vi "Main 1.0.vi"() -> ()   [LabVIEW 2014]
doc: "This template is for the Queued Message Handler design pattern.\n\nThe Event Handling Loop generates messages based on user interface actions.\n\nThe Message Handling Loop processes messages generated by the Event Handling Loop, or by other messages. The messages are string values, so new messages can be added easily to the Message Cases case structure in the Message Handling Loop. Each message cluster can also provide an optional value for Message Data, which is a variant that can be converted to whatever message-specific data is required."
uses:
  Loops.ctl
  Digital/Digital Input Cluster.ctl
  Digital/Digital Output Cluster.ctl
  Laser/Keyence Status.ctl
  Analog/Analog Output Cluster.ctl
  Analog/Analog Input Cluster.ctl
  Analog/Analog Result Cluster.ctl
  Engine/Thread Flag Control.ctl
  Engine/Message.ctl
  Analog/Enum AO.ctl
  Data Processor/Data Processor cluster.ctl
  Data Processor/I Adj Parameters.ctl
  Data Processor/UCTRL Cluster.ctl
  <vilib>/Utility/miscctls.llb/LVRectTypeDef.ctl
  <vilib>/Utility/miscctls.llb/LVPointTypeDef.ctl
  Engine/Thread.ctl
  Teszt/Teszt.ctl
  Teszt/Command.ctl
  Laser/Keyence data cluster.ctl
  support/Message Queue/Enqueue Message (Single).vi
  support/Message Queue/Enqueue Message (Array).vi
  global/Global 1.vi
  <vilib>/Utility/error.llb/Error Cluster From Error Code.vi
  <vilib>/ErrorRing/Error Ring.xnode
  support/Message Queue/Message Queue.lvlib
  support/User Event - Stop/User Event - Stop.lvlib
panel:
  out "Digitális Óra":timestamp format="%<%H:%M:%S\n%x>T"
  out "Termék":string
  in  "Tab Control":T1(tab)=enum."Etalon"
  out "Gyûrû megnyomva":bool caption="JÓ"
  out "Termék behelyezve":bool caption="JÓ"
  out "Gyûrû behelyezve":bool caption="JÓ"
  in  "Reset_Counters 2":bool
  out "Rossz db 2":i32 caption="Rossz db"
  out "Jó db 2":i32 caption="Jó db"
  out "Állapot kijelzõ ring":string
  out "Rossz 3":bool caption="Rossz"
  out "JÓ 3":bool caption="JÓ"
  out "dU görbe":T2
  in  "Eredmény Listbox":i32(listbox)
  out "Állapot kijelzõ fõképernyõ":string
  out "Rossz 2":bool caption="Rossz"
  out "JÓ 2":bool caption="JÓ"
  in  "Mérés stop 2":bool
  in  "Mérés start 2":bool
  in  "Reset_Counters":bool
  out "Rossz db":i32
  out "Jó db":i32
  out "Felhasználó":string
  out "Jogosultság":string
  in  "Termék választás":bool
  in  "Kilépés":bool
  in  "Felhasználó váltás":bool
  in  "Karbantartás":bool
  in  "Stop":bool
  in  "Végig mér":bool
  in  "Mérés Folyamatos":bool
  in  "Mérés stop":bool
  in  "Mérés következõ":bool
  out "Állapot kijelzõ 2":string
  out "Rossz":bool
  out "JÓ":bool
  in  "Mérés Listbox":i32(listbox)
  in  "Mérés start":bool
  in  "Thread 1":bool
  in  "Thread 0":bool
  out "Thread Num":enum16{"Mérés", "Gyûrûzés"}(ring)
  in  "Teszt eltávolít":bool
  out "Tesztszekvencia neve":string="Nincs betöltve..."
  in  "Teszt szerkeszt":bool
  in  "Teszt hozzáad":bool
  in  "Teszt töröl":bool
  in  "Teszt módosít":bool
  in  "Teszt vektor listbox":i32(listbox)
  in  "Teszt másol":bool
  in  "Teszt beilleszt":bool
  in  "Teszt megnyit":bool
  in  "Teszt ment":bool
  out "Thread Num 2":enum16{"Mérés", "Gyûrûzés"}(ring)
  in  "Etalon mérés":bool=TRUE
  in  "Teszt eltávolít 2":bool
  out "Tesztszekvencia neve 2":string="Nincs betöltve..."
  in  "Teszt szerkeszt 2":bool
  in  "Teszt hozzáad 2":bool
  in  "Teszt töröl 2":bool
  in  "Teszt módosít 2":bool
  in  "Etalon listbox":i32(listbox)
  in  "Teszt másol 2":bool
  in  "Teszt beilleszt 2":bool
  in  "Teszt megnyit 2":bool
  in  "Teszt ment 2":bool
  in  "Thread 0_2":bool
  in  "Thread 1_2":bool
  in  "Tab control debug":enum32{"Digital IO", "Analog IO", "Laser"}(tab)
  out "Digital input":T3
  in  "Digital Out":T4
  in  "Setup UCTRL NTC":bool
  out "NI Analog Input":T5 {"NI-6221"."Uref" format="%_5f"; "NI-6221"."Temperature" format="%_5f"; "NI-6221"."Uisol" format="%_5f"; "NI-6221"."U48" format="%_5f"; "NI-6221"."U15" format="%_5f"; "NI-6221"."NTC" format="%_5f"; "NI-6221"."Sensor" format="%_5f"; "Analog Result"."Számolt NTC hõmérséklet" format="%.3g"; "Analog Result"."15V" format="%.3g"; "Analog Result"."Elvárt NTC ellenállás" format="%.3g"; "Analog Result"."48V" format="%.3g"; "Analog Result"."Hõmérséklet" format="%.3g"; "Analog Result"."Szigetelési ellenállás" format="%.3g"; "Analog Result"."NTC ellenállás" format="%.3g"; "Analog Result"."Szenzor ellenállás" format="%.3g"}
  in  "NI Analog Output":T7
  out "UCTRL NTC":dbl
  out "UCTRL R":dbl
  out "UCTRL dU":dbl
  in  "Setup UCTRL R":bool
  in  "Keyence Disable":bool caption="Lézer jelölés tiltása"
  in  "Update Sys Time":bool
  out "Communication opened":bool
  in  "Start marking":bool
  out "Status":T8
  in  "Program change":bool
  in  "Error clear":bool
  in  "Keyence Open":bool
  in  "Program No":dbl
  in  "Termék cluster array":T9[](array[typedef])
  in  "Termék ment":bool
  out "Aktuális termék":T9
  in  "Felhasználók mentés":bool
  in  "Jogosultságok array":T10[](array[typedef])
  in  "Felhasználók Listbox":i32(listbox)
  in  "Új felhasználó":bool
  in  "Felhasználó törlése":bool
  in  "Felhasználó módosítás":bool
  out "Loops":T11
  out "Állapot kijelzõ":string
  # "Termék:"
  # "686 EOL Teszter"
  # "GYÛRÛZÉS"
  # "MÉRÉS"
  # "Menü"
  # "Bejelentkezve:"
  # "Jogosultság:"
  # "Menü"
  # "Keyence lézer jelölõ"
  # "Aktuális termék:"
  # "Termékek felvétele/beállítása:"
  # "Menü"
  # "Felhasználók"
  # "Jogosultságok"
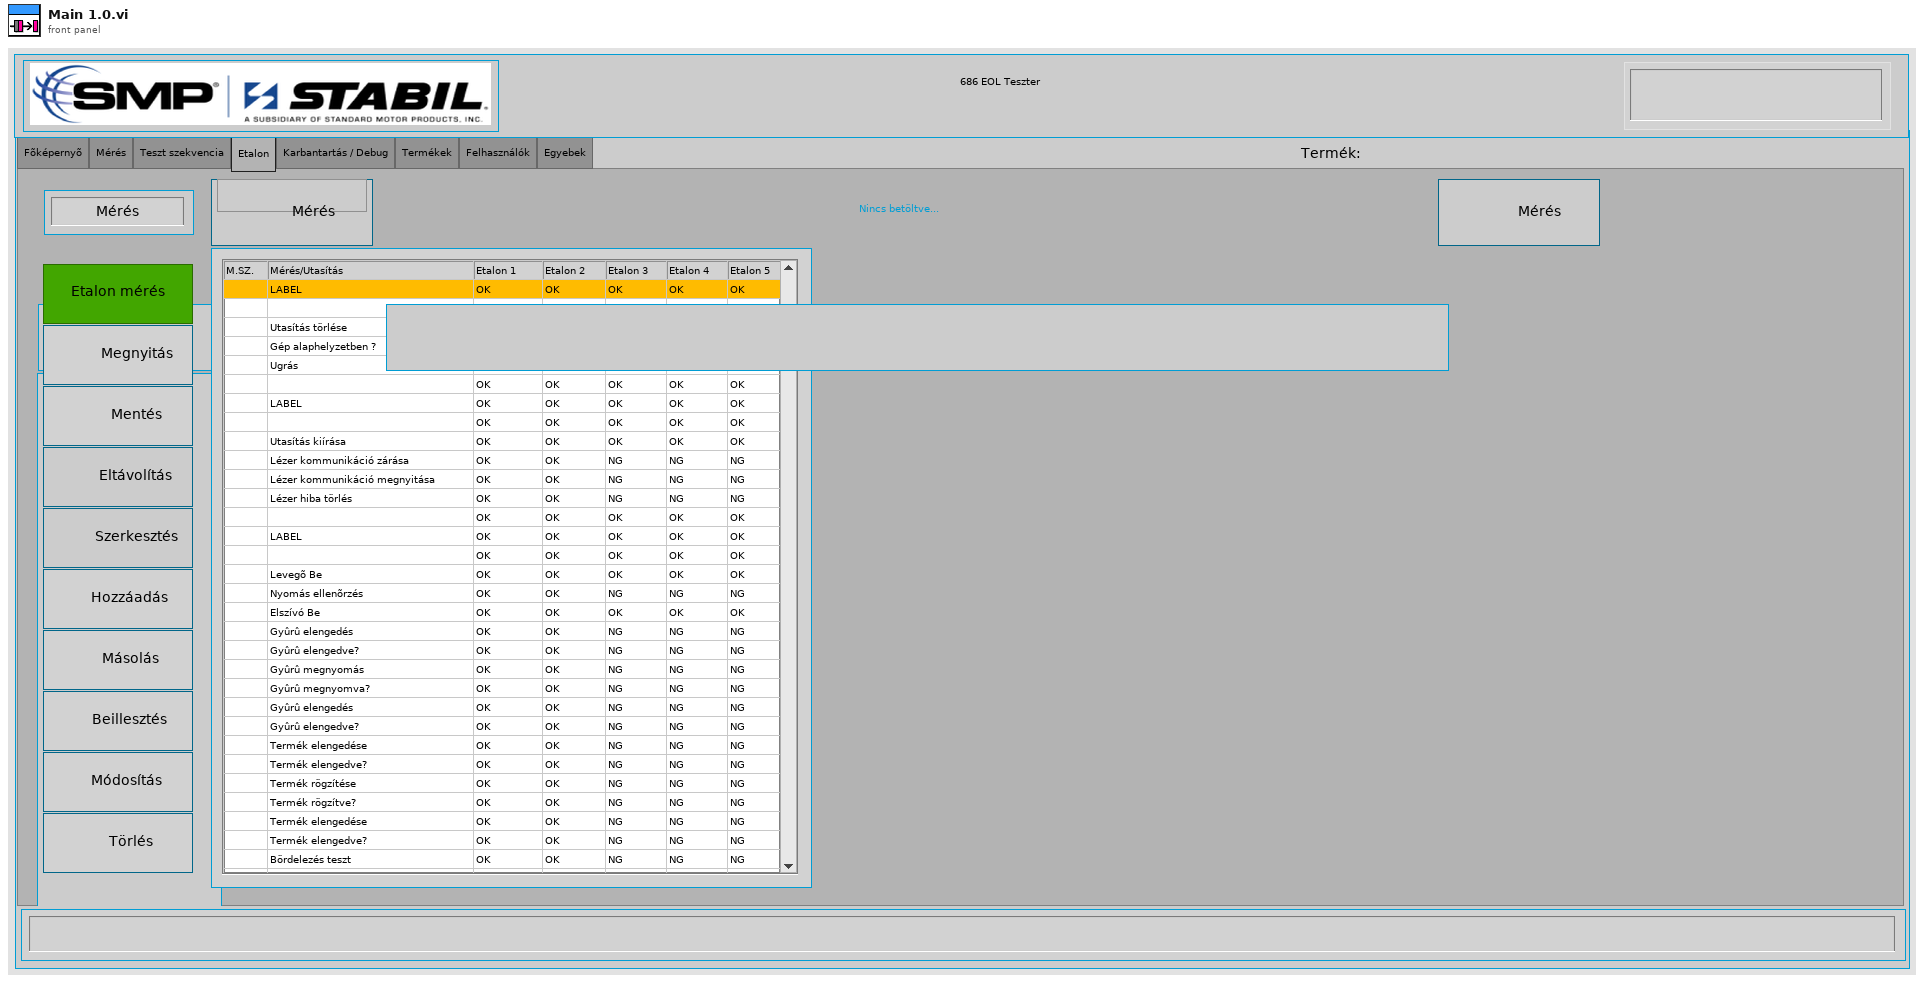
[diagram p1: front panel]
types:
  T1 = enum32{"Fõképernyõ", "Mérés", "Teszt szekvencia", "Etalon", "Karbantartás / Debug", "Termékek", "Felhasználók", "Egyebek"}
  T2 = typedef "dU görbe.ctl" = waveform(dbl)
  T3 = typedef "Digital Input Cluster.ctl" = cluster{"PCIE-6321 IN":cluster{"Termék bördelezve":bool, "Izolációs relék OK":bool, "Rézgyûrû a terméken":bool, "Termék rögzítve":bool, "Termék a gyûrûzõben":bool, "Rézgyûrû behelyezve":bool, "Rézgyûrû elengedve":bool, "Rézgyûrû megnyomva":bool, "Termék elengedve":bool, "Levegõ rendben":bool, "Termék jelen (táv)":bool, "Termék jelen (fém)":bool, "Selejt érzékelõ":bool}}
  T4 = typedef "Digital Output Cluster.ctl" = cluster{"PCIE-6321 OUT":cluster{"Izolációs relé":bool, "B oldal relé (nincs használva)":bool, "48V relé":bool, "Elszívás KI":bool, "Bördelezés teszt":bool, "Gyûrû megnyomás":bool, "Termék rögzítés":bool, "R mérés relé":bool, "200mA relé":bool, "NTC mérés relé":bool, "Levegõ BE":bool}}
  T5 = typedef "Analog Input Cluster.ctl" = cluster{"NI-6221":cluster{"Sensor":dbl, "Uref":dbl, "Temperature":dbl, "Uisol":dbl, "NTC":dbl, "U48":dbl, "U15":dbl}, "Analog Result":T6, "AI engedélyezés":bool, "dU":dbl[]}
  T6 = typedef "Analog Result Cluster.ctl" = cluster{"Szenzor ellenállás":dbl, "NTC ellenállás":dbl, "Szigetelési ellenállás":dbl, "Hõmérséklet":dbl, "48V":dbl, "15V":dbl, "Elvárt NTC ellenállás":dbl, "Számolt NTC hõmérséklet":dbl}
  T7 = typedef "Analog Output Cluster.ctl" = cluster{"NI-6221":cluster{"UCTRL":dbl}}
  T8 = typedef "Keyence Status.ctl" = cluster{"Ready":bool, "Error":bool, "Warning":bool, "Shutter":bool, "Mark Check OK":bool, "Mark Check NG":bool, "Marking Busy":bool, "Program No":u16, "Marking Check Busy":bool, "Marking Completed":bool, "Marking Score":u16, "Marking Error":bool, "Marking Stop":bool, "Program is changing":bool, "Date/Time":timestamp}
  T9 = typedef "Termék cluster.ctl" = cluster{"Termék név":string, "Teszt szekvencia":path, "Etalonok száma":i8}
  T10 = typedef "Tab jogosultság.ctl" = cluster{"Tab Name":string, "Operator":bool, "Karbantartó":bool, "QS":bool}
  T11 = typedef "Loops.ctl" = cluster{"Engine Stopped":bool, "Laser Stopped":bool, "Keyence Stopped":bool, "Data Processor Stopped":bool, "Timers Stopped":bool, "Timer mérés Stopped":bool, "Timer laser Stopped":bool, "DAQ  Stopped":bool, "NI Digital Stopped":bool, "NI Analog Stopped":bool, "Ring Stopped":bool}
  T12 = typedef "Message Queue.lvlib/All Message Queues.ctl" = cluster{"UI":refnum<queue>, "Engine":refnum<queue>, "Laser":refnum<queue>, "Keyence":refnum<queue>, "Data Processor":refnum<queue>, "Timers":refnum<queue>, "Timer mérés":refnum<queue>, "Timer laser":refnum<queue>, "DAQ":refnum<queue>, "NI Digital":refnum<queue>, "DI data":refnum<queue>, "DO data":refnum<queue>, "Data Processor data":refnum<queue>, "Keyence Data":refnum<queue>, "Ring":refnum<queue>, "NI Analog":refnum<queue>, "AI data":refnum<queue>, "AO data":refnum<queue>, "Analog UI Data":refnum<queue>}
  T13 = typedef "LVPointTypeDef.ctl" = cluster{"Horizontal":i16, "Vertical":i16}
  T14 = typedef "LVRectTypeDef.ctl" = cluster{"Left":i16, "Top":i16, "Right":i16, "Bottom":i16}
  T15 = cluster{"Thread Num":enum16{"Mérés", "Gyûrûzés"}, "Elérési út":path}
  T16 = typedef "Thread.ctl" = cluster{"Run":bool, "Pause":bool, "Step Execution":bool, "Ignore Error":bool, "File name":string, "Program":T17[], "Program PTR":u32, "Current Test":T17, "Error":errorcluster, "Previous Test":T17, "Etalon number":u32, "Etalon error code":u32, "Meas Result":bool, "Etalon Result":bool, "Aborted":bool, "Alaphelyzet":bool, "Command":string, "Response":string}
  T17 = typedef "Teszt.ctl" = cluster{"Thread ID":dbl, "Mérésszám":string, "Mérés/Utasítás":string, "Command":T18, "Min":string, "Max":string, "Aktív?":bool, "Log?":bool, "Kiértékelés":bool, "Etalon 1 exp":bool, "Etalon 2 exp":bool, "Etalon 3 exp":bool, "Etalon 4 exp":bool, "Etalon 5 exp":bool}
  T18 = typedef "Command.ctl" = cluster{"Parancs":string, "Paraméter 1":string, "Paraméter 2":string, "Paraméter 3":string, "Paraméter 4":string, "Paraméter 5":string, "Eredmény":string}
  T19 = typedef "Felhasználó típus.ctl" = cluster{"NÉV:":string, "Jelszó: (csak számjegyek)":string, "Felhasználói szint":string}
  T20 = cluster{"Jó":bool, "Rossz":bool, "Jó db":i32, "Rossz db":i32}
  T21 = enum8{"Enabled", "Disabled", "Disabled and Grayed Out"}
  T22 = typedef "Fõképernyõ references.ctl" = cluster{"Felhasználó váltás":refnum<vi>, "Kilépés":refnum<vi>, "Termék választás":refnum<vi>, "Karbantartás":refnum<vi>, "Stop":refnum<vi>, "Tab control":refnum<vi>, "Tab control debug":refnum<vi>, "Mérés start":refnum<vi>, "Mérés start 2":refnum<vi>, "Mérés következõ":refnum<vi>, "Mérés stop":refnum<vi>, "Mérés stop 2":refnum<vi>, "Mérés folyamatos":refnum<vi>, "Végig mér":refnum<vi>, "Mérés listbox":refnum<vi>, "Teszt vektor listbox":refnum<vi>, "Etalon listbox":refnum<vi>, "Eredmény listbox":refnum<vi>}
  T23 = typedef "Thread Flag Control.ctl" = cluster{"Thread ID":u16, "Thread Flag":bool}
  T24 = typedef "Message.ctl" = cluster{"Thread ID":u16, "Callback":string, "Data":variant, "Error":errorcluster}
  T25 = cluster{"ItemNames[0]":string, "ItemNames[1]":string, "ItemNames[2]":string}
  T26 = typedef "Keyence data cluster.ctl" = cluster{"Communication Opened":bool, "Status":T8, "IP Address":string, "Laser Disabled":bool}
  T27 = typedef "Data Processor cluster.ctl" = cluster{"Dummy":bool, "R Res":dbl, "NTC Res":dbl, "Insulation Res":dbl, "Temperature":dbl, "NTC Exp Res":dbl, "NTC Calc Temp":dbl, "Delta U Puffer":refnum<queue>, "I Adj Parameters":T28, "UCTRL Cluster":T29}
  T28 = typedef "I Adj Parameters.ctl" = cluster{"Vr NTC":dbl, "Vr R":dbl, "Vr dU":dbl, "I Adj step":i32, "Output":dbl, "Adj Failed":bool}
  T29 = typedef "UCTRL Cluster.ctl" = cluster{"UCTRL NTC":dbl, "UCTRL R":dbl, "UCTRL dU":dbl}
  T30 = typedef "Enum AO.ctl" = enum16{"UCTRL"}
  T31 = enum32{"Page Enabled", "Page Disabled", "Page Disabled & Grayed"}
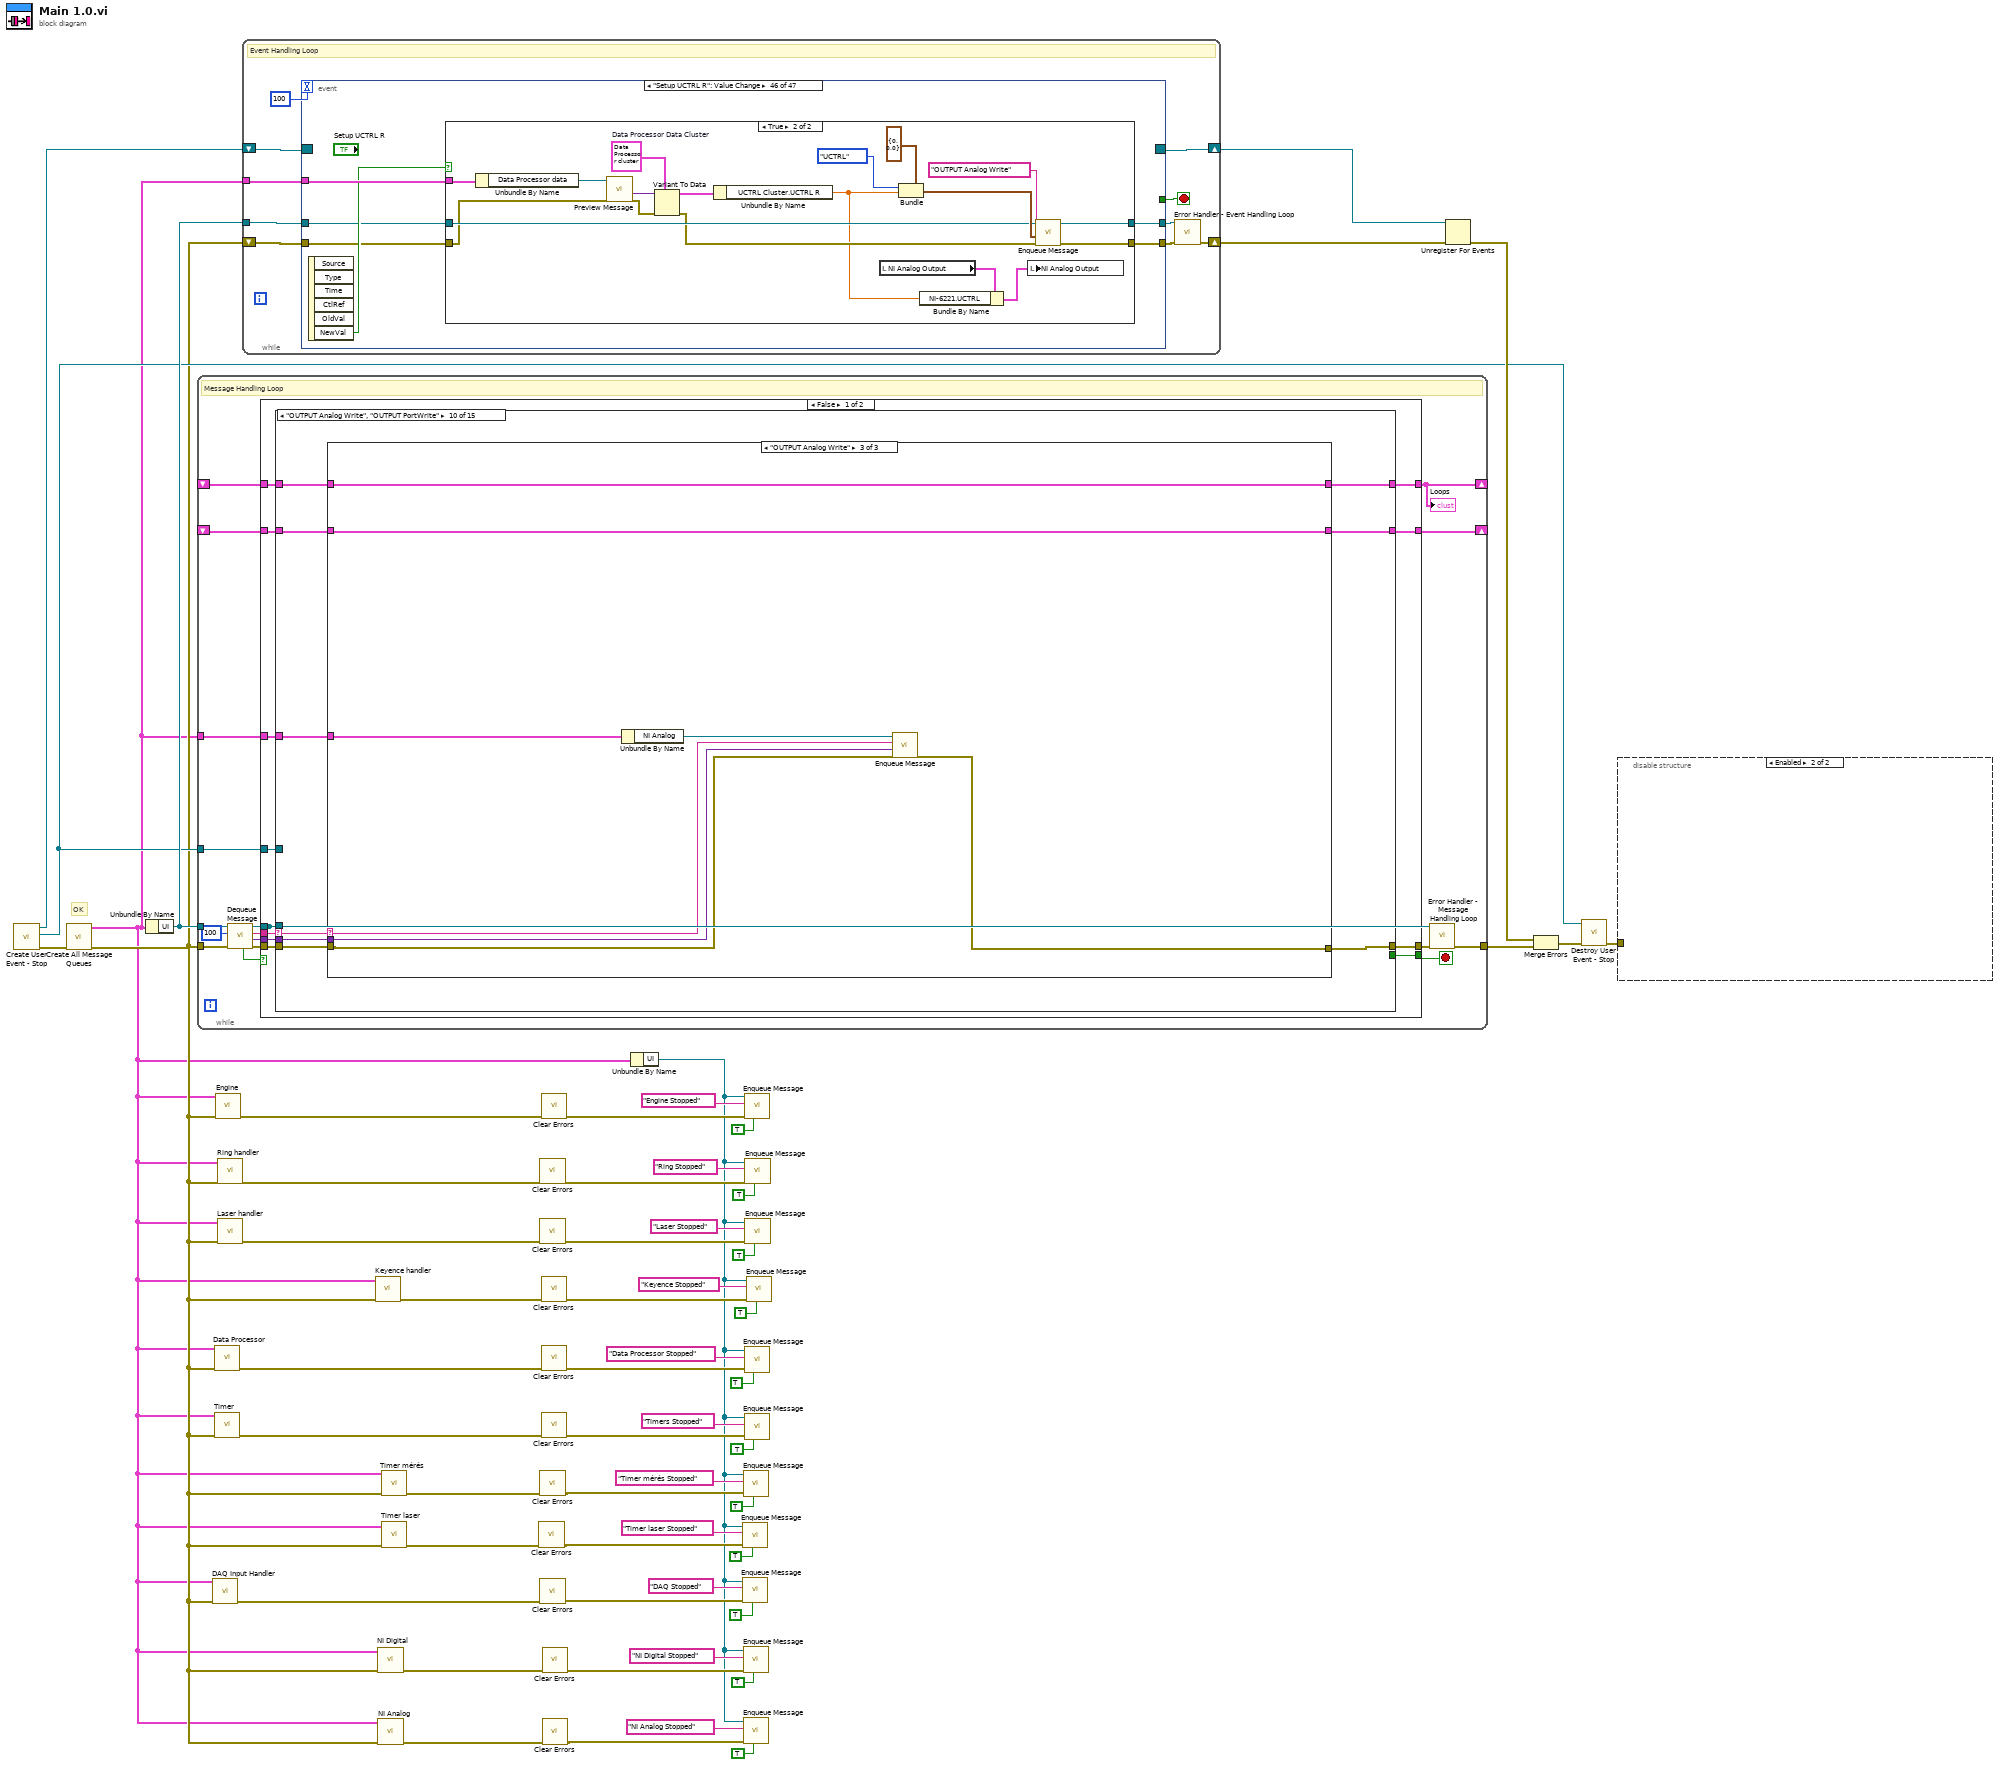
[diagram p0: block diagram]
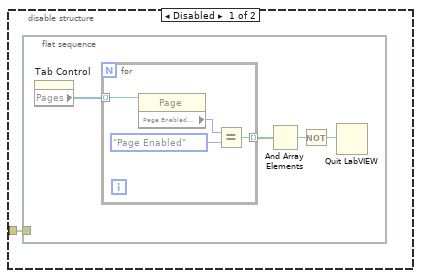
[diagram p2: hidden frame]
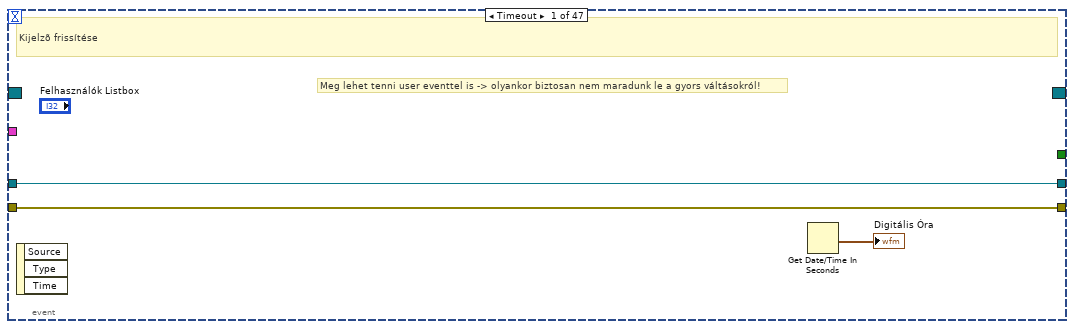
[diagram p3: hidden frame]
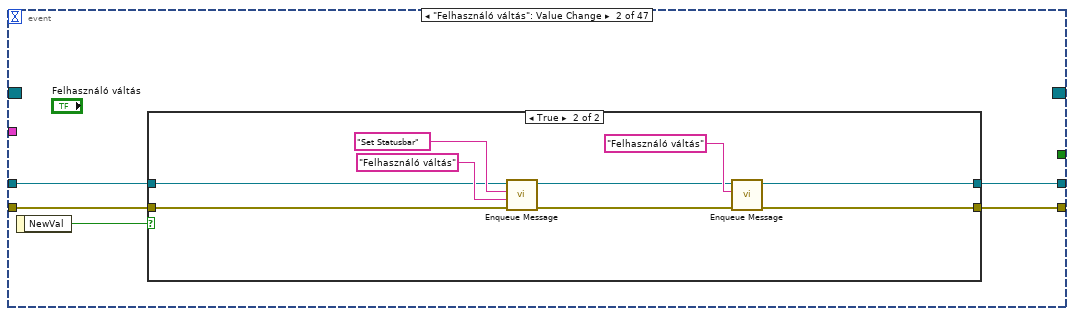
[diagram p4: hidden frame]
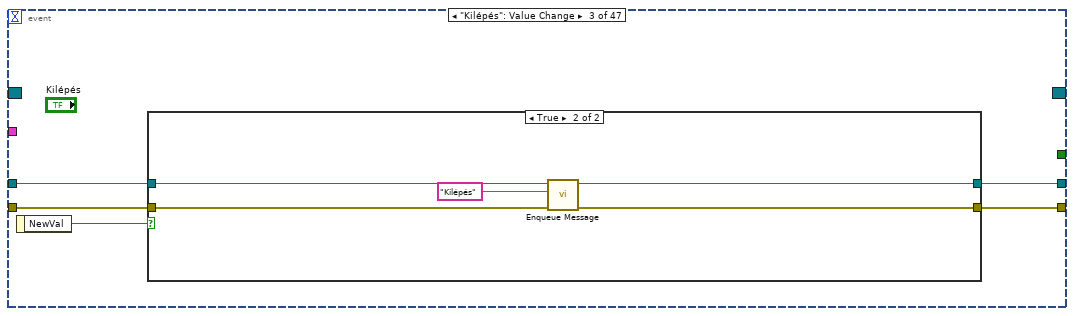
[diagram p6: hidden frame]
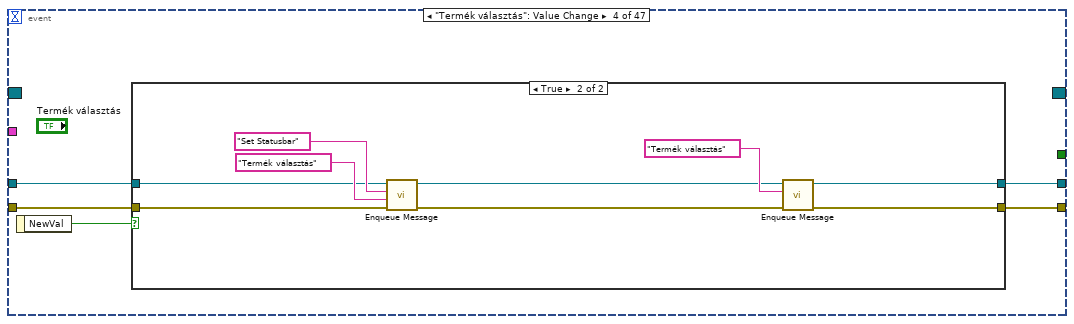
[diagram p8: hidden frame]
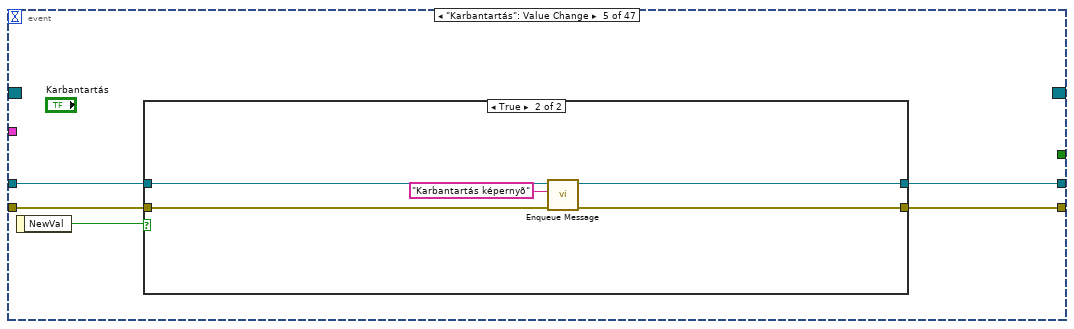
[diagram p10: hidden frame]
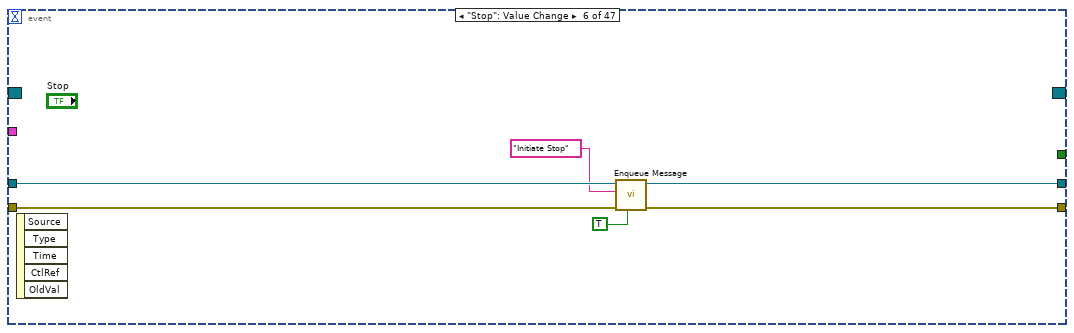
[diagram p12: hidden frame]
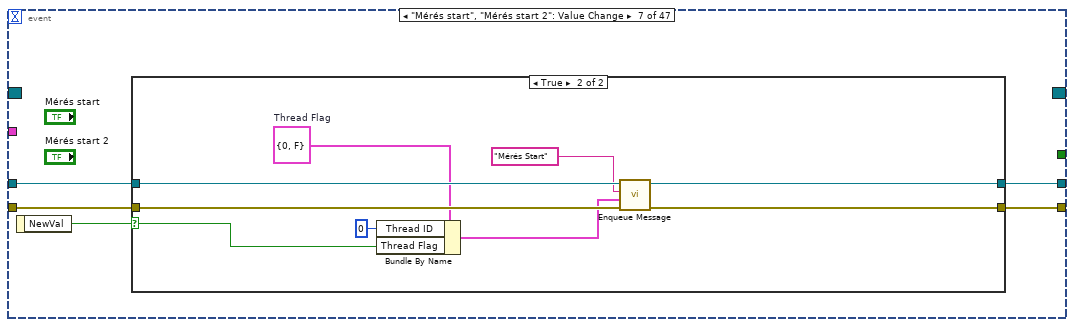
[diagram p13: hidden frame]
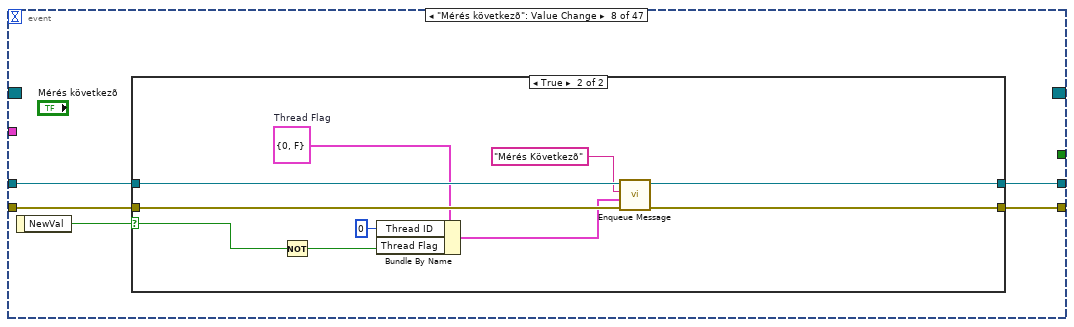
[diagram p15: hidden frame]
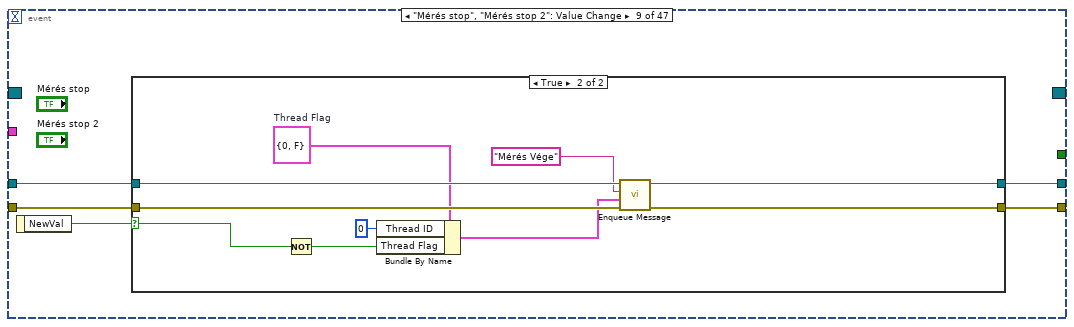
[diagram p17: hidden frame]
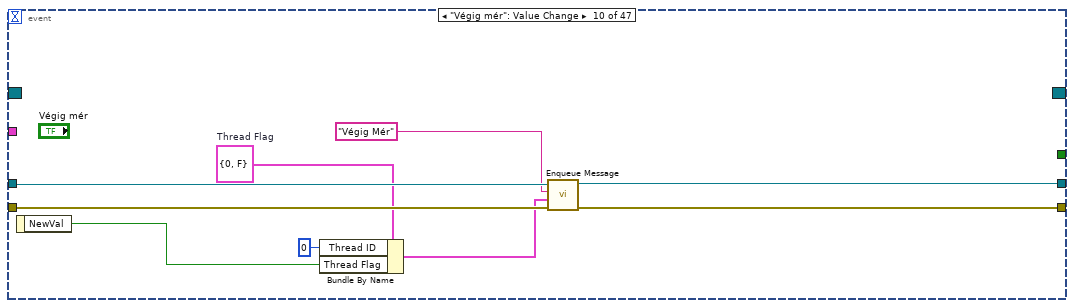
[diagram p19: hidden frame]
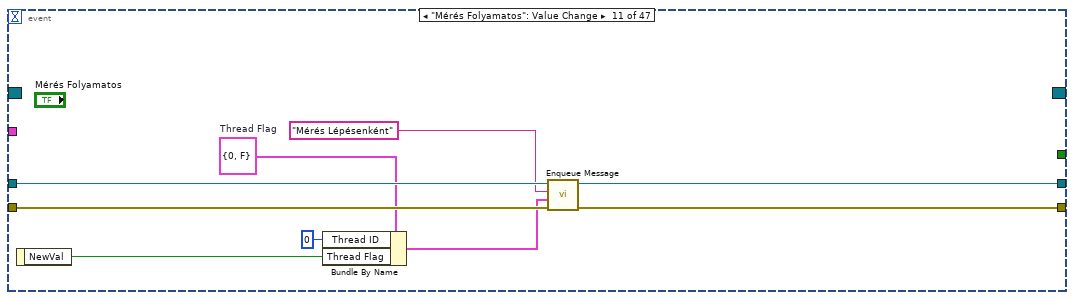
[diagram p20: hidden frame]
diagram:
  # "OK"
  n1 = call "Create User Event - Stop.vi"() -> ("error out"=w56:errorcluster, "User Event - Stop"=w13:refnum<user-event>, "Stop Event Registration Refnum"=w12:refnum<event-registration>)  [unwired: 9 in]
  n2 = call "Create All Message Queues.vi"("error in (no error)"=w56) -> ("error out"=w3:errorcluster, "Message Queues out"=w1:T12)  [unwired: 9 in]
  n3 = Unbundle By Name(w1) -> ("UI"=w50:refnum<queue>)
  n4 = while {
    tunnel: w50 -> [w68]
    tunnel: w13 -> [w73]
    tunnel: w3 -> [w72]
    tunnel: [w66] -> w57
    shift-right: [w64] -> _
    shift-left: _ -> [w63]
    tunnel: w1 -> [w62]
    shift-right: [w60] -> _
    shift-left: _ -> [w61]
    stop <- w74 stop-if-true
    # "Message Handling Loop"
    n5 = call "Dequeue Message.vi"("error in (no error)"=w72, "timeout in ms (-1)"=100, "Message Queue"=w68) -> ("error out"=w71:errorcluster, "Message Data"=w69:variant, "Message"=w70:string, "dup Message Queue"=w67:refnum<queue>, "timed out?"=w59:bool)  [unwired: 4 in]
    n6 = case shown="False" w59 {
      tunnel: [w86 FALSE] -> w74
      tunnel: w73 -> [w85 _]
      tunnel: w71 -> [w84 w1498]
      tunnel: w70 -> [w83 _]
      tunnel: w69 -> [w82 _]
      tunnel: w67 -> [w81 _]
      tunnel: [w80 w1500] -> w65
      tunnel: [w79 w1512] -> w64
      tunnel: w63 -> [w78 w1512]
      tunnel: w62 -> [w77 w1506]
      tunnel: w61 -> [w76 w1513]
      tunnel: [w75 w1513] -> w60
      frame False {
        n7 = case "Message Cases" shown="\"OUTPUT Analog Write\", \"OUTPUT PortWrite\"" w83 {
          selector: w83 -> [w97 w176 w316 w475 w533 w747 w771 w866 _ w1061 w1092 w1103 w1394 _ w1486]
          tunnel: w81 -> [w96 w177 w317 w474 w532 w746 w770 w865 _ _ _ w1102 w1398 w1476 _]
          tunnel: w84 -> [w95 w178 w318 w473 w531 w745 w768 w864 w991 w1065 w1091 w1101 w1400 w1477 _]
          tunnel: [w89 w181 w321 w467 w525 w739 w763 w858 w992 w1062 w1087 w1095 w1397 w1472 w1487] -> w80
          tunnel: [_ _ w313 _ _ _ _ _ _ _ _ _ _ _ _] -> w86
          tunnel: w82 -> [w94 w173 w312 w472 w530 w744 w769 w863 _ w1064 w1090 w1100 w1399 _ _]
          tunnel: w85 -> [w92 w174 w314 w470 w528 w742 w767 w861 _ _ _ w1098 _ _ _]
          tunnel: [w90 w179 w319 w468 w526 w740 w764 w859 w1005 w1057 w1088 w1096 w1392 w1470 w1485] -> w79
          tunnel: w78 -> [w91 w180 w320 w469 w527 w741 w765 w860 w1005 w1058 w1088 w1097 w1393 w1470 w1485]
          tunnel: w77 -> [w93 w175 w315 w471 w529 w743 w766 w862 w999 w1063 w1089 w1099 _ _ _]
          tunnel: w76 -> [w87 w171 w311 w465 w524 w737 w761 w856 w1004 w1060 w1086 w1093 w1396 w1469 w1484]
          tunnel: [w88 w172 w310 w466 w523 w738 w762 w857 w1004 w1059 w1086 w1094 w1395 w1469 w1484] -> w75
          frame "Initialize", "Initialize Data", "Initialize UI" {
            n8 = case shown="\"Initialize Data\"" w97 {
              tunnel: w96 -> [w103 _ _ _]
              tunnel: w95 -> [w102 w145 w146 w169]
              tunnel: w94 -> [_ _ _ _]
              tunnel: w93 -> [_ _ w157 _]
              tunnel: w92 -> [_ _ _ _]
              tunnel: w91 -> [w110 _ w160 w170]
              tunnel: [w110 w135 w162 w170] -> w90
              tunnel: [w108 w116 w159 w169] -> w89
              tunnel: [w99 w144 w161 w168] -> w88
              tunnel: w87 -> [_ w144 w161 w168]
              frame "Initialize" {
                w99 = T11 {"Engine Stopped"=FALSE, "Laser Stopped"=FALSE, "Keyence Stopped"=FALSE, "Data Processor Stopped"=FALSE, "Timers Stopped"=FALSE, "Timer mérés Stopped"=FALSE, "Timer laser Stopped"=FALSE, "DAQ  Stopped"=FALSE, "NI Digital Stopped"=FALSE, "NI Analog Stopped"=FALSE, "Ring Stopped"=FALSE}  # Loops
                # "Reinit values default"
                n9 = case shown="True" TRUE {
                  tunnel: w102 -> [w111 w113]
                  tunnel: [w111 w112] -> w105
                  frame False {
                  }
                  frame True {
                    # "50 ->hogy látszódjon a title bar"
                    # "Origó"
                    # "Fullscreen"
                    n10 = property class="VI"(error in=w113, "Front Panel.PanelBounds"=T14 {"Left"=0, "Top"=50, "Right"=1920, "Bottom"=1030} ("Front Panel Window:Panel Bounds")) -> (error out=w112:errorcluster)  [unwired: 1 in, 1 out]
                    n11 = property on="Pane" class="Pane"("Origin"=T13 {"Horizontal"=0, "Vertical"=0}) -> ()  [unwired: 2 in, 2 out]
                  }
                }
                n12 = control-ref of="This VI"() -> (w106:refnum<vi>)
                n13 = invoke class="VI" method="Default Vals.Reinit All"(reference=w106, error in=w105) -> (reference out=w107:refnum<vi>, error out=w104:errorcluster)  [unwired: 1 in, 1 out]
                n14 = Close Reference(reference=w107, error in (no error)=w104) -> (error out=w98:errorcluster)
                n15 = call-poly "Enqueue Message.vi"("error in (no error)"=w102, "Message Array"=string[] ["Initialize Data", "Initialize UI"], "Message Queue"=w103) -> ("error out"=w101:errorcluster)  [unwired: 7 in, 1 out]
                n16 = Merge Errors(w98, w101) -> (w108:errorcluster)
              }
              frame "Initialize Data" {
                w137 = enum16{"Mérés", "Gyûrûzés"}."Mérés" ("Thread Num")
                w136 = T22 {"Felhasználó váltás"=refnum, "Kilépés"=refnum, "Termék választás"=refnum, "Karbantartás"=refnum, "Stop"=refnum, "Tab control"=refnum, "Tab control debug"=refnum, "Mérés start"=refnum, "Mérés start 2"=refnum, "Mérés következõ"=refnum, "Mérés stop"=refnum, "Mérés stop 2"=refnum, "Mérés folyamatos"=refnum, "Végig mér"=refnum, "Mérés listbox"=refnum, "Teszt vektor listbox"=refnum, "Etalon listbox"=refnum, "Eredmény listbox"=refnum}  # Fõképernyõ references
                n17 = call "Megnyitás.vi"("error in"=w145) -> ("error out"=w142:errorcluster, "Felhasználói adatok out"=w143:string[][])  [unwired: 9 in]
                n18 = control-ref of="Mérés Listbox"() -> (w120:refnum<vi>)
                n19 = control-ref of="Teszt vektor listbox"() -> (w119:refnum<vi>)
                n20 = control-ref of="Etalon listbox"() -> (w118:refnum<vi>)
                n21 = control-ref of="Eredmény Listbox"() -> (w117:refnum<vi>)
                n22 = control-ref of="Tab Control"() -> (w129:refnum<vi>)
                n23 = control-ref of="Tab control debug"() -> (w128:refnum<vi>)
                n24 = control-ref of="Felhasználó váltás"() -> (w134:refnum<vi>)
                n25 = control-ref of="Kilépés"() -> (w133:refnum<vi>)
                n26 = control-ref of="Termék választás"() -> (w132:refnum<vi>)
                n27 = control-ref of="Karbantartás"() -> (w131:refnum<vi>)
                n28 = control-ref of="Stop"() -> (w130:refnum<vi>)
                n29 = control-ref of="Mérés start"() -> (w127:refnum<vi>)
                n30 = control-ref of="Mérés start 2"() -> (w126:refnum<vi>)
                n31 = control-ref of="Mérés következõ"() -> (w125:refnum<vi>)
                n32 = control-ref of="Mérés stop"() -> (w124:refnum<vi>)
                n33 = control-ref of="Mérés stop 2"() -> (w123:refnum<vi>)
                n34 = control-ref of="Mérés Folyamatos"() -> (w122:refnum<vi>)
                n35 = control-ref of="Végig mér"() -> (w121:refnum<vi>)
                n36 = property on="Felhasználók Listbox" class="MCListbox (strict)"(error in=w142, "ItemNames"=w143) -> (error out=w141:errorcluster)  [unwired: 1 in, 1 out]
                n37 = Bundle By Name(cluster=w136, "Felhasználó váltás"=w134, "Kilépés"=w133, "Termék választás"=w132, "Karbantartás"=w131, "Stop"=w130, "Tab control"=w129, "Tab control debug"=w128, "Mérés start"=w127, "Mérés start 2"=w126, "Mérés következõ"=w125, "Mérés stop"=w124, "Mérés stop 2"=w123, "Mérés folyamatos"=w122, "Végig mér"=w121, "Mérés listbox"=w120, "Teszt vektor listbox"=w119, "Etalon listbox"=w118, "Eredmény listbox"=w117) -> (w135:T22)
                n38 = call "Termék megnyitás.vi"("error in"=w141) -> ("error out"=w139:errorcluster, "Termék cluster array"=w140:T9[])  [unwired: 8 in, 1 out]
                n39 = local write "Termék cluster array"(w140) -> ()
                n40 = call "Jogosultságok megnyitás.vi"("error in"=w139, "UI Data"=w135) -> ("error out"=w116:errorcluster, "Jogosultsági adatok out"=w138:T10[])  [unwired: 8 in]
                n41 = local write "Jogosultságok array"(w138) -> ()
                "Thread Num" <- w137
                "Thread Num 2" <- w137
              }
              frame "Initialize UI" {
                # "KÉSZ"
                n42 = Unbundle By Name(w160) -> ("Eredmény listbox"=w147:refnum<vi>, "Etalon listbox"=w151:refnum<vi>, "Teszt vektor listbox"=w152:refnum<vi>, "Mérés listbox"=w153:refnum<vi>)
                n43 = call "Fõképernyõ UI engedélyezés.vi"("Error In"=w146, "Felhasználói szint"="", "UI Data"=w160) -> ("Error Out"=w166:errorcluster, "Felhasználói szint ki"=w163:string, "UI Data out"=w165:T22)  [unwired: 6 in]
                n44 = Unbundle By Name(w157) -> ("Engine"=w156:refnum<queue>)
                n45 = call "Mérésképernyõ UI engedélyezés.vi"("Error In"=w166, "Felhasználói szint"=w163, "UI Data"=w165) -> ("Error Out"=w164:errorcluster, "UI Data out"=w162:T22)  [unwired: 7 in]
                n46 = call "Init listbox.vi"("error in (no error)"=w146, "MulticolumnListbox in"=w153) -> ("error out"=w154:errorcluster)  [unwired: 9 in]
                n47 = call "Init listbox.vi"("error in (no error)"=w154, "MulticolumnListbox in"=w152) -> ("error out"=w150:errorcluster)  [unwired: 9 in]
                n48 = call "Init listbox.vi"("error in (no error)"=w150, "MulticolumnListbox in"=w151) -> ("error out"=w149:errorcluster)  [unwired: 9 in]
                n49 = call "Init listbox.vi"("error in (no error)"=w149, "MulticolumnListbox in"=w147) -> ("error out"=w148:errorcluster)  [unwired: 9 in]
                n50 = Merge Errors(w164, w148) -> (w158:errorcluster)
                n51 = call-poly "Enqueue Message.vi"("error in (no error)"=w158, "Message"="UI Initialized", "Message Queue"=w156) -> ("error out"=w159:errorcluster)  [unwired: 7 in, 1 out]
              }
              frame Default {
                # "KÉSZ"
              }
            }
          }
          frame "Felhasználó váltás", "Initiate Stop", "Karbantartás képernyõ", "Kilépés", "Termék választás" {
            n52 = case shown="\"Felhasználó váltás\"" w176 {
              tunnel: [w199 w219 w229 w264 w290 w308] -> w181
              tunnel: w180 -> [w193 w220 w233 w268 w300 w309]
              tunnel: [w192 w210 w233 w268 w300 w309] -> w179
              tunnel: w178 -> [w189 w215 w228 w269 w295 w308]
              tunnel: w177 -> [w184 w213 w227 _ w297 _]
              tunnel: w175 -> [_ _ w224 _ w293 _]
              tunnel: w174 -> [_ _ _ _ _ _]
              tunnel: w173 -> [_ _ _ _ _ _]
              tunnel: [w188 w217 w225 w267 w292 w307] -> w172
              tunnel: w171 -> [w188 w217 w225 w267 w292 w307]
              frame "Felhasználó váltás" {
                # "KÉSZ"
                n53 = property on="Felhasználók Listbox" class="MCListbox (strict)"(error in=w189) -> (error out=w195:errorcluster, "ItemNames"=w196:string[][])  [unwired: 1 in, 1 out]
                n54 = call "Bejelentkezés.vi"("Error In"=w195, "Message Queue"=w184, "Felhasználói adatok in"=w196) -> ("Error Out"=w183:errorcluster, "OK ?"=w194:bool, "Felhasználó ki"=w182:T19)  [unwired: 6 in]
                n55 = case shown="True" w194 {
                  tunnel: w182 -> [_ w208]
                  tunnel: w193 -> [w201 w207]
                  tunnel: [w201 w203] -> w192
                  tunnel: w189 -> [w200 w206]
                  tunnel: [w200 w202] -> w191
                  frame False {
                  }
                  frame True {
                    n56 = local read "Jogosultságok array"() -> (w204:T10[])
                    n57 = Unbundle By Name(w208) -> ("Felhasználói szint"=w205:string)
                    n58 = call "Fõképernyõ UI engedélyezés.vi"("Error In"=w206, "Jogosultságok array"=w204, "Felhasználói szint"=w205, "UI Data"=w207) -> ("Error Out"=w202:errorcluster, "UI Data out"=w203:T22)  [unwired: 5 in, 1 out]
                  }
                }
                n59 = call-poly "Enqueue Message.vi"("error in (no error)"=w183, "Message Data"=w182, "Message"="Set User", "Message Queue"=w184) -> ("error out"=w186:errorcluster, "dup Message Queue"=w185:refnum<queue>)  [unwired: 6 in]
                n60 = call-poly "Enqueue Message.vi"("error in (no error)"=w186, "Message Data"="", "Message"="Set Statusbar", "Message Queue"=w185) -> ("error out"=w198:errorcluster)  [unwired: 6 in, 1 out]
                n61 = Merge Errors(w191, w198) -> (w199:errorcluster)
              }
              frame "Kilépés" {
                w211 = T19 {"NÉV:"="", "Jelszó: (csak számjegyek)"="", "Felhasználói szint"=""}  # Felhasználói adatok in
                # "KÉSZ"
                n62 = call "Fõképernyõ UI engedélyezés.vi"("Error In"=w215, "Felhasználói szint"="", "UI Data"=w220) -> ("Error Out"=w209:errorcluster, "UI Data out"=w210:T22)  [unwired: 6 in, 1 out]
                n63 = call-poly "Enqueue Message.vi"("error in (no error)"=w215, "Message Data"=w211, "Message"="Set User", "Message Queue"=w213) -> ("error out"=w214:errorcluster, "dup Message Queue"=w212:refnum<queue>)  [unwired: 6 in]
                n64 = call-poly "Enqueue Message.vi"("error in (no error)"=w214, "Message Data"="", "Message"="Set Statusbar", "Message Queue"=w212) -> ("error out"=w223:errorcluster)  [unwired: 6 in, 1 out]
                n65 = Merge Errors(w209, w223) -> (w219:errorcluster)
              }
              frame "Termék választás" {
                # "KÉSZ"
                n66 = call "Termék választás.vi"("error in"=w228, "Termék cluster array"="Termék cluster array") -> ("error out"=w226:errorcluster, "Kiválasztott termék"=w231:T9, "OK"=w230:bool)  [unwired: 6 in, 1 out]
                n67 = case shown="True" w230 {
                  tunnel: w231 -> [_ w247]
                  tunnel: w227 -> [w234 w241]
                  tunnel: w226 -> [w235 w255]
                  tunnel: [w236 w246] -> w229
                  tunnel: w224 -> [_ w251]
                  frame False {
                    n68 = call-poly "Enqueue Message.vi"("error in (no error)"=w235, "Message Data"="", "Message"="Set Statusbar", "Message Queue"=w234) -> ("error out"=w236:errorcluster)  [unwired: 6 in, 1 out]
                  }
                  frame True {
                    n69 = Unbundle By Name(w251) -> ("Engine"=w250:refnum<queue>)
                    n70 = Unbundle By Name(w247) -> ("Termék név"=→"Termék":string)
                    n71 = Unbundle By Name(w247) -> ("Teszt szekvencia"=w242:path)
                    n72 = call-poly "Enqueue Message.vi"("error in (no error)"=w255, "Message Data"=w247, "Message"="Set Product Variables", "Message Queue"=w250) -> ("error out"=w252:errorcluster, "dup Message Queue"=w249:refnum<queue>)  [unwired: 6 in]
                    n73 = local read "Etalon mérés"() -> (w253:bool)
                    n74 = Bundle By Name(cluster=T15 {"Thread Num"=enum."Mérés", "Elérési út"=path ""}, "Thread Num"=enum16{"Mérés", "Gyûrûzés"}."Mérés", "Elérési út"=w242) -> (w243:T15)
                    n75 = case shown="True" w253 {
                      tunnel: w252 -> [w259 w263]
                      tunnel: [w258 w262] -> w240
                      tunnel: w249 -> [w256 w260]
                      frame True {
                        n76 = call-poly "Enqueue Message.vi"("error in (no error)"=w259, "Message"="Set Etalon", "Message Queue"=w256) -> ("error out"=w258:errorcluster)  [unwired: 7 in, 1 out]
                      }
                      frame False {
                        n77 = call-poly "Enqueue Message.vi"("error in (no error)"=w263, "Message"="Reset Etalon", "Message Queue"=w260) -> ("error out"=w262:errorcluster)  [unwired: 7 in, 1 out]
                      }
                    }
                    n78 = call-poly "Enqueue Message.vi"("error in (no error)"=w240, "Message Data"=w243, "Message"="Tesztszekvencia megnyitása", "Message Queue"=w241) -> ("error out"=w246:errorcluster)  [unwired: 6 in, 1 out]
                    "Aktuális termék" <- w247
                  }
                }
              }
              frame "Karbantartás képernyõ" {
                # "KÉSZ"
                n79 = Unbundle By Name(w268) -> ("Tab control"=w285:refnum<vi>)
                n80 = Unbundle By Name(w268) -> ("Tab control debug"=w276:refnum<vi>)
                n81 = property class="TabCtl"(reference=w285, error in=w269, "Value"=4 ("index")) -> (error out=w280:errorcluster, "Pages"=w279:refnum<vi>[])  [unwired: 1 out]
                n82 = property class="TabCtl"(reference=w276, error in=w269, "Value"=0 ("index")) -> (error out=w273:errorcluster, "Pages"=w274:refnum<vi>[])  [unwired: 1 out]
                n83 = Index Array(array=w279, index #1=0 ("index"), index #2=4 ("index")) -> (element #1=w283:refnum<vi>, element #2=w284:refnum<vi>)
                n84 = property class="Page"(reference=w284, error in=w280, "FG Color"=u32 13816530) -> (error out=w271:errorcluster)  [unwired: 1 out]
                n85 = property class="Page"(reference=w283, error in=w280, "FG Color"=u32 12369084) -> (error out=w270:errorcluster)  [unwired: 1 out]
                n86 = for {
                  shift-right: [w289] -> w272
                  shift-left: w273 -> [w288]
                  tunnel: u32[] [13816530, 12369084, 12369084, 12369084, 12369084, 12369084, 12369084] -> [w287] mode=indexing
                  tunnel: w274 -> [w286] mode=indexing
                  n87 = property class="Page"(reference=w286, error in=w288, "FG Color"=w287) -> (error out=w289:errorcluster)  [unwired: 1 out]
                }
                n88 = Merge Errors(w270, w271, w272) -> (w264:errorcluster)
              }
              frame "Initiate Stop" {
                n89 = disable-structure shown="Disabled" {
                  disable-tunnel: w297 -> [w304 w306]
                  disable-tunnel: [w303 w306] -> w296
                  disable-tunnel: w295 -> [w302 w305]
                  disable-tunnel: [w301 w305] -> w294
                  frame Disabled {
                    n90 = Flush Queue(queue=w304, error in (no error)=w302) -> (queue out=w303:refnum<queue>, error out=w301:errorcluster)  [unwired: 1 out]
                  }
                  frame Enabled {
                  }
                }
                n91 = call-poly "Enqueue Message.vi"("error in (no error)"=w294, "Message Data"="Program leállítása..." ("Message"), "Message"="Set Statusbar", "Message Queue"=w296) -> ("error out"=w291:errorcluster)  [unwired: 6 in, 1 out]
                n92 = call "Initiate Stop.vi"("error in (no error)"=w291, "Loops"=w292, "Message Queues in"=w293) -> ("error out"=w290:errorcluster)  [unwired: 6 in]
              }
              frame Default {
                # "KÉSZ"
              }
            }
          }
          frame "All Stopped?", "DAQ Stopped", "Data Processor Stopped", "Engine Stopped", "Keyence Stopped", "Laser Stopped", "NI Analog Stopped", "NI Digital Stopped", "Program Stop", "Ring Stopped", "Timer laser Stopped", "Timer mérés Stopped", "Timers Stopped" {
            n93 = case shown="\"NI Analog Stopped\"" w316 {
              tunnel: [w327 w337 w347 w357 w367 w377 w387 w397 w407 w417 w427 w437 w448 w463] -> w321
              tunnel: w320 -> [w331 w341 w351 w361 w371 w381 w391 w401 w411 w421 w431 w438 w455 w464]
              tunnel: [w331 w341 w351 w361 w371 w381 w391 w401 w411 w421 w431 w438 w455 w464] -> w319
              tunnel: w318 -> [w322 w332 w343 w352 w362 w372 w382 w392 w403 w412 w422 w436 w445 w463]
              tunnel: w317 -> [w326 w336 w346 w356 w366 w376 w386 w396 w406 w416 w426 w435 w450 _]
              tunnel: w315 -> [w323 w333 w344 w353 w363 w373 w383 w393 w404 w413 w423 _ _ _]
              tunnel: w314 -> [_ _ _ _ _ _ _ _ _ _ _ _ w449 _]
              tunnel: [_ _ _ _ _ _ _ _ _ _ _ _ TRUE _] -> w313
              tunnel: w312 -> [_ _ _ _ _ _ _ _ _ _ _ _ _ _]
              tunnel: w311 -> [w330 w340 w350 w360 w370 w380 w390 w400 w410 w420 w430 w434 w446 w462]
              tunnel: [w329 w339 w349 w359 w369 w379 w389 w399 w409 w419 w429 w434 w446 w462] -> w310
              frame "Engine Stopped" {
                n94 = Unbundle By Name(w323) -> ("Engine"=w324:refnum<queue>)
                n95 = Release Queue(queue=w324, error in (no error)=w322) -> ()  [unwired: 1 in, 3 out]
                n96 = Bundle By Name(cluster=w330, "Engine Stopped"=TRUE) -> (w329:T11)
                n97 = call-poly "Enqueue Message.vi"("error in (no error)"=w322, "Message"="All Stopped?", "Message Queue"=w326) -> ("error out"=w327:errorcluster)  [unwired: 7 in, 1 out]
              }
              frame "Ring Stopped" {
                n98 = Unbundle By Name(w333) -> ("Ring"=w334:refnum<queue>)
                n99 = Release Queue(queue=w334, error in (no error)=w332) -> ()  [unwired: 1 in, 3 out]
                n100 = Bundle By Name(cluster=w340, "Ring Stopped"=TRUE ("Engine Stopped")) -> (w339:T11)
                n101 = call-poly "Enqueue Message.vi"("error in (no error)"=w332, "Message"="All Stopped?", "Message Queue"=w336) -> ("error out"=w337:errorcluster)  [unwired: 7 in, 1 out]
              }
              frame "Laser Stopped" {
                # "KÉSZ"
                n102 = Unbundle By Name(w344) -> ("Laser"=w345:refnum<queue>)
                n103 = Release Queue(queue=w345, error in (no error)=w343) -> ()  [unwired: 1 in, 3 out]
                n104 = Bundle By Name(cluster=w350, "Laser Stopped"=TRUE ("Engine Stopped")) -> (w349:T11)
                n105 = call-poly "Enqueue Message.vi"("error in (no error)"=w343, "Message"="All Stopped?", "Message Queue"=w346) -> ("error out"=w347:errorcluster)  [unwired: 7 in, 1 out]
              }
              frame "Keyence Stopped" {
                n106 = Unbundle By Name(w353) -> ("Keyence"=w354:refnum<queue>)
                n107 = Release Queue(queue=w354, error in (no error)=w352) -> ()  [unwired: 1 in, 3 out]
                n108 = Bundle By Name(cluster=w360, "Keyence Stopped"=TRUE ("Engine Stopped")) -> (w359:T11)
                n109 = call-poly "Enqueue Message.vi"("error in (no error)"=w352, "Message"="All Stopped?", "Message Queue"=w356) -> ("error out"=w357:errorcluster)  [unwired: 7 in, 1 out]
              }
              frame "Data Processor Stopped" {
                # "KÉSZ"
                n110 = Unbundle By Name(w363) -> ("Data Processor"=w364:refnum<queue>)
                n111 = Release Queue(queue=w364, error in (no error)=w362) -> ()  [unwired: 1 in, 3 out]
                n112 = Bundle By Name(cluster=w370, "Data Processor Stopped"=TRUE ("Engine Stopped")) -> (w369:T11)
                n113 = call-poly "Enqueue Message.vi"("error in (no error)"=w362, "Message"="All Stopped?", "Message Queue"=w366) -> ("error out"=w367:errorcluster)  [unwired: 7 in, 1 out]
              }
              frame "Timers Stopped" {
                # "KÉSZ"
                n114 = Unbundle By Name(w373) -> ("Timers"=w374:refnum<queue>)
                n115 = Release Queue(queue=w374, error in (no error)=w372) -> ()  [unwired: 1 in, 3 out]
                n116 = Bundle By Name(cluster=w380, "Timers Stopped"=TRUE ("Engine Stopped")) -> (w379:T11)
                n117 = call-poly "Enqueue Message.vi"("error in (no error)"=w372, "Message"="All Stopped?", "Message Queue"=w376) -> ("error out"=w377:errorcluster)  [unwired: 7 in, 1 out]
              }
              frame "Timer mérés Stopped" {
                # "KÉSZ"
                n118 = Unbundle By Name(w383) -> ("Timer mérés"=w384:refnum<queue>)
                n119 = Release Queue(queue=w384, error in (no error)=w382) -> ()  [unwired: 1 in, 3 out]
                n120 = Bundle By Name(cluster=w390, "Timer mérés Stopped"=TRUE ("Engine Stopped")) -> (w389:T11)
                n121 = call-poly "Enqueue Message.vi"("error in (no error)"=w382, "Message"="All Stopped?", "Message Queue"=w386) -> ("error out"=w387:errorcluster)  [unwired: 7 in, 1 out]
              }
              frame "Timer laser Stopped" {
                # "KÉSZ"
                n122 = Unbundle By Name(w393) -> ("Timer laser"=w394:refnum<queue>)
                n123 = Release Queue(queue=w394, error in (no error)=w392) -> ()  [unwired: 1 in, 3 out]
                n124 = Bundle By Name(cluster=w400, "Timer laser Stopped"=TRUE ("Engine Stopped")) -> (w399:T11)
                n125 = call-poly "Enqueue Message.vi"("error in (no error)"=w392, "Message"="All Stopped?", "Message Queue"=w396) -> ("error out"=w397:errorcluster)  [unwired: 7 in, 1 out]
              }
              frame "DAQ Stopped" {
                # "KÉSZ"
                n126 = Unbundle By Name(w404) -> ("DAQ"=w405:refnum<queue>)
                n127 = Release Queue(queue=w405, error in (no error)=w403) -> ()  [unwired: 1 in, 3 out]
                n128 = Bundle By Name(cluster=w410, "DAQ  Stopped"=TRUE ("Engine Stopped")) -> (w409:T11)
                n129 = call-poly "Enqueue Message.vi"("error in (no error)"=w403, "Message"="All Stopped?", "Message Queue"=w406) -> ("error out"=w407:errorcluster)  [unwired: 7 in, 1 out]
              }
              frame "NI Digital Stopped" {
                # "KÉSZ"
                n130 = Unbundle By Name(w413) -> ("NI Digital"=w414:refnum<queue>)
                n131 = Release Queue(queue=w414, error in (no error)=w412) -> ()  [unwired: 1 in, 3 out]
                n132 = Bundle By Name(cluster=w420, "NI Digital Stopped"=TRUE ("Engine Stopped")) -> (w419:T11)
                n133 = call-poly "Enqueue Message.vi"("error in (no error)"=w412, "Message"="All Stopped?", "Message Queue"=w416) -> ("error out"=w417:errorcluster)  [unwired: 7 in, 1 out]
              }
              frame "NI Analog Stopped" {
                # "KÉSZ"
                n134 = Unbundle By Name(w423) -> ("NI Analog"=w424:refnum<queue>)
                n135 = Release Queue(queue=w424, error in (no error)=w422) -> ()  [unwired: 1 in, 3 out]
                n136 = Bundle By Name(cluster=w430, "NI Analog Stopped"=TRUE ("Engine Stopped")) -> (w429:T11)
                n137 = call-poly "Enqueue Message.vi"("error in (no error)"=w422, "Message"="All Stopped?", "Message Queue"=w426) -> ("error out"=w427:errorcluster)  [unwired: 7 in, 1 out]
              }
              frame "All Stopped?" {
                # "KÉSZ"
                n138 = Cluster To Array(cluster=w434) -> (array=w433:bool[])
                n139 = And Array Elements(Boolean array=w433) -> (logical AND=w432:bool)
                n140 = case shown="False" w432 {
                  tunnel: [w439 w443] -> w437
                  tunnel: w436 -> [w439 w442]
                  tunnel: w435 -> [_ w441]
                  frame False {
                  }
                  frame True {
                    n141 = call-poly "Enqueue Message.vi"("Priority Message? (F)"=TRUE, "error in (no error)"=w442, "Message"="Program Stop", "Message Queue"=w441) -> ("error out"=w443:errorcluster)  [unwired: 6 in, 1 out]
                  }
                }
              }
              frame "Program Stop" {
                # "KÉSZ"
                n142 = flat-sequence {
                  tunnel: w449 -> [w458]
                  tunnel: [w458] -> w454
                  tunnel: w445 -> [w456]
                  tunnel: [w456] -> w453
                  tunnel: [w460] -> w451
                  tunnel: w454 -> [w461]
                  tunnel: w453 -> [w459]
                  frame #0 {
                    n143 = Wait (ms)(milliseconds to wait=u32 100) -> ()  [unwired: 1 out]
                  }
                  frame #1 {
                    n144 = call "Fire User Event - Stop.vi"("error in (no error)"=w459, "User Event - Stop"=w461) -> ("error out"=w460:errorcluster)  [unwired: 9 in]
                  }
                }
                n145 = Release Queue(queue=w450, error in (no error)=w445) -> (error out=w452:errorcluster)  [unwired: 1 in, 2 out]
                n146 = Merge Errors(w451, w452) -> (w448:errorcluster)
              }
              frame Default {
                # "KÉSZ"
              }
            }
          }
          frame "Mérés Következõ", "Mérés Lépésenként", "Mérés Start", "Mérés Vége", "Végig Mér" {
            n147 = case shown="\"Mérés Start\", \"Mérés Vége\"" w475 {
              tunnel: w474 -> [_ _ _ _ _]
              tunnel: w473 -> [w483 w494 w505 w516 w521]
              tunnel: w472 -> [w484 w495 w506 w517 _]
              tunnel: w471 -> [w482 w493 w504 w515 _]
              tunnel: w470 -> [_ _ _ _ _]
              tunnel: w469 -> [w478 w489 w500 w511 w522]
              tunnel: [w478 w489 w500 w511 w522] -> w468
              tunnel: [w476 w487 w498 w509 w521] -> w467
              tunnel: w465 -> [w481 w492 w503 w514 w520]
              tunnel: [w481 w492 w503 w514 w520] -> w466
              frame "Mérés Start", "Mérés Vége" {
                w480 = T23 {"Thread ID"=0, "Thread Flag"=FALSE}  # Thread Flag
                n148 = Unbundle By Name(w482) -> ("Engine"=w485:refnum<queue>)
                n149 = Variant To Data(error in=w483, type=w480, Variant=w484) -> (data=w479:T23, error out=w477:errorcluster)
                n150 = call-poly "Enqueue Message.vi"("error in (no error)"=w477, "Message Data"=w479, "Message"="Run", "Message Queue"=w485) -> ("error out"=w476:errorcluster)  [unwired: 6 in, 1 out]
              }
              frame "Mérés Következõ" {
                w491 = T23 {"Thread ID"=0, "Thread Flag"=FALSE}  # Thread Flag
                # "KÉSZ"
                n151 = Unbundle By Name(w493) -> ("Engine"=w496:refnum<queue>)
                n152 = Variant To Data(error in=w494, type=w491, Variant=w495) -> (data=w490:T23, error out=w488:errorcluster)
                n153 = call-poly "Enqueue Message.vi"("error in (no error)"=w488, "Message Data"=w490, "Message"="Pause", "Message Queue"=w496) -> ("error out"=w487:errorcluster)  [unwired: 6 in, 1 out]
              }
              frame "Végig Mér" {
                w502 = T23 {"Thread ID"=0, "Thread Flag"=FALSE}  # Thread Flag
                # "KÉSZ"
                n154 = Unbundle By Name(w504) -> ("Engine"=w507:refnum<queue>)
                n155 = Variant To Data(error in=w505, type=w502, Variant=w506) -> (data=w501:T23, error out=w499:errorcluster)
                n156 = call-poly "Enqueue Message.vi"("error in (no error)"=w499, "Message Data"=w501, "Message"="Ignore Error", "Message Queue"=w507) -> ("error out"=w498:errorcluster)  [unwired: 6 in, 1 out]
              }
              frame "Mérés Lépésenként" {
                w513 = T23 {"Thread ID"=0, "Thread Flag"=FALSE}  # Thread Flag
                # "KÉSZ"
                n157 = Unbundle By Name(w515) -> ("Engine"=w518:refnum<queue>)
                n158 = Variant To Data(error in=w516, type=w513, Variant=w517) -> (data=w512:T23, error out=w510:errorcluster)
                n159 = call-poly "Enqueue Message.vi"("error in (no error)"=w510, "Message Data"=w512, "Message"="Step Execution", "Message Queue"=w518) -> ("error out"=w509:errorcluster)  [unwired: 6 in, 1 out]
              }
              frame Default {
                # "KÉSZ"
              }
            }
          }
          frame "Etalon mérés", "Teszt beillesztése", "Teszt hozzáadása", "Teszt másolása", "Teszt módosítása", "Teszt szerkesztése", "Teszt törlése", "Teszt váltás Gyûrûzés", "Teszt váltás Mérés", "Tesztszekvencia eltávolítása", "Tesztszekvencia megnyitása", "Tesztszekvencia mentése", "Update Test Listbox" {
            n160 = case shown="\"Update Test Listbox\"" w533 {
              tunnel: w532 -> [_ _ _ _ _ _ _ _ _ _ _ _ _ _]
              tunnel: w531 -> [w547 w570 w593 w601 w609 w621 w635 w649 w663 w679 w708 w714 w725 w735]
              tunnel: w530 -> [w546 _ _ _ _ _ _ _ _ w680 w707 _ _ _]
              tunnel: w529 -> [w545 w573 w597 w600 w608 w624 w638 w652 w666 w681 _ w719 w730 _]
              tunnel: w528 -> [_ _ _ _ _ _ _ _ _ _ _ _ _ _]
              tunnel: w527 -> [w544 w572 w596 w605 w616 w623 w637 w651 w665 w672 w706 w720 w731 w736]
              tunnel: [w544 w572 w596 w605 w616 w623 w637 w651 w665 w672 w706 w720 w731 w736] -> w526
              tunnel: [w543 w571 w595 w602 w610 w625 w639 w653 w667 w676 w694 w721 w732 w735] -> w525
              tunnel: w524 -> [w539 w567 w594 w598 w607 w618 w631 w645 w659 w673 w695 w722 w733 w734]
              tunnel: [w539 w567 w594 w598 w607 w618 w631 w645 w659 w673 w695 w722 w733 w734] -> w523
              frame "Tesztszekvencia megnyitása" {
                # "KÉSZ"
                n161 = Variant To Data(error in=w547, type=T15 {"Thread Num"=enum."Mérés", "Elérési út"=path ""}, Variant=w546) -> (data=w537:T15, error out=w542:errorcluster)
                n162 = Unbundle By Name(w544) -> ("Etalon listbox"=w538:refnum<vi>, "Teszt vektor listbox"=w548:refnum<vi>)
                n163 = Unbundle By Name(w537) -> ("Thread Num"=w534:enum16{"Mérés", "Gyûrûzés"}, "Elérési út"=w536:path)
                n164 = call "Open file dialog.vi"("error in (no error)"=w542, "File Path Control"=w536) -> ("error out"=w541:errorcluster, "selected path"=w540:path)  [unwired: 7 in, 1 out]
                n165 = case shown="No Error" w541 {
                  selector: w541 -> [w554 w564]
                  tunnel: w548 -> [w562 _]
                  tunnel: w545 -> [w561 _]
                  tunnel: [w556 w563] -> w543
                  tunnel: w540 -> [w550 _]
                  tunnel: w538 -> [w551 _]
                  tunnel: w534 -> [w549 _]
                  frame No Error {
                    w560 = T24 {"Thread ID"=0, "Callback"="", "Data"=variant, "Error"={"status"=FALSE, "code"=0, "source"=""}}  # Message
                    n166 = call "Init listbox.vi"("error in (no error)"=w554, "MulticolumnListbox in"=w562) -> ("error out"=w553:errorcluster)  [unwired: 9 in]
                    n167 = call "Init listbox.vi"("error in (no error)"=w553, "MulticolumnListbox in"=w551) -> ("error out"=w552:errorcluster)  [unwired: 9 in]
                    n168 = Unbundle By Name(w561) -> ("Engine"=w557:refnum<queue>)
                    n169 = Bundle By Name(cluster=w560, "Thread ID"=w549, "Data"=w550, "Callback"="Update Test Listbox") -> (w559:T24)
                    n170 = call-poly "Enqueue Message.vi"("error in (no error)"=w552, "Message Data"=w559, "Message"="Open Test Sequence", "Message Queue"=w557) -> ("error out"=w556:errorcluster)  [unwired: 6 in, 1 out]
                  }
                  frame Error {
                    n171 = call <vilib>:"Clear Errors.vi"("error in (no error)"=w564, "specific error code to clear (0: all)"=43) -> ("error out"=w563:errorcluster)  [unwired: 4 in, 1 out]
                  }
                }
              }
              frame "Tesztszekvencia mentése" {
                # "KÉSZ"
                n172 = property on="Tesztszekvencia neve" class="Str"() -> ("Value"=w566:string)  [unwired: 2 in, 2 out]
                n173 = call "Save file Dialog.vi"("error in (no error)"=w570, "Default file name"=w566) -> ("error out"=w569:errorcluster, "selected path"=w568:path)  [unwired: 7 in, 1 out]
                n174 = case shown="No Error" w569 {
                  selector: w569 -> [w576 w585]
                  tunnel: w573 -> [w583 _]
                  tunnel: [w578 w584] -> w571
                  tunnel: w568 -> [w577 _]
                  frame No Error {
                    w582 = T24 {"Thread ID"=0, "Callback"="", "Data"=variant, "Error"={"status"=FALSE, "code"=0, "source"=""}}  # Message
                    n175 = local read "Thread Num"() -> (w574:enum16{"Mérés", "Gyûrûzés"})
                    n176 = Unbundle By Name(w583) -> ("Engine"=w579:refnum<queue>)
                    n177 = Bundle By Name(cluster=w582, "Thread ID"=w574, "Data"=w577, "Callback"="Update Test Listbox") -> (w581:T24)
                    n178 = call-poly "Enqueue Message.vi"("error in (no error)"=w576, "Message Data"=w581, "Message"="Save Test Sequence", "Message Queue"=w579) -> ("error out"=w578:errorcluster)  [unwired: 6 in, 1 out]
                  }
                  frame Error {
                    n179 = call <vilib>:"Clear Errors.vi"("error in (no error)"=w585, "specific error code to clear (0: all)"=43) -> ("error out"=w584:errorcluster)  [unwired: 4 in, 1 out]
                  }
                }
              }
              frame "Tesztszekvencia eltávolítása" {
                w592 = T24 {"Thread ID"=0, "Callback"="", "Data"=variant, "Error"={"status"=FALSE, "code"=0, "source"=""}}  # Message
                # "KÉSZ"
                n180 = local read "Thread Num"() -> (w587:enum16{"Mérés", "Gyûrûzés"})
                n181 = Unbundle By Name(w597) -> ("Engine"=w589:refnum<queue>)
                n182 = Bundle By Name(cluster=w592, "Thread ID"=w587, "Callback"="Update Test Listbox") -> (w591:T24)
                n183 = call-poly "Enqueue Message.vi"("error in (no error)"=w593, "Message Data"=w591, "Message"="Delete Test Sequence", "Message Queue"=w589) -> ("error out"=w595:errorcluster)  [unwired: 6 in, 1 out]
              }
              frame "Teszt szerkesztése" {
                w599 = T24 {"Thread ID"=0, "Callback"="", "Data"=variant, "Error"={"status"=FALSE, "code"=0, "source"=""}}  # Message
                n184 = Unbundle By Name(w600) -> ("Engine"=w603:refnum<queue>)
                n185 = call-poly "Enqueue Message.vi"("error in (no error)"=w601, "Message Data"=w599, "Message"="Edit Test", "Message Queue"=w603) -> ("error out"=w602:errorcluster)  [unwired: 6 in, 1 out]
              }
              frame "Teszt hozzáadása" {
                w615 = T24 {"Thread ID"=0, "Callback"="", "Data"=variant, "Error"={"status"=FALSE, "code"=0, "source"=""}}  # Message
                n186 = local read "Thread Num"() -> (w606:enum16{"Mérés", "Gyûrûzés"})
                n187 = Unbundle By Name(w608) -> ("Engine"=w612:refnum<queue>)
                n188 = Bundle By Name(cluster=w615, "Thread ID"=w606, "Callback"="Update Test Listbox") -> (w614:T24)
                n189 = call-poly "Enqueue Message.vi"("error in (no error)"=w609, "Message Data"=w614, "Message"="Add Test", "Message Queue"=w612) -> ("error out"=w610:errorcluster)  [unwired: 6 in, 1 out]
              }
              frame "Teszt másolása" {
                w629 = T24 {"Thread ID"=0, "Callback"="", "Data"=variant, "Error"={"status"=FALSE, "code"=0, "source"=""}}  # Message
                n190 = Unbundle By Name(w623) -> ("Teszt vektor listbox"=w622:refnum<vi>)
                n191 = property class="MCListbox"(reference=w622, error in=w621) -> (error out=w620:errorcluster, "Value"=w619:variant)  [unwired: 1 out]
                n192 = local read "Thread Num"() -> (w617:enum16{"Mérés", "Gyûrûzés"})
                n193 = Unbundle By Name(w624) -> ("Engine"=w626:refnum<queue>)
                n194 = Bundle By Name(cluster=w629, "Thread ID"=w617, "Data"=w619) -> (w628:T24)
                n195 = call-poly "Enqueue Message.vi"("error in (no error)"=w620, "Message Data"=w628, "Message"="Copy Test", "Message Queue"=w626) -> ("error out"=w625:errorcluster)  [unwired: 6 in, 1 out]
              }
              frame "Teszt beillesztése" {
                w643 = T24 {"Thread ID"=0, "Callback"="", "Data"=variant, "Error"={"status"=FALSE, "code"=0, "source"=""}}  # Message
                n196 = Unbundle By Name(w637) -> ("Teszt vektor listbox"=w636:refnum<vi>)
                n197 = property class="MCListbox"(reference=w636, error in=w635) -> (error out=w634:errorcluster, "Value"=w633:variant)  [unwired: 1 out]
                n198 = local read "Thread Num"() -> (w630:enum16{"Mérés", "Gyûrûzés"})
                n199 = Unbundle By Name(w638) -> ("Engine"=w640:refnum<queue>)
                n200 = Bundle By Name(cluster=w643, "Thread ID"=w630, "Data"=w633, "Callback"="Update Test Listbox") -> (w642:T24)
                n201 = call-poly "Enqueue Message.vi"("error in (no error)"=w634, "Message Data"=w642, "Message"="Paste Test", "Message Queue"=w640) -> ("error out"=w639:errorcluster)  [unwired: 6 in, 1 out]
              }
              frame "Teszt módosítása" {
                w657 = T24 {"Thread ID"=0, "Callback"="", "Data"=variant, "Error"={"status"=FALSE, "code"=0, "source"=""}}  # Message
                n202 = Unbundle By Name(w651) -> ("Teszt vektor listbox"=w650:refnum<vi>)
                n203 = property class="MCListbox"(reference=w650, error in=w649) -> (error out=w648:errorcluster, "Value"=w647:variant)  [unwired: 1 out]
                n204 = local read "Thread Num"() -> (w644:enum16{"Mérés", "Gyûrûzés"})
                n205 = Unbundle By Name(w652) -> ("Engine"=w654:refnum<queue>)
                n206 = Bundle By Name(cluster=w657, "Thread ID"=w644, "Data"=w647, "Callback"="Update Test Listbox") -> (w656:T24)
                n207 = call-poly "Enqueue Message.vi"("error in (no error)"=w648, "Message Data"=w656, "Message"="Modify Test", "Message Queue"=w654) -> ("error out"=w653:errorcluster)  [unwired: 6 in, 1 out]
              }
              frame "Teszt törlése" {
                w671 = T24 {"Thread ID"=0, "Callback"="", "Data"=variant, "Error"={"status"=FALSE, "code"=0, "source"=""}}  # Message
                n208 = Unbundle By Name(w665) -> ("Teszt vektor listbox"=w664:refnum<vi>)
                n209 = property class="MCListbox"(reference=w664, error in=w663) -> (error out=w662:errorcluster, "Value"=w661:variant)  [unwired: 1 out]
                n210 = local read "Thread Num"() -> (w658:enum16{"Mérés", "Gyûrûzés"})
                n211 = Unbundle By Name(w666) -> ("Engine"=w668:refnum<queue>)
                n212 = Bundle By Name(cluster=w671, "Thread ID"=w658, "Data"=w661, "Callback"="Update Test Listbox") -> (w670:T24)
                n213 = call-poly "Enqueue Message.vi"("error in (no error)"=w662, "Message Data"=w670, "Message"="Delete Test", "Message Queue"=w668) -> ("error out"=w667:errorcluster)  [unwired: 6 in, 1 out]
              }
              frame "Etalon mérés" {
                n214 = Variant To Data(error in=w679, type=TRUE, Variant=w680) -> (data=w674:bool, error out=w675:errorcluster)
                n215 = Unbundle By Name(w681) -> ("Engine"=w677:refnum<queue>)
                n216 = case shown="False" w674 {
                  tunnel: w675 -> [w685 w689]
                  tunnel: [w684 w688] -> w676
                  tunnel: w677 -> [w682 w686]
                  frame True {
                    n217 = call-poly "Enqueue Message.vi"("error in (no error)"=w685, "Message"="Set Etalon", "Message Queue"=w682) -> ("error out"=w684:errorcluster)  [unwired: 7 in, 1 out]
                  }
                  frame False {
                    n218 = call-poly "Enqueue Message.vi"("error in (no error)"=w689, "Message"="Reset Etalon", "Message Queue"=w686) -> ("error out"=w688:errorcluster)  [unwired: 7 in, 1 out]
                  }
                }
              }
              frame "Update Test Listbox" {
                w705 = T24 {"Thread ID"=0, "Callback"="", "Data"=variant, "Error"={"status"=FALSE, "code"=0, "source"=""}}  # Message
                # "KÉSZ"
                n219 = Variant To Data(error in=w708, type=w705, Variant=w707) -> (data=w703:T24, error out=w701:errorcluster)
                n220 = Unbundle By Name(w703) -> ("Data"=w702:variant)
                n221 = Unbundle By Name(w703) -> ("Thread ID"=w698:u16)
                n222 = Variant To Data(error in=w701, type=T16[] [], Variant=w702) -> (data=w699:T16[], error out=w694:errorcluster)
                n223 = Index Array(array=w699, index=w698) -> (element=w697:T16)
                n224 = Unbundle By Name(w697) -> ("File name"=→"Tesztszekvencia neve" →"Tesztszekvencia neve 2":string, "Program"=w696:T17[])
                n225 = for {
                  tunnel: w696 -> [w711] mode=indexing
                  tunnel: [w710] -> w692 mode=indexing
                  tunnel: [w709] -> w691 mode=indexing
                  n226 = call "Teszt cluster2string.vi"("Teszt cluster"=w711) -> ("Etalon string array"=w709:string[], "Teszt vektor string array"=w710:string[])  [unwired: 9 in]
                }
                n227 = Unbundle By Name(w706) -> ("Etalon listbox"=w704:refnum<vi>, "Teszt vektor listbox"=w693:refnum<vi>)
                n228 = property class="MCListbox"(reference=w693, "ItemNames"=w692) -> ()  [unwired: 1 in, 2 out]
                n229 = property class="MCListbox"(reference=w704, "ItemNames"=w691) -> ()  [unwired: 1 in, 2 out]
              }
              frame "Teszt váltás Mérés" {
                w712 = enum16{"Mérés", "Gyûrûzés"}."Mérés" ("Thread Num")
                w716 = T24 {"Thread ID"=0, "Callback"="", "Data"=variant, "Error"={"status"=FALSE, "code"=0, "source"=""}}  # Message
                n230 = local write "Thread Num 2"(w712) -> ()
                n231 = local write "Thread Num"(w712) -> ()
                n232 = Unbundle By Name(w719) -> ("Engine"=w718:refnum<queue>)
                n233 = Bundle By Name(cluster=w716, "Thread ID"=w712, "Callback"="Update Test Listbox") -> (w715:T24)
                n234 = call-poly "Enqueue Message.vi"("error in (no error)"=w714, "Message Data"=w715, "Message"="Select Test Sequence", "Message Queue"=w718) -> ("error out"=w721:errorcluster)  [unwired: 6 in, 1 out]
              }
              frame "Teszt váltás Gyûrûzés" {
                w723 = enum16{"Mérés", "Gyûrûzés"}."Gyûrûzés" ("Thread Num")
                w727 = T24 {"Thread ID"=0, "Callback"="", "Data"=variant, "Error"={"status"=FALSE, "code"=0, "source"=""}}  # Message
                n235 = local write "Thread Num 2"(w723) -> ()
                n236 = local write "Thread Num"(w723) -> ()
                n237 = Unbundle By Name(w730) -> ("Engine"=w729:refnum<queue>)
                n238 = Bundle By Name(cluster=w727, "Thread ID"=w723, "Callback"="Update Test Listbox") -> (w726:T24)
                n239 = call-poly "Enqueue Message.vi"("error in (no error)"=w725, "Message Data"=w726, "Message"="Select Test Sequence", "Message Queue"=w729) -> ("error out"=w732:errorcluster)  [unwired: 6 in, 1 out]
              }
              frame Default {
                # "KÉSZ"
              }
            }
          }
          frame "Termék mentése" {
            n240 = case shown="\"Termék mentése\"" w747 {
              tunnel: w746 -> [w751 _]
              tunnel: w745 -> [w750 w759]
              tunnel: w744 -> [_ _]
              tunnel: w743 -> [_ _]
              tunnel: w742 -> [_ _]
              tunnel: w741 -> [w757 w760]
              tunnel: [w757 w760] -> w740
              tunnel: [w752 w759] -> w739
              tunnel: [w748 w758] -> w738
              tunnel: w737 -> [w748 w758]
              frame "Termék mentése" {
                # "KÉSZ"
                n241 = local read "Termék cluster array"() -> (w753:T9[])
                n242 = call "Termék mentés.vi"("error in"=w750, "Termék cluster array"=w753) -> ("error out"=w754:errorcluster)  [unwired: 8 in, 1 out]
                n243 = call-poly "Enqueue Message.vi"("error in (no error)"=w754, "Message Data"="", "Message"="Set Statusbar", "Message Queue"=w751) -> ("error out"=w756:errorcluster)  [unwired: 6 in, 1 out]
                n244 = Merge Errors(w756) -> (w752:errorcluster)
              }
              frame Default {
                # "KÉSZ"
              }
            }
          }
          frame "Felhasználó mentés", "Felhasználó módosítása", "Felhasználó törlése", "Új felhasználó" {
            n245 = case shown="\"Új felhasználó\"" w771 {
              tunnel: w770 -> [w776 w801 w815 w849 _]
              tunnel: w769 -> [_ _ _ _ _]
              tunnel: w768 -> [w775 w800 w814 w841 w854]
              tunnel: w767 -> [_ _ _ _ _]
              tunnel: w766 -> [_ _ _ _ _]
              tunnel: w765 -> [w786 w810 w827 w852 w855]
              tunnel: [w786 w810 w827 w852 w855] -> w764
              tunnel: [w774 w802 w813 w848 w854] -> w763
              tunnel: [w772 w798 w811 w846 w853] -> w762
              tunnel: w761 -> [w772 w798 w811 w846 w853]
              frame "Új felhasználó" {
                # "KÉSZ"
                n246 = property on="Felhasználók Listbox" class="MCListbox (strict)"(error in=w775) -> (error out=w779:errorcluster, "ItemNames"=w783:string[][])  [unwired: 1 in, 1 out]
                n247 = call "Adatbevitel.vi"("Error In"=w775, "Felhasználói adatok in"=T19 {"NÉV:"="", "Jelszó: (csak számjegyek)"="", "Felhasználói szint"="Operátor"}) -> ("Error Out"=w781:errorcluster, "OK ?"=w778:bool, "Felhasználói adatok out"=w782:string[])  [unwired: 7 in]
                n248 = case shown="True" w778 {
                  tunnel: w783 -> [_ w796]
                  tunnel: w782 -> [_ w795]
                  tunnel: w781 -> [w788 w790]
                  tunnel: [w789 w793] -> w780
                  tunnel: w779 -> [w787 w791]
                  frame False {
                    n249 = Merge Errors(w787, w788) -> (w789:errorcluster)
                  }
                  frame True {
                    n250 = Build Array (concatenate)(w796, w795) -> (w794:string[][])
                    n251 = property on="Felhasználók Listbox" class="MCListbox (strict)"(error in=w791, "ItemNames"=w794) -> (error out=w792:errorcluster)  [unwired: 1 in, 1 out]
                    n252 = Merge Errors(w792, w790) -> (w793:errorcluster)
                  }
                }
                n253 = call-poly "Enqueue Message.vi"("error in (no error)"=w780, "Message Data"="", "Message"="Set Statusbar", "Message Queue"=w776) -> ("error out"=w785:errorcluster)  [unwired: 6 in, 1 out]
                n254 = Merge Errors(w785) -> (w774:errorcluster)
              }
              frame "Felhasználó törlése" {
                # "KÉSZ"
                n255 = property on="Felhasználók Listbox" class="MCListbox (strict)"(error in=w800) -> (error out=w803:errorcluster, "ItemNames"=w807:string[][], "Value"=w805:i32)  [unwired: 1 in, 1 out]
                n256 = Delete From Array(array=w807, length=1, index (row)=w805) -> (array with subset deleted=w804:string[][])  [unwired: 1 in, 1 out]
                n257 = property on="Felhasználók Listbox" class="MCListbox (strict)"(error in=w803, "ItemNames"=w804) -> (error out=w797:errorcluster)  [unwired: 1 in, 1 out]
                n258 = call-poly "Enqueue Message.vi"("error in (no error)"=w797, "Message Data"="", "Message"="Set Statusbar", "Message Queue"=w801) -> ("error out"=w809:errorcluster)  [unwired: 6 in, 1 out]
                n259 = Merge Errors(w809) -> (w802:errorcluster)
              }
              frame "Felhasználó módosítása" {
                # "KÉSZ"
                n260 = property on="Felhasználók Listbox" class="MCListbox (strict)"(error in=w814) -> (error out=w818:errorcluster, "ItemNames"=w821:string[][], "Value"=w819:i32)  [unwired: 1 in, 1 out]
                n261 = Index Array(array=w821, index (row)=w819) -> (element=w824:string[])  [unwired: 1 in]
                n262 = Array To Cluster(array=w824) -> (cluster=w823:T25)
                n263 = call "Adatbevitel.vi"("Error In"=w814, "Felhasználói adatok in"=w823) -> ("Error Out"=w822:errorcluster, "OK ?"=w816:bool, "Felhasználói adatok out"=w820:string[])  [unwired: 7 in]
                n264 = case shown="True" w816 {
                  tunnel: w822 -> [w829 w831]
                  tunnel: w821 -> [_ w838]
                  tunnel: w820 -> [_ w837]
                  tunnel: w819 -> [_ w836]
                  tunnel: w818 -> [w828 w833]
                  tunnel: [w830 w832] -> w817
                  frame False {
                    n265 = Merge Errors(w828, w829) -> (w830:errorcluster)
                  }
                  frame True {
                    n266 = Replace Array Subset(array=w838, new element=w837, index (row)=w836) -> (w835:string[][])  [unwired: 1 in]
                    n267 = property on="Felhasználók Listbox" class="MCListbox (strict)"(error in=w833, "ItemNames"=w835) -> (error out=w834:errorcluster)  [unwired: 1 in, 1 out]
                    n268 = Merge Errors(w834, w831) -> (w832:errorcluster)
                  }
                }
                n269 = call-poly "Enqueue Message.vi"("error in (no error)"=w817, "Message Data"="", "Message"="Set Statusbar", "Message Queue"=w815) -> ("error out"=w826:errorcluster)  [unwired: 6 in, 1 out]
                n270 = Merge Errors(w826) -> (w813:errorcluster)
              }
              frame "Felhasználó mentés" {
                # "KÉSZ"
                n271 = property on="Felhasználók Listbox" class="MCListbox (strict)"(error in=w841) -> (error out=w844:errorcluster, "ItemNames"=w845:string[][])  [unwired: 1 in, 1 out]
                n272 = call "Mentés.vi"("error in"=w844, "Felhasználói adatok in"=w845) -> ("error out"=w842:errorcluster)  [unwired: 9 in]
                n273 = call "Jogosultságok mentés.vi"("error in"=w841, "Jogosultság adatok in"="Jogosultságok array") -> ("error out"=w839:errorcluster)  [unwired: 9 in]
                n274 = Merge Errors(w839, w842) -> (w843:errorcluster)
                n275 = call-poly "Enqueue Message.vi"("error in (no error)"=w843, "Message Data"="", "Message"="Set Statusbar", "Message Queue"=w849) -> ("error out"=w851:errorcluster)  [unwired: 6 in, 1 out]
                n276 = Merge Errors(w851) -> (w848:errorcluster)
              }
              frame Default {
                # "KÉSZ"
              }
            }
          }
          frame "Reset Result Number Variables", "Set Meas Statusbar", "Set Result LED Variables", "Set Result Number Variables", "Set Statusbar", "Set Statusbar Main", "Set Statusbar Ring", "Set User" {
            n277 = case shown="\"Set User\"" w866 {
              selector: w866 -> [_ w891 _ _ _ _ _ _]
              tunnel: w865 -> [_ _ _ _ _ _ _ _]
              tunnel: w864 -> [w877 w888 w933 w945 w952 w962 w979 w987]
              tunnel: w863 -> [w876 w889 w934 w946 w953 w963 w980 _]
              tunnel: w862 -> [_ _ _ _ _ _ _ _]
              tunnel: w861 -> [_ _ _ _ _ _ _ _]
              tunnel: w860 -> [w878 w894 w936 w948 w955 w969 w981 w988]
              tunnel: [w878 w894 w936 w948 w955 w969 w981 w988] -> w859
              tunnel: [w869 w892 w932 w943 w950 w957 w974 w987] -> w858
              tunnel: [w875 w893 w935 w947 w954 w968 w978 w986] -> w857
              tunnel: w856 -> [w875 w893 w935 w947 w954 w968 w978 w986]
              frame "Set Result LED Variables" {
                w874 = T24 {"Thread ID"=0, "Callback"="", "Data"=variant, "Error"={"status"=FALSE, "code"=0, "source"=""}}  # Message
                # "KÉSZ"
                n278 = Variant To Data(error in=w877, type=w874, Variant=w876) -> (data=w873:T24, error out=w870:errorcluster)
                n279 = Unbundle By Name(w873) -> ("Thread ID"=w867:u16, "Data"=w872:variant)
                n280 = Variant To Data(error in=w870, type=T20 {"Jó"=FALSE, "Rossz"=FALSE, "Jó db"=0, "Rossz db"=0}, Variant=w872) -> (data=w868:T20, error out=w869:errorcluster)
                n281 = case shown="1" w867 {
                  tunnel: w868 -> [w881 w884]
                  frame 0, Default {
                    n282 = Unbundle By Name(w881) -> ("Jó"=→"JÓ" →"JÓ 2":bool, "Rossz"=→"Rossz" →"Rossz 2":bool)
                  }
                  frame 1 {
                    n283 = Unbundle By Name(w884) -> ("Jó"=→"JÓ 3":bool, "Rossz"=→"Rossz 3":bool)
                  }
                }
              }
              frame "Reset Result Number Variables", "Set Result Number Variables" {
                w890 = T24 {"Thread ID"=0, "Callback"="", "Data"=variant, "Error"={"status"=FALSE, "code"=0, "source"=""}}  # Message
                # "KÉSZ"
                n284 = Variant To Data(error in=w888, type=w890, Variant=w889) -> (data=w886:T24, error out=w885:errorcluster)
                n285 = Unbundle By Name(w886) -> ("Thread ID"=w887:u16)
                n286 = case shown="1" w887 {
                  tunnel: [w900 w916] -> w892
                  tunnel: w891 -> [w898 w915]
                  tunnel: w886 -> [w896 w912]
                  tunnel: w885 -> [w895 w911]
                  frame 0, Default {
                    n287 = case shown="\"Set Result Number Variables\"" w898 {
                      tunnel: [w901 w910] -> w900
                      tunnel: [w902 w909] -> w897
                      tunnel: [w902 w908] -> w899
                      tunnel: w896 -> [_ w905]
                      tunnel: w895 -> [w901 w903]
                      frame "Reset Result Number Variables", Default {
                        w902 = 0 ("Jó db")
                      }
                      frame "Set Result Number Variables" {
                        n288 = Unbundle By Name(w905) -> ("Data"=w904:variant)
                        n289 = Variant To Data(error in=w903, type=T20 {"Jó"=FALSE, "Rossz"=FALSE, "Jó db"=0, "Rossz db"=0}, Variant=w904) -> (data=w906:T20, error out=w910:errorcluster)
                        n290 = Unbundle By Name(w906) -> ("Jó db"=w909:i32, "Rossz db"=w908:i32)
                      }
                    }
                    "Rossz db" <- w899
                    "Jó db" <- w897
                  }
                  frame 1 {
                    n291 = case shown="\"Set Result Number Variables\"" w915 {
                      tunnel: [w917 w926] -> w916
                      tunnel: [w918 w925] -> w914
                      tunnel: [w918 w924] -> w913
                      tunnel: w912 -> [_ w920]
                      tunnel: w911 -> [w917 w919]
                      frame "Reset Result Number Variables", Default {
                        w918 = 0 ("Jó db")
                      }
                      frame "Set Result Number Variables" {
                        n292 = Unbundle By Name(w920) -> ("Data"=w921:variant)
                        n293 = Variant To Data(error in=w919, type=T20 {"Jó"=FALSE, "Rossz"=FALSE, "Jó db"=0, "Rossz db"=0}, Variant=w921) -> (data=w922:T20, error out=w926:errorcluster)
                        n294 = Unbundle By Name(w922) -> ("Jó db"=w925:i32, "Rossz db"=w924:i32)
                      }
                    }
                    "Jó db 2" <- w914
                    "Rossz db 2" <- w913
                  }
                }
              }
              frame "Set Statusbar" {
                w930 = ""
                # "KÉSZ"
                n295 = Variant To Data(error in=w933, type=w930, Variant=w934) -> (data=w928:string, error out=w931:errorcluster)
                n296 = Not Equal?(x=w930, y=w928) -> (x != y?=w929:bool)
                n297 = case shown="True" w929 {
                  tunnel: [w939 w941] -> w932
                  tunnel: w931 -> [w939 w941]
                  tunnel: w928 -> [w937 w940]
                  tunnel: [w937 w940] -> w927
                  frame False {
                    n298 = Wait (ms)(milliseconds to wait=u32 200) -> ()  [unwired: 1 out]
                  }
                  frame True {
                  }
                }
                "Állapot kijelzõ" <- w927
              }
              frame "Set Statusbar Main" {
                # "KÉSZ"
                n299 = Variant To Data(error in=w945, type="", Variant=w946) -> (data=→"Állapot kijelzõ fõképernyõ":string, error out=w943:errorcluster)
              }
              frame "Set Statusbar Ring" {
                # "KÉSZ"
                n300 = Variant To Data(error in=w952, type="", Variant=w953) -> (data=→"Állapot kijelzõ ring":string, error out=w950:errorcluster)
              }
              frame "Set Meas Statusbar" {
                w966 = T17 {"Thread ID"=0.0, "Mérésszám"="", "Mérés/Utasítás"="", "Command"={"Parancs"="", "Paraméter 1"="", "Paraméter 2"="", "Paraméter 3"="", "Paraméter 4"="", "Paraméter 5"="", "Eredmény"=""}, "Min"="", "Max"="", "Aktív?"=FALSE, "Log?"=FALSE, "Kiértékelés"=FALSE, "Etalon 1 exp"=FALSE, "Etalon 2 exp"=FALSE, "Etalon 3 exp"=FALSE, "Etalon 4 exp"=FALSE, "Etalon 5 exp"=FALSE}  # Teszt cluster
                w967 = T24 {"Thread ID"=0, "Callback"="", "Data"=variant, "Error"={"status"=FALSE, "code"=0, "source"=""}}  # Message
                # "KÉSZ"
                n301 = Variant To Data(error in=w962, type=w967, Variant=w963) -> (data=w959:T24, error out=w964:errorcluster)
                n302 = Unbundle By Name(w959) -> ("Thread ID"=w956:u16)
                n303 = Unbundle By Name(w959) -> ("Data"=w965:variant)
                n304 = Variant To Data(error in=w964, type=w966, Variant=w965) -> (data=w961:T17, error out=w958:errorcluster)
                n305 = Unbundle By Name(w961) -> ("Mérés/Utasítás"=w960:string)
                n306 = case shown="0, Default" w956 {
                  tunnel: w960 -> [_ w972]
                  tunnel: [w970 w971] -> w957
                  tunnel: w958 -> [w970 w971]
                  frame 1 {
                  }
                  frame 0, Default {
                    "Állapot kijelzõ 2" <- w972
                  }
                }
              }
              frame "Set User" {
                # "KÉSZ"
                n307 = Variant To Data(error in=w979, type=T19 {"NÉV:"="", "Jelszó: (csak számjegyek)"="", "Felhasználói szint"=""} ("Felhasználói adatok in"), Variant=w980) -> (data=w975:T19, error out=w974:errorcluster)
                n308 = Unbundle By Name(w975) -> ("NÉV:"=w973:string, "Felhasználói szint"=→"Jogosultság":string)
                "Felhasználó" <- w973
                n309 = global write "Global 1.vi" "Operator"(w973) -> ()
                n310 = case shown="Default" w973 {
                  frame Default {
                    n311 = property on="Felhasználó" class="Str"("Text.BGColor"=u32 16777216, "Text.TextColor"=u32 3381759) -> ()  [unwired: 2 in, 2 out]
                  }
                  frame "Kovács Edit" {
                    n312 = property on="Felhasználó" class="Str"("Text.BGColor"=u32 15888895, "Text.TextColor"=u32 0) -> ()  [unwired: 2 in, 2 out]
                  }
                }
              }
              frame Default {
                # "KÉSZ"
              }
            }
          }
          frame "Update Controls" {
            n313 = property on="Tab Control" class="TabCtl (strict)"(error in=w991) -> (error out=w993:errorcluster, "Pages"=w996:refnum<vi>[], "Value"=w995:T1)  [unwired: 1 in, 1 out]
            n314 = Index Array(array=w996, index=w995) -> (element=w994:refnum<vi>)
            n315 = property class="Page"(reference=w994, error in=w993) -> (error out=w990:errorcluster, "PageLabel"=w989:string)  [unwired: 1 out]
            n316 = property on="Tab control debug" class="TabCtl (strict)"(error in=w990) -> (error out=w998:errorcluster, "Pages"=w1003:refnum<vi>[], "Value"=w1002:enum32{"Digital IO", "Analog IO", "Laser"})  [unwired: 1 in, 1 out]
            n317 = Index Array(array=w1003, index=w1002) -> (element=w1001:refnum<vi>)
            n318 = property class="Page"(reference=w1001, error in=w998) -> (error out=w997:errorcluster, "PageLabel"=w1000:string)  [unwired: 1 out]
            n319 = case shown="\"Karbantartás / Debug\"" w989 {
              tunnel: w1000 -> [_ w1013]
              tunnel: w999 -> [w1008 w1012]
              tunnel: w997 -> [w1007 w1011]
              tunnel: [w1006 w1010] -> w992
              frame Default {
                n320 = call "AI engedélyezés refresh.vi"("error in (no error)"=w1007, "AI engedélyezés"=FALSE, "Message Queues in"=w1008) -> ("error out"=w1006:errorcluster)  [unwired: 8 in]
              }
              frame "Karbantartás / Debug" {
                n321 = case shown="\"Analog IO\"" w1013 {
                  tunnel: [w1014 w1018 w1031 w1043] -> w1010
                  tunnel: w1012 -> [w1016 w1021 w1034 w1042]
                  tunnel: w1011 -> [w1015 w1023 w1036 w1047]
                  frame Default {
                    n322 = call "AI engedélyezés refresh.vi"("error in (no error)"=w1015, "AI engedélyezés"=FALSE, "Message Queues in"=w1016) -> ("error out"=w1014:errorcluster)  [unwired: 8 in]
                  }
                  frame "Digital IO" {
                    w1024 = T4 {"PCIE-6321 OUT"={"Izolációs relé"=FALSE, "B oldal relé (nincs használva)"=FALSE, "48V relé"=FALSE, "Elszívás KI"=FALSE, "Bördelezés teszt"=FALSE, "Gyûrû megnyomás"=FALSE, "Termék rögzítés"=FALSE, "R mérés relé"=FALSE, "200mA relé"=FALSE, "NTC mérés relé"=FALSE, "Levegõ BE"=FALSE}}  # Digital Out
                    # "Össze kell hangolni\na mintavétellel"
                    n323 = Unbundle By Name(w1021) -> ("DO data"=w1026:refnum<queue>)
                    n324 = Wait (ms)(milliseconds to wait=u32 50) -> ()  [unwired: 1 out]
                    n325 = call "Preview Message.vi"("error in (no error)"=w1023, "Message Queue"=w1026) -> ("error out"=w1028:errorcluster, "Message Data"=w1029:variant)  [unwired: 5 in, 3 out]
                    n326 = Variant To Data(error in=w1028, type=w1024, Variant=w1029) -> (data=w1025:T4, error out=w1022:errorcluster)
                    n327 = local write "Digital Out"(w1025) -> ()
                    n328 = call <vilib>:"Clear Errors.vi"("error in (no error)"=w1022) -> ("error out"=w1019:errorcluster)  [unwired: 5 in, 1 out]
                    n329 = call "AI engedélyezés refresh.vi"("error in (no error)"=w1019, "AI engedélyezés"=FALSE, "Message Queues in"=w1021) -> ("error out"=w1018:errorcluster)  [unwired: 8 in]
                  }
                  frame "Analog IO" {
                    w1030 = T7 {"NI-6221"={"UCTRL"=0.0}}  # NI Analog Output
                    # "Össze kell hangolni\na mintavétellel"
                    n330 = Unbundle By Name(w1034) -> ("AO data"=w1038:refnum<queue>)
                    n331 = Wait (ms)(milliseconds to wait=u32 50) -> ()  [unwired: 1 out]
                    n332 = call "Preview Message.vi"("error in (no error)"=w1036, "Message Queue"=w1038) -> ("error out"=w1040:errorcluster, "Message Data"=w1041:variant)  [unwired: 5 in, 3 out]
                    n333 = Variant To Data(error in=w1040, type=w1030, Variant=w1041) -> (data=w1037:T7, error out=w1035:errorcluster)
                    n334 = local write "NI Analog Output"(w1037) -> ()
                    n335 = call <vilib>:"Clear Errors.vi"("error in (no error)"=w1035) -> ("error out"=w1032:errorcluster)  [unwired: 5 in, 1 out]
                    n336 = call "AI engedélyezés refresh.vi"("error in (no error)"=w1032, "AI engedélyezés"=TRUE, "Message Queues in"=w1034) -> ("error out"=w1031:errorcluster)  [unwired: 8 in]
                  }
                  frame "Laser" {
                    w1053 = T26 {"Communication Opened"=FALSE, "Status"={"Ready"=FALSE, "Error"=FALSE, "Warning"=FALSE, "Shutter"=FALSE, "Mark Check OK"=FALSE, "Mark Check NG"=FALSE, "Marking Busy"=FALSE, "Program No"=0, "Marking Check Busy"=FALSE, "Marking Completed"=FALSE, "Marking Score"=0, "Marking Error"=FALSE, "Marking Stop"=FALSE, "Program is changing"=FALSE, "Date/Time"=timestamp(0 s since 1904-01-01)}, "IP Address"="", "Laser Disabled"=FALSE}  # Keyence Data Cluster
                    # "Össze kell hangolni\na mintavétellel"
                    n337 = Unbundle By Name(w1042) -> ("Keyence Data"=w1051:refnum<queue>)
                    n338 = Wait (ms)(milliseconds to wait=u32 50) -> ()  [unwired: 1 out]
                    n339 = call "Preview Message.vi"("error in (no error)"=w1047, "Message Queue"=w1051) -> ("error out"=w1055:errorcluster, "Message Data"=w1056:variant)  [unwired: 5 in, 3 out]
                    n340 = Variant To Data(error in=w1055, type=w1053, Variant=w1056) -> (data=w1052:T26, error out=w1050:errorcluster)
                    n341 = Unbundle By Name(w1052) -> ("Communication Opened"=w1049:bool, "Status.Program No"=w1048:u16, "Laser Disabled"=w1046:bool)
                    n342 = call <vilib>:"Clear Errors.vi"("error in (no error)"=w1050) -> ("error out"=w1044:errorcluster)  [unwired: 5 in, 1 out]
                    n343 = local write "Keyence Open"(w1049) -> ()
                    n344 = local write "Program No"(w1048) -> ()
                    n345 = local write "Keyence Disable"(w1046) -> ()
                    n346 = call "AI engedélyezés refresh.vi"("error in (no error)"=w1044, "AI engedélyezés"=FALSE, "Message Queues in"=w1042) -> ("error out"=w1043:errorcluster)  [unwired: 8 in]
                  }
                }
              }
            }
          }
          frame "OUTPUT Analog Write", "OUTPUT PortWrite" {
            n347 = case shown="\"OUTPUT Analog Write\"" w1061 {
              selector: w1061 -> [_ w1071 w1079]
              tunnel: w1065 -> [w1066 w1076 w1084]
              tunnel: w1064 -> [_ w1075 w1083]
              tunnel: w1063 -> [_ w1074 w1082]
              tunnel: [w1066 w1073 w1081] -> w1062
              tunnel: w1060 -> [w1068 w1070 w1078]
              tunnel: [w1068 w1070 w1078] -> w1059
              tunnel: w1058 -> [w1067 w1069 w1077]
              tunnel: [w1067 w1069 w1077] -> w1057
              frame Default {
              }
              frame "OUTPUT PortWrite" {
                n348 = Unbundle By Name(w1074) -> ("NI Digital"=w1072:refnum<queue>)
                n349 = call-poly "Enqueue Message.vi"("error in (no error)"=w1076, "Message Data"=w1075, "Message"=w1071, "Message Queue"=w1072) -> ("error out"=w1073:errorcluster)  [unwired: 6 in, 1 out]
              }
              frame "OUTPUT Analog Write" {
                n350 = Unbundle By Name(w1082) -> ("NI Analog"=w1080:refnum<queue>)
                n351 = call-poly "Enqueue Message.vi"("error in (no error)"=w1084, "Message Data"=w1083, "Message"=w1079, "Message Queue"=w1080) -> ("error out"=w1081:errorcluster)  [unwired: 6 in, 1 out]
              }
            }
          }
          frame "KEYENCE Error Clear", "KEYENCE Laser Disable", "KEYENCE Marking", "KEYENCE Open Connection", "KEYENCE Program Change", "KEYENCE Program Read", "KEYENCE Update Sys Time" {
            n352 = Unbundle By Name(w1089) -> ("Keyence"=w1085:refnum<queue>)
            n353 = call-poly "Enqueue Message.vi"("error in (no error)"=w1091, "Message Data"=w1090, "Message"=w1092, "Message Queue"=w1085) -> ("error out"=w1087:errorcluster)  [unwired: 6 in, 1 out]
          }
          frame "Kiértékelés Etalon UI", "Kiértékelés Ring UI", "Kiértékelés UI", "Mérés Continue UI", "Mérés Init UI", "Mérés Pause UI", "Mérés Start UI", "Mérés Vége UI", "Méréseredmény UI", "Write logfile" {
            n354 = case shown="\"Méréseredmény UI\"" w1103 {
              tunnel: w1102 -> [w1114 w1141 _ _ _ w1263 w1301 w1329 _ _ _]
              tunnel: w1101 -> [w1115 w1142 w1164 w1180 w1206 w1271 w1309 w1341 w1363 w1378 w1390]
              tunnel: w1100 -> [w1116 w1143 w1165 w1181 w1207 w1274 w1312 w1344 w1366 w1379 _]
              tunnel: w1099 -> [_ _ _ _ _ _ _ _ _ _ _]
              tunnel: w1098 -> [_ _ _ _ _ _ _ _ _ _ _]
              tunnel: w1097 -> [w1112 w1140 w1169 w1185 w1202 w1264 w1302 w1335 w1358 w1383 w1391]
              tunnel: [w1112 w1140 w1169 w1185 w1202 w1264 w1302 w1335 w1358 w1383 w1391] -> w1096
              tunnel: [w1120 w1147 w1171 w1187 w1205 w1273 w1311 w1343 w1365 w1382 w1390] -> w1095
              tunnel: [w1119 w1146 w1170 w1186 w1204 w1272 w1310 w1342 w1364 w1384 w1389] -> w1094
              tunnel: w1093 -> [w1119 w1146 w1170 w1186 w1204 w1272 w1310 w1342 w1364 w1384 w1389]
              frame "Mérés Init UI" {
                w1117 = T24 {"Thread ID"=0, "Callback"="", "Data"=variant, "Error"={"status"=FALSE, "code"=0, "source"=""}}  # Message
                # "EZ NINCS IS HASZNÁLVA!!!"
                n355 = Variant To Data(error in=w1115, type=w1117, Variant=w1116) -> (data=w1110:T24, error out=w1105:errorcluster)
                n356 = Unbundle By Name(w1110) -> ("Thread ID"=w1106:u16)
                n357 = case shown="1" w1106 {
                  tunnel: w1112 -> [w1126 _]
                  tunnel: w1105 -> [w1123 w1127]
                  tunnel: [w1121 w1128] -> w1104
                  frame 0, Default {
                    n358 = Unbundle By Name(w1126) -> ("Eredmény listbox"=w1124:refnum<vi>, "Mérés listbox"=w1125:refnum<vi>)
                    n359 = call "Init listbox.vi"("error in (no error)"=w1123, "MulticolumnListbox in"=w1125) -> ("error out"=w1122:errorcluster)  [unwired: 9 in]
                    n360 = call "Init listbox.vi"("error in (no error)"=w1122, "MulticolumnListbox in"=w1124) -> ("error out"=w1121:errorcluster)  [unwired: 9 in]
                  }
                  frame 1 {
                    n361 = disable-structure shown="Enabled" {
                      disable-tunnel: [w1130 w1131] -> w1128
                      disable-tunnel: w1127 -> [w1129 w1131]
                      frame Disabled {
                        n362 = call "Init listbox.vi"("error in (no error)"=w1129) -> ("error out"=w1130:errorcluster)  [unwired: 10 in]
                      }
                      frame Enabled {
                      }
                    }
                  }
                }
                n363 = call "Meas Init UI.vi"("error in (no error)"=w1104, "UI Data in"=w1112) -> ("error out"=w1113:errorcluster)  [unwired: 9 in]
                n364 = Bundle By Name(cluster=w1110, "Data"=T20 {"Jó"=FALSE, "Rossz"=FALSE, "Jó db"=1, "Rossz db"=1}) -> (w1108:T24)
                n365 = call-poly "Enqueue Message.vi"("Priority Message? (F)"=TRUE, "error in (no error)"=w1113, "Message Data"=w1108, "Message"="Set Result LED Variables", "Message Queue"=w1114) -> ("error out"=w1118:errorcluster)  [unwired: 5 in, 1 out]
                n366 = Merge Errors(w1118) -> (w1120:errorcluster)
              }
              frame "Mérés Start UI" {
                w1144 = T24 {"Thread ID"=0, "Callback"="", "Data"=variant, "Error"={"status"=FALSE, "code"=0, "source"=""}}  # Message
                # "KÉSZ"
                n367 = Variant To Data(error in=w1142, type=w1144, Variant=w1143) -> (data=w1138:T24, error out=w1133:errorcluster)
                n368 = Unbundle By Name(w1138) -> ("Thread ID"=w1134:u16)
                n369 = case shown="0" w1134 {
                  tunnel: w1140 -> [w1155 _ _]
                  tunnel: w1133 -> [w1154 w1156 w1161]
                  tunnel: [w1150 w1157 w1161] -> w1132
                  frame 0 {
                    n370 = Unbundle By Name(w1155) -> ("Eredmény listbox"=w1152:refnum<vi>, "Mérés listbox"=w1153:refnum<vi>)
                    n371 = call "Meas Start UI.vi"("error in (no error)"=w1154, "UI Data in"=w1155) -> ("error out"=w1151:errorcluster)  [unwired: 9 in]
                    n372 = call "Init listbox.vi"("error in (no error)"=w1151, "MulticolumnListbox in"=w1153) -> ("error out"=w1148:errorcluster)  [unwired: 9 in]
                    n373 = call "Init listbox.vi"("error in (no error)"=w1151, "MulticolumnListbox in"=w1152) -> ("error out"=w1149:errorcluster)  [unwired: 9 in]
                    n374 = Merge Errors(w1149, w1148) -> (w1150:errorcluster)
                  }
                  frame 1 {
                    n375 = disable-structure shown="Enabled" {
                      disable-tunnel: [w1159 w1160] -> w1157
                      disable-tunnel: w1156 -> [w1158 w1160]
                      frame Disabled {
                        n376 = call "Init listbox.vi"("error in (no error)"=w1158) -> ("error out"=w1159:errorcluster)  [unwired: 10 in]
                      }
                      frame Enabled {
                      }
                    }
                  }
                  frame Default {
                  }
                }
                n377 = Bundle By Name(cluster=w1138, "Data"=T20 {"Jó"=FALSE, "Rossz"=FALSE, "Jó db"=1, "Rossz db"=1}) -> (w1136:T24)
                n378 = call-poly "Enqueue Message.vi"("Priority Message? (F)"=TRUE, "error in (no error)"=w1132, "Message Data"=w1136, "Message"="Set Result LED Variables", "Message Queue"=w1141) -> ("error out"=w1145:errorcluster)  [unwired: 5 in, 1 out]
                n379 = Merge Errors(w1145) -> (w1147:errorcluster)
              }
              frame "Mérés Pause UI" {
                w1167 = T24 {"Thread ID"=0, "Callback"="", "Data"=variant, "Error"={"status"=FALSE, "code"=0, "source"=""}}  # Message
                # "KÉSZ"
                n380 = Variant To Data(error in=w1164, type=w1167, Variant=w1165) -> (data=w1166:T24, error out=w1162:errorcluster)
                n381 = Unbundle By Name(w1166) -> ("Thread ID"=w1163:u16)
                n382 = case shown="0" w1163 {
                  tunnel: w1169 -> [_ w1177]
                  tunnel: [w1172 w1174] -> w1168
                  tunnel: w1162 -> [w1172 w1173]
                  frame Default {
                  }
                  frame 0 {
                    n383 = Unbundle By Name(w1177) -> ("Mérés következõ"=w1176:refnum<vi>)
                    n384 = property on="Property Node" class="Bool"(reference=w1176, error in=w1173, "DisabledEnum"=T21."Enabled" ("Disabled")) -> (error out=w1174:errorcluster)  [unwired: 1 out]
                  }
                }
                n385 = Merge Errors(w1168) -> (w1171:errorcluster)
              }
              frame "Mérés Continue UI" {
                w1183 = T24 {"Thread ID"=0, "Callback"="", "Data"=variant, "Error"={"status"=FALSE, "code"=0, "source"=""}}  # Message
                # "KÉSZ"
                n386 = Variant To Data(error in=w1180, type=w1183, Variant=w1181) -> (data=w1182:T24, error out=w1178:errorcluster)
                n387 = Unbundle By Name(w1182) -> ("Thread ID"=w1179:u16)
                n388 = case shown="0" w1179 {
                  tunnel: w1185 -> [_ w1193]
                  tunnel: [w1188 w1190] -> w1184
                  tunnel: w1178 -> [w1188 w1189]
                  frame Default {
                  }
                  frame 0 {
                    n389 = Unbundle By Name(w1193) -> ("Mérés következõ"=w1192:refnum<vi>)
                    n390 = property on="Property Node" class="Bool"(reference=w1192, error in=w1189, "DisabledEnum"=T21."Disabled and Grayed Out" ("Disabled")) -> (error out=w1190:errorcluster)  [unwired: 1 out]
                  }
                }
                n391 = Merge Errors(w1184) -> (w1187:errorcluster)
              }
              frame "Méréseredmény UI" {
                w1201 = T17 {"Thread ID"=0.0, "Mérésszám"="", "Mérés/Utasítás"="", "Command"={"Parancs"="", "Paraméter 1"="", "Paraméter 2"="", "Paraméter 3"="", "Paraméter 4"="", "Paraméter 5"="", "Eredmény"=""}, "Min"="", "Max"="", "Aktív?"=FALSE, "Log?"=FALSE, "Kiértékelés"=FALSE, "Etalon 1 exp"=FALSE, "Etalon 2 exp"=FALSE, "Etalon 3 exp"=FALSE, "Etalon 4 exp"=FALSE, "Etalon 5 exp"=FALSE}  # Teszt cluster
                w1203 = T24 {"Thread ID"=0, "Callback"="", "Data"=variant, "Error"={"status"=FALSE, "code"=0, "source"=""}}  # Message
                # "KÉSZ"
                n392 = Variant To Data(error in=w1206, type=w1203, Variant=w1207) -> (data=w1199:T24, error out=w1198:errorcluster)
                n393 = Unbundle By Name(w1199) -> ("Thread ID"=w1194:u16)
                n394 = Unbundle By Name(w1199) -> ("Data"=w1200:variant)
                n395 = Variant To Data(error in=w1198, type=w1201, Variant=w1200) -> (data=w1197:T17, error out=w1196:errorcluster)
                n396 = case shown="0, Default" w1194 {
                  tunnel: w1202 -> [w1217 _]
                  tunnel: w1197 -> [w1208 w1237]
                  tunnel: w1196 -> [w1216 w1236]
                  tunnel: [w1215 w1235] -> w1195
                  frame 0, Default {
                    n397 = Unbundle By Name(w1217) -> ("Eredmény listbox"=w1209:refnum<vi>, "Mérés listbox"=w1210:refnum<vi>)
                    n398 = Unbundle By Name(w1208) -> ("Log?"=w1212:bool, "Kiértékelés"=w1214:bool)
                    n399 = Not(x=w1214) -> (.not. x?=w1213:bool)
                    n400 = Or(x=w1212, y=w1213) -> (x .or. y?=w1211:bool)
                    n401 = case shown="True" w1211 {
                      tunnel: [w1218 w1224] -> w1215
                      tunnel: w1216 -> [w1218 w1228]
                      tunnel: w1210 -> [_ w1227]
                      tunnel: w1209 -> [_ w1223]
                      tunnel: w1208 -> [_ w1222]
                      frame False {
                      }
                      frame True {
                        n402 = call "Add Row to Listbox.vi"("List size"=23, "error in"=w1228, "Teszt cluster"=w1222, "MulticolumnListbox in"=w1227) -> ("error out"=w1225:errorcluster)  [unwired: 7 in]
                        n403 = Unbundle By Name(w1222) -> ("Mérésszám"=w1221:string)
                        n404 = Not Equal?(x=w1221, y="") -> (x != y?=w1219:bool)
                        n405 = case shown="True" w1219 {
                          tunnel: w1225 -> [w1229 w1234]
                          tunnel: [w1229 w1233] -> w1224
                          tunnel: w1223 -> [_ w1232]
                          tunnel: w1222 -> [_ w1230]
                          frame False {
                          }
                          frame True {
                            n406 = call "Add Row to Listbox.vi"("List size"=19, "error in"=w1234, "Teszt cluster"=w1230, "MulticolumnListbox in"=w1232) -> ("error out"=w1233:errorcluster)  [unwired: 7 in]
                          }
                        }
                      }
                    }
                  }
                  frame 1 {
                    n407 = disable-structure shown="Enabled" {
                      disable-tunnel: w1237 -> [w1244 _]
                      disable-tunnel: w1236 -> [w1243 w1250]
                      disable-tunnel: [w1242 w1250] -> w1235
                      frame Disabled {
                        n408 = Unbundle By Name(w1244) -> ("Log?"=w1239:bool, "Kiértékelés"=w1241:bool)
                        n409 = Not(x=w1241) -> (.not. x?=w1240:bool)
                        n410 = Or(x=w1239, y=w1240) -> (x .or. y?=w1238:bool)
                        n411 = case shown="True" w1238 {
                          tunnel: [w1245 w1249] -> w1242
                          tunnel: w1243 -> [w1245 w1248]
                          tunnel: w1244 -> [_ w1246]
                          frame False {
                          }
                          frame True {
                            n412 = call "Add Row to Listbox.vi"("List size"=23, "error in"=w1248, "Teszt cluster"=w1246) -> ("error out"=w1249:errorcluster)  [unwired: 8 in]
                          }
                        }
                      }
                      frame Enabled {
                      }
                    }
                  }
                }
                n413 = Merge Errors(w1195) -> (w1205:errorcluster)
              }
              frame "Kiértékelés UI" {
                w1270 = T24 {"Thread ID"=0, "Callback"="", "Data"=variant, "Error"={"status"=FALSE, "code"=0, "source"=""}}  # Message
                # "OK"
                n414 = Variant To Data(error in=w1271, type=w1270, Variant=w1274) -> (data=w1262:T24, error out=w1267:errorcluster)
                n415 = Unbundle By Name(w1262) -> ("Data"=w1269:variant)
                n416 = Variant To Data(error in=w1267, type=FALSE, Variant=w1269) -> (data=w1266:bool, error out=w1265:errorcluster)
                n417 = local read "Jó db"() -> (w1255:i32)
                n418 = local read "Rossz db"() -> (w1254:i32)
                n419 = case shown="True" w1266 {
                  tunnel: w1255 -> [w1278 w1285]
                  tunnel: w1254 -> [w1276 w1284]
                  tunnel: [w1275 w1282] -> w1252
                  frame True {
                    n420 = Increment(x=w1278) -> (x+1=w1277:i32)
                    n421 = Bundle By Name(cluster=T20 {"Jó"=FALSE, "Rossz"=FALSE, "Jó db"=0, "Rossz db"=0}, "Jó"=TRUE, "Rossz"=FALSE ("Jó"), "Jó db"=w1277, "Rossz db"=w1276) -> (w1275:T20)
                  }
                  frame False {
                    n422 = Increment(x=w1284) -> (x+1=w1283:i32)
                    n423 = Bundle By Name(cluster=T20 {"Jó"=FALSE, "Rossz"=FALSE, "Jó db"=0, "Rossz db"=0}, "Jó"=FALSE, "Rossz"=TRUE ("Jó"), "Jó db"=w1285, "Rossz db"=w1283) -> (w1282:T20)
                  }
                }
                n424 = Bundle By Name(cluster=w1262, "Data"=w1252) -> (w1251:T24)
                n425 = call-poly "Enqueue Message.vi"("Priority Message? (F)"=TRUE, "error in (no error)"=w1265, "Message Data"=w1251, "Message"="Set Result Number Variables", "Message Queue"=w1263) -> ("error out"=w1258:errorcluster, "dup Message Queue"=w1257:refnum<queue>)  [unwired: 5 in]
                n426 = call-poly "Enqueue Message.vi"("Priority Message? (F)"=TRUE, "error in (no error)"=w1258, "Message Data"=w1251, "Message"="Set Result LED Variables", "Message Queue"=w1257) -> ("error out"=w1261:errorcluster)  [unwired: 5 in, 1 out]
                n427 = Merge Errors(w1261) -> (w1273:errorcluster)
              }
              frame "Kiértékelés Ring UI" {
                w1308 = T24 {"Thread ID"=0, "Callback"="", "Data"=variant, "Error"={"status"=FALSE, "code"=0, "source"=""}}  # Message
                # "OK"
                n428 = Variant To Data(error in=w1309, type=w1308, Variant=w1312) -> (data=w1300:T24, error out=w1305:errorcluster)
                n429 = Unbundle By Name(w1300) -> ("Data"=w1307:variant)
                n430 = Variant To Data(error in=w1305, type=FALSE, Variant=w1307) -> (data=w1304:bool, error out=w1303:errorcluster)
                n431 = local read "Jó db 2"() -> (w1293:i32)
                n432 = local read "Rossz db 2"() -> (w1292:i32)
                n433 = case shown="True" w1304 {
                  tunnel: w1293 -> [w1316 w1323]
                  tunnel: w1292 -> [w1314 w1322]
                  tunnel: [w1313 w1320] -> w1290
                  frame True {
                    n434 = Increment(x=w1316) -> (x+1=w1315:i32)
                    n435 = Bundle By Name(cluster=T20 {"Jó"=FALSE, "Rossz"=FALSE, "Jó db"=0, "Rossz db"=0}, "Jó"=TRUE, "Rossz"=FALSE ("Jó"), "Jó db"=w1315, "Rossz db"=w1314) -> (w1313:T20)
                  }
                  frame False {
                    n436 = Increment(x=w1322) -> (x+1=w1321:i32)
                    n437 = Bundle By Name(cluster=T20 {"Jó"=FALSE, "Rossz"=FALSE, "Jó db"=0, "Rossz db"=0}, "Jó"=FALSE, "Rossz"=TRUE ("Jó"), "Jó db"=w1323, "Rossz db"=w1321) -> (w1320:T20)
                  }
                }
                n438 = Bundle By Name(cluster=w1300, "Data"=w1290) -> (w1289:T24)
                n439 = call-poly "Enqueue Message.vi"("Priority Message? (F)"=TRUE, "error in (no error)"=w1303, "Message Data"=w1289, "Message"="Set Result Number Variables", "Message Queue"=w1301) -> ("error out"=w1296:errorcluster, "dup Message Queue"=w1295:refnum<queue>)  [unwired: 5 in]
                n440 = call-poly "Enqueue Message.vi"("Priority Message? (F)"=TRUE, "error in (no error)"=w1296, "Message Data"=w1289, "Message"="Set Result LED Variables", "Message Queue"=w1295) -> ("error out"=w1299:errorcluster)  [unwired: 5 in, 1 out]
                n441 = Merge Errors(w1299) -> (w1311:errorcluster)
              }
              frame "Kiértékelés Etalon UI" {
                w1340 = T24 {"Thread ID"=0, "Callback"="", "Data"=variant, "Error"={"status"=FALSE, "code"=0, "source"=""}}  # Message
                # "OK"
                n442 = Variant To Data(error in=w1341, type=w1340, Variant=w1344) -> (data=w1334:T24, error out=w1337:errorcluster)
                n443 = Unbundle By Name(w1334) -> ("Data"=w1339:variant)
                n444 = Variant To Data(error in=w1337, type=FALSE, Variant=w1339) -> (data=w1336:bool, error out=w1328:errorcluster)
                n445 = case shown="True" w1336 {
                  tunnel: [w1345 w1349] -> w1330
                  frame True {
                    n446 = Bundle By Name(cluster=T20 {"Jó"=FALSE, "Rossz"=FALSE, "Jó db"=0, "Rossz db"=0}, "Jó"=TRUE, "Rossz"=FALSE ("Jó")) -> (w1345:T20)
                  }
                  frame False {
                    n447 = Bundle By Name(cluster=T20 {"Jó"=FALSE, "Rossz"=FALSE, "Jó db"=0, "Rossz db"=0}, "Jó"=FALSE, "Rossz"=TRUE ("Jó")) -> (w1349:T20)
                  }
                }
                n448 = Bundle By Name(cluster=w1334, "Data"=w1330) -> (w1327:T24)
                n449 = call-poly "Enqueue Message.vi"("Priority Message? (F)"=TRUE, "error in (no error)"=w1328, "Message Data"=w1327, "Message"="Set Result LED Variables", "Message Queue"=w1329) -> ("error out"=w1333:errorcluster)  [unwired: 5 in, 1 out]
                n450 = Merge Errors(w1333) -> (w1343:errorcluster)
              }
              frame "Write logfile" {
                w1353 = u32 0  # Etalon number
                w1362 = T24 {"Thread ID"=0, "Callback"="", "Data"=variant, "Error"={"status"=FALSE, "code"=0, "source"=""}}  # Message
                # "LOG IDE JÖN"
                n451 = Variant To Data(error in=w1363, type=w1362, Variant=w1366) -> (data=w1359:T24, error out=w1360:errorcluster)
                n452 = Unbundle By Name(w1359) -> ("Thread ID"=w1357:u16)
                n453 = Unbundle By Name(w1359) -> ("Data"=w1361:variant)
                n454 = Variant To Data(error in=w1360, type=w1353, Variant=w1361) -> (data=w1355:u32, error out=w1356:errorcluster)
                n455 = case shown="0, Default" w1357 {
                  tunnel: w1358 -> [w1373 _]
                  tunnel: w1356 -> [w1372 w1375]
                  tunnel: w1355 -> [w1367 _]
                  tunnel: [w1371 w1375] -> w1354
                  frame 0, Default {
                    n456 = Unbundle By Name(w1373) -> ("Teszt vektor listbox"=w1369:refnum<vi>, "Mérés listbox"=w1368:refnum<vi>)
                    n457 = local read "Termék"() -> (w1374:string)
                    n458 = call "Generate logfile path 2.vi"("error in"=w1372, "Típus"=w1374, "Etalon number"=w1367) -> ("error out"=w1371:errorcluster, "Log_Path"=w1370:path)  [unwired: 7 in]
                    n459 = call "Generate logfile 3.vi"("Mérés"=w1368, "Teszt vektor listbox"=w1369, "Log_Path"=w1370) -> ()  [unwired: 9 in]
                  }
                  frame 1 {
                  }
                }
                n460 = Merge Errors(w1354) -> (w1365:errorcluster)
              }
              frame "Mérés Vége UI" {
                w1381 = T24 {"Thread ID"=0, "Callback"="", "Data"=variant, "Error"={"status"=FALSE, "code"=0, "source"=""}}  # Message
                # "KÉSZ"
                n461 = Variant To Data(error in=w1378, type=w1381, Variant=w1379) -> (data=w1380:T24, error out=w1377:errorcluster)
                n462 = Unbundle By Name(w1380) -> ("Thread ID"=w1376:u16)
                n463 = case shown="0" w1376 {
                  tunnel: w1383 -> [_ w1388]
                  tunnel: [w1385 w1387] -> w1382
                  tunnel: w1377 -> [w1385 w1386]
                  frame Default {
                  }
                  frame 0 {
                    n464 = call "Meas End UI.vi"("error in (no error)"=w1386, "UI Data in"=w1388) -> ("error out"=w1387:errorcluster)  [unwired: 9 in]
                  }
                }
              }
              frame Default {
                # "KÉSZ"
              }
            }
          }
          frame "Error", "Error 9100" {
            # "Hibakezelés, a hibaüzenetet az error handler VI küldi minden ciklus végén"
            n465 = case shown="\"Error\"" w1394 {
              tunnel: w1400 -> [w1403 w1415 w1425]
              tunnel: w1399 -> [_ w1414 _]
              tunnel: w1398 -> [_ w1412 w1424]
              tunnel: [w1403 w1411 w1422] -> w1397
              tunnel: w1396 -> [w1402 w1405 w1432]
              tunnel: [w1402 w1405 w1432] -> w1395
              tunnel: w1393 -> [w1401 w1404 w1427]
              tunnel: [w1401 w1404 w1426] -> w1392
              frame Default {
              }
              frame "Error" {
                n466 = Variant To Data(error in=w1415, type=errorcluster {"status"=FALSE, "code"=0, "source"=""} ("error constant"), Variant=w1414) -> (data=w1408:errorcluster, error out=w1410:errorcluster)
                n467 = Unbundle By Name(w1408) -> ("code"=w1409:i32)
                n468 = case shown="Default" w1409 {
                  tunnel: w1408 -> [w1418 w1420]
                  tunnel: ["Initiate Stop" "Error 9100"] -> w1406
                  frame Default {
                    # "Késleltetés hogy a hibás VI le tudjon állni és visszajelezni hogy már nem fut"
                    n469 = call <vilib>:"Simple Error Handler.vi"("error in (no error)"=w1418) -> ()  [unwired: 4 in, 5 out]
                    n470 = Wait (ms)(milliseconds to wait=u32 100) -> ()  [unwired: 1 out]
                  }
                  frame -9100 {
                    # "Késleltetés hogy a hibás VI le tudjon állni és visszajelezni hogy már nem fut"
                    n471 = call <vilib>:"Simple Error Handler.vi"("error in (no error)"=w1420) -> ()  [unwired: 4 in, 5 out]
                    n472 = Wait (ms)(milliseconds to wait=u32 100) -> ()  [unwired: 1 out]
                  }
                }
                n473 = call-poly "Enqueue Message.vi"("Priority Message? (F)"=TRUE, "error in (no error)"=w1410, "Message"=w1406, "Message Queue"=w1412) -> ("error out"=w1411:errorcluster)  [unwired: 6 in, 1 out]
              }
              frame "Error 9100" {
                n474 = property on="Felhasználók Listbox" class="MCListbox (strict)"(error in=w1425) -> (error out=w1429:errorcluster, "ItemNames"=w1430:string[][])  [unwired: 1 in, 1 out]
                n475 = call "Bejelentkezés.vi"("Error In"=w1429, "Message Queue"=w1424, "Felhasználói adatok in"=w1430) -> ("Error Out"=w1423:errorcluster, "OK ?"=w1431:bool, "Felhasználó ki"=w1428:T19)  [unwired: 6 in]
                n476 = case shown="True" w1431 {
                  tunnel: [w1438 w1444] -> w1426
                  tunnel: w1423 -> [w1433 w1445]
                  tunnel: w1428 -> [_ w1439]
                  tunnel: w1427 -> [w1438 w1442]
                  tunnel: w1424 -> [w1436 w1441]
                  tunnel: [w1437 w1440] -> w1422
                  frame False {
                    n477 = call-poly "Enqueue Message.vi"("Priority Message? (F)"=TRUE, "error in (no error)"=w1433, "Message"="Initiate Stop", "Message Queue"=w1436) -> ("error out"=w1437:errorcluster)  [unwired: 6 in, 1 out]
                  }
                  frame True {
                    n478 = Unbundle By Name(w1439) -> ("Felhasználói szint"=w1443:string)
                    n479 = case shown="\"Mérnök\"" w1443 {
                      selector: w1443 -> [_ w1464]
                      tunnel: w1445 -> [w1446 w1454]
                      tunnel: [w1451 w1466] -> w1444
                      tunnel: w1442 -> [w1451 w1463]
                      tunnel: w1441 -> [w1448 w1456]
                      tunnel: [w1447 w1453] -> w1440
                      tunnel: w1439 -> [_ w1452]
                      frame Default {
                        n480 = call-poly "Enqueue Message.vi"("Priority Message? (F)"=TRUE, "error in (no error)"=w1446, "Message"="Initiate Stop", "Message Queue"=w1448) -> ("error out"=w1447:errorcluster)  [unwired: 6 in, 1 out]
                      }
                      frame "Mérnök" {
                        n481 = call "Fõképernyõ UI engedélyezés.vi"("Error In"=w1454, "Felhasználói szint"=w1464, "UI Data"=w1463) -> ("Error Out"=w1468:errorcluster, "Felhasználói szint ki"=w1465:string, "UI Data out"=w1467:T22)  [unwired: 6 in]
                        n482 = call-poly "Enqueue Message.vi"("error in (no error)"=w1454, "Message Data"=w1452, "Message"="Set User", "Message Queue"=w1456) -> ("error out"=w1461:errorcluster, "dup Message Queue"=w1462:refnum<queue>)  [unwired: 6 in]
                        n483 = call "Mérésképernyõ UI engedélyezés.vi"("Error In"=w1468, "Felhasználói szint"=w1465, "UI Data"=w1467) -> ("Error Out"=w1455:errorcluster, "UI Data out"=w1466:T22)  [unwired: 7 in]
                        n484 = call-poly "Enqueue Message.vi"("error in (no error)"=w1461, "Message Data"="", "Message"="Set Statusbar", "Message Queue"=w1462) -> ("error out"=w1457:errorcluster)  [unwired: 6 in, 1 out]
                        n485 = Merge Errors(w1455, w1457) -> (w1453:errorcluster)
                      }
                    }
                  }
                }
              }
            }
          }
          frame "Confirm Quit" {
            # "Rákérdezünk hogy biztosan ki akar-e lépni a programból."
            n486 = Two Button Dialog(message="Biztosan kilép a programból?", 1:"Mégsem" ("F button name (\"Cancel\")"), 2:"Igen" ("T button name (\"OK\")")) -> (T button?=w1471:bool)
            n487 = case shown="True" w1471 {
              tunnel: w1477 -> [w1478 w1483]
              tunnel: w1476 -> [_ w1482]
              tunnel: [w1478 w1479] -> w1472
              frame False {
              }
              frame True {
                n488 = call-poly "Enqueue Message.vi"("Priority Message? (F)"=TRUE, "error in (no error)"=w1483, "Message"="Initiate Stop", "Message Queue"=w1482) -> ("error out"=w1479:errorcluster)  [unwired: 6 in, 1 out]
              }
            }
          }
          frame Default {
            # "Nem létezõ parancs esetén fut csak le, hibát generál"
            n489 = xnode "Error Ring"("parameter 0"=w1486) -> ("error out"=w1487:errorcluster)
          }
        }
      }
      frame True {
        n490 = property on="Tab Control" class="TabCtl (strict)"(error in=w1498) -> (error out=w1497:errorcluster, "Pages"=w1505:refnum<vi>[], "Value"=w1504:T1)  [unwired: 1 in, 1 out]
        n491 = Index Array(array=w1505, index=w1504) -> (element=w1503:refnum<vi>)
        n492 = property class="Page"(reference=w1503, error in=w1497) -> (error out=w1496:errorcluster, "PageLabel"=w1499:string)  [unwired: 1 out]
        n493 = property on="Tab control debug" class="TabCtl (strict)"(error in=w1496) -> (error out=w1495:errorcluster, "Pages"=w1510:refnum<vi>[], "Value"=w1509:enum32{"Digital IO", "Analog IO", "Laser"})  [unwired: 1 in, 1 out]
        n494 = Index Array(array=w1510, index=w1509) -> (element=w1508:refnum<vi>)
        n495 = property class="Page"(reference=w1508, error in=w1495) -> ("PageLabel"=w1507:string)  [unwired: 2 out]
        n496 = case shown="\"Karbantartás / Debug\"" w1499 {
          tunnel: w1507 -> [_ w1520]
          tunnel: w1506 -> [w1515 w1519]
          tunnel: w1498 -> [w1514 w1518]
          tunnel: [w1514 w1517] -> w1502
          tunnel: [w1515 w1516] -> w1501
          frame Default {
          }
          frame "Karbantartás / Debug" {
            n497 = case shown="\"Analog IO\"" w1520 {
              tunnel: [w1521 w1523 w1537 w1549] -> w1517
              tunnel: w1519 -> [w1522 w1524 w1539 w1550]
              tunnel: w1518 -> [w1521 w1526 w1543 w1552]
              tunnel: [w1522 w1524 w1539 w1550] -> w1516
              frame Default {
              }
              frame "Digital IO" {
                w1531 = T3 {"PCIE-6321 IN"={"Termék bördelezve"=FALSE, "Izolációs relék OK"=FALSE, "Rézgyûrû a terméken"=FALSE, "Termék rögzítve"=FALSE, "Termék a gyûrûzõben"=FALSE, "Rézgyûrû behelyezve"=FALSE, "Rézgyûrû elengedve"=FALSE, "Rézgyûrû megnyomva"=FALSE, "Termék elengedve"=FALSE, "Levegõ rendben"=FALSE, "Termék jelen (táv)"=FALSE, "Termék jelen (fém)"=FALSE, "Selejt érzékelõ"=FALSE}}  # Digital input
                # "Össze kell hangolni\na mintavétellel"
                n498 = Unbundle By Name(w1524) -> ("DI data"=w1527:refnum<queue>)
                n499 = Wait (ms)(milliseconds to wait=u32 50) -> ()  [unwired: 1 out]
                n500 = call "Preview Message.vi"("error in (no error)"=w1526, "Message Queue"=w1527) -> ("error out"=w1529:errorcluster, "Message Data"=w1530:variant)  [unwired: 5 in, 3 out]
                n501 = Variant To Data(error in=w1529, type=w1531, Variant=w1530) -> (data=→"Digital input":T3, error out=w1523:errorcluster)
              }
              frame "Analog IO" {
                w1536 = T27 {"Dummy"=FALSE, "R Res"=0.0, "NTC Res"=0.0, "Insulation Res"=0.0, "Temperature"=0.0, "NTC Exp Res"=0.0, "NTC Calc Temp"=0.0, "Delta U Puffer"=refnum, "I Adj Parameters"={"Vr NTC"=0.0, "Vr R"=0.0, "Vr dU"=0.0, "I Adj step"=0, "Output"=0.0, "Adj Failed"=FALSE}, "UCTRL Cluster"={"UCTRL NTC"=0.0, "UCTRL R"=0.0, "UCTRL dU"=0.0}}  # Data Processor Data Cluster
                w1545 = T5 {"NI-6221"={"Sensor"=0.0, "Uref"=0.0, "Temperature"=0.0, "Uisol"=0.0, "NTC"=0.0, "U48"=0.0, "U15"=0.0}, "Analog Result"={"Szenzor ellenállás"=0.0, "NTC ellenállás"=0.0, "Szigetelési ellenállás"=0.0, "Hõmérséklet"=0.0, "48V"=0.0, "15V"=0.0, "Elvárt NTC ellenállás"=0.0, "Számolt NTC hõmérséklet"=0.0}, "AI engedélyezés"=FALSE, "dU"=[]}  # NI Analog Input
                n502 = Unbundle By Name(w1539) -> ("Data Processor data"=w1540:refnum<queue>)
                n503 = Unbundle By Name(w1539) -> ("Analog UI Data"=w1548:refnum<queue>)
                n504 = call "Preview Message.vi"("error in (no error)"=w1543, "Message Queue"=w1548) -> ("error out"=w1547:errorcluster, "Message Data"=w1546:variant)  [unwired: 5 in, 3 out]
                n505 = Variant To Data(error in=w1547, type=w1545, Variant=w1546) -> (data=→"NI Analog Input":T5, error out=w1538:errorcluster)
                n506 = call "Preview Message.vi"("error in (no error)"=w1538, "Message Queue"=w1540) -> ("error out"=w1541:errorcluster, "Message Data"=w1542:variant)  [unwired: 5 in, 3 out]
                n507 = Variant To Data(error in=w1541, type=w1536, Variant=w1542) -> (data=w1535:T27, error out=w1537:errorcluster)
                n508 = Unbundle By Name(w1535) -> ("UCTRL Cluster.UCTRL NTC"=→"UCTRL NTC":dbl, "UCTRL Cluster.UCTRL R"=→"UCTRL R":dbl, "UCTRL Cluster.UCTRL dU"=→"UCTRL dU":dbl)
              }
              frame "Laser" {
                w1556 = T26 {"Communication Opened"=FALSE, "Status"={"Ready"=FALSE, "Error"=FALSE, "Warning"=FALSE, "Shutter"=FALSE, "Mark Check OK"=FALSE, "Mark Check NG"=FALSE, "Marking Busy"=FALSE, "Program No"=0, "Marking Check Busy"=FALSE, "Marking Completed"=FALSE, "Marking Score"=0, "Marking Error"=FALSE, "Marking Stop"=FALSE, "Program is changing"=FALSE, "Date/Time"=timestamp(0 s since 1904-01-01)}, "IP Address"="", "Laser Disabled"=FALSE}  # Keyence Data Cluster
                # "Össze kell hangolni\na mintavétellel"
                n509 = Unbundle By Name(w1550) -> ("Keyence Data"=w1553:refnum<queue>)
                n510 = Wait (ms)(milliseconds to wait=u32 50) -> ()  [unwired: 1 out]
                n511 = call "Preview Message.vi"("error in (no error)"=w1552, "Message Queue"=w1553) -> ("error out"=w1558:errorcluster, "Message Data"=w1559:variant)  [unwired: 5 in, 3 out]
                n512 = Variant To Data(error in=w1558, type=w1556, Variant=w1559) -> (data=w1555:T26, error out=w1549:errorcluster)
                n513 = Unbundle By Name(w1555) -> ("Status"=→"Status":T8, "Communication Opened"=→"Communication opened":bool)
              }
            }
          }
        }
        n514 = case shown="\"Fõképernyõ\"" w1499 {
          tunnel: [w1560 w1569] -> w1500
          tunnel: w1502 -> [w1560 w1570]
          tunnel: w1501 -> [_ w1563]
          frame Default {
          }
          frame "Fõképernyõ" {
            w1567 = T5 {"NI-6221"={"Sensor"=0.0, "Uref"=0.0, "Temperature"=0.0, "Uisol"=0.0, "NTC"=0.0, "U48"=0.0, "U15"=0.0}, "Analog Result"={"Szenzor ellenállás"=0.0, "NTC ellenállás"=0.0, "Szigetelési ellenállás"=0.0, "Hõmérséklet"=0.0, "48V"=0.0, "15V"=0.0, "Elvárt NTC ellenállás"=0.0, "Számolt NTC hõmérséklet"=0.0}, "AI engedélyezés"=FALSE, "dU"=[]}  # NI Analog Input
            w1571 = T3 {"PCIE-6321 IN"={"Termék bördelezve"=FALSE, "Izolációs relék OK"=FALSE, "Rézgyûrû a terméken"=FALSE, "Termék rögzítve"=FALSE, "Termék a gyûrûzõben"=FALSE, "Rézgyûrû behelyezve"=FALSE, "Rézgyûrû elengedve"=FALSE, "Rézgyûrû megnyomva"=FALSE, "Termék elengedve"=FALSE, "Levegõ rendben"=FALSE, "Termék jelen (táv)"=FALSE, "Termék jelen (fém)"=FALSE, "Selejt érzékelõ"=FALSE}}  # Digital input
            n515 = Unbundle By Name(w1563) -> ("DI data"=w1568:refnum<queue>)
            n516 = Unbundle By Name(w1563) -> ("Analog UI Data"=w1564:refnum<queue>)
            n517 = call "Preview Message.vi"("error in (no error)"=w1570, "Message Queue"=w1568) -> ("error out"=w1574:errorcluster, "Message Data"=w1572:variant)  [unwired: 5 in, 3 out]
            n518 = Variant To Data(error in=w1574, type=w1571, Variant=w1572) -> (data=w1573:T3, error out=w1569:errorcluster)
            n519 = Unbundle By Name(w1573) -> ("PCIE-6321 IN.Rézgyûrû behelyezve"=→"Gyûrû behelyezve":bool, "PCIE-6321 IN.Termék a gyûrûzõben"=→"Termék behelyezve":bool, "PCIE-6321 IN.Rézgyûrû megnyomva"=→"Gyûrû megnyomva":bool)
            n520 = call "Preview Message.vi"("Message Queue"=w1564) -> ("error out"=w1565:errorcluster, "Message Data"=w1566:variant)  [unwired: 6 in, 3 out]
            n521 = Variant To Data(error in=w1565, type=w1567, Variant=w1566) -> (data=w1562:T5)  [unwired: 1 out]
            n522 = Unbundle By Name(w1562) -> ("dU"=→"dU görbe":dbl[])
          }
        }
      }
    }
    "Loops" <- w60
    n523 = call "Error Handler - Message Handling Loop.vi"("error in (no error)"=w65, "Message Queue"=w67) -> ("dup error in"=w66:errorcluster)  [unwired: 8 in, 1 out]
  }
  n524 = call "DAQ Input Handler.vi"("error in (no error)"=w3, "Message Queues out"=w1) -> ("error out"=w36:errorcluster)  [unwired: 8 in, 1 out]
  n525 = call "Data Processor.vi"("error in (no error)"=w3, "Message Queues out"=w1) -> ("error out"=w32:errorcluster)  [unwired: 8 in, 1 out]
  n526 = call "Timer.vi"("error in (no error)"=w3, "Message Queues in"=w1) -> ("error out"=w46:errorcluster)  [unwired: 8 in, 1 out]
  n527 = call "Engine.vi"("Error In"=w3, "Message Queues"=w1) -> ("Error Out"=w49:errorcluster)  [unwired: 9 in]
  n528 = call "Ring handler.vi"("error in (no error)"=w3, "Message Queues out"=w1) -> ("error out"=w11:errorcluster)  [unwired: 8 in, 1 out]
  n529 = call "Laser handler.vi"("error in (no error)"=w3, "Message Queues out"=w1) -> ("error out"=w21:errorcluster)  [unwired: 8 in, 1 out]
  n530 = while {
    tunnel: w50 -> [w1587]
    shift-right: [w1585] -> w53
    shift-left: w12 -> [w1586]
    shift-right: [w1581] -> w52
    shift-left: w3 -> [w1579]
    tunnel: w1 -> [w1578]
    stop <- w1583 stop-if-true
    # "Event Handling Loop"
    n531 = event shown="[45] \"Setup UCTRL R\": Value Change" {
      selector: w1586 -> [_ _ _ _ _ _ _ _ _ _ _ _ _ _ _ _ _ _ _ _ _ _ _ _ _ _ _ _ _ _ _ _ _ _ _ _ _ _ _ _ _ _ _ _ _ _ _]
      dyn-events: [_ _ _ _ _ _ _ _ _ _ _ _ _ _ _ _ _ _ _ _ _ _ _ _ _ _ _ _ _ _ _ _ _ _ _ _ _ _ _ _ _ _ _ _ _ _ _] -> w1585
      timeout: 100 -> [_ _ _ _ _ _ _ _ _ _ _ _ _ _ _ _ _ _ _ _ _ _ _ _ _ _ _ _ _ _ _ _ _ _ _ _ _ _ _ _ _ _ _ _ _ _ _]
      tunnel: [_ _ _ _ _ _ _ _ _ _ _ _ _ _ _ _ _ _ _ _ _ _ _ _ _ _ _ _ _ _ _ _ _ _ _ _ _ _ _ _ TRUE ("Discard?") _ _ _ _ _ _] -> w1583
      tunnel: w1587 -> [w1589 w1595 w1611 w1623 w1639 w1650 w1657 w1673 w1690 w1711 w1720 w1725 w1740 w1752 w1755 w1761 w1773 w1785 w1797 w1809 w1821 w1834 w1850 w1862 w1874 w1886 w1905 w1910 w1923 w1936 w1948 w1960 w1973 w1979 w1984 w2000 w2016 w2032 w2048 w2050 w2053 w2060 w2078 w2088 w2092 w2118 w2146]
      tunnel: [w1588 w1593 w1609 w1621 w1637 w1651 w1655 w1671 w1688 w1709 w1718 w1723 w1738 w1753 w1756 w1759 w1771 w1783 w1795 w1807 w1819 w1832 w1848 w1860 w1872 w1884 w1903 w1908 w1921 w1934 w1946 w1958 w1971 w1977 w1982 w1998 w2014 w2030 w2047 _ w2051 w2064 w2075 w2085 w2089 w2115 w2155] -> w1584
      tunnel: [w1589 w1594 w1610 w1622 w1638 w1652 w1656 w1672 w1689 w1710 w1719 w1724 w1739 w1752 w1755 w1760 w1772 w1784 w1796 w1808 w1820 w1833 w1849 w1861 w1873 w1885 w1904 w1909 w1922 w1935 w1947 w1959 w1972 w1976 w1983 w1999 w2015 w2031 w2046 w2050 w2053 w2059 w2077 w2087 w2091 w2117 w2145] -> w1582
      tunnel: w1579 -> [w1588 w1591 w1607 w1620 w1636 w1649 w1654 w1670 w1687 w1708 w1717 w1722 w1737 w1753 w1756 w1757 w1769 w1781 w1793 w1806 w1818 w1831 w1847 w1859 w1871 w1883 w1902 w1907 w1920 w1933 w1945 w1957 w1970 w1978 w1980 w1997 w2012 w2028 _ _ w2052 w2063 w2076 w2086 w2090 w2116 w2156]
      tunnel: w1578 -> [_ _ _ _ _ _ _ _ _ _ _ _ _ _ _ _ _ _ _ _ _ _ _ _ _ _ _ _ _ _ _ _ _ _ _ _ _ _ _ _ _ _ _ _ w2094 w2120 _]
      event Timeout {
        # "Meg lehet tenni user eventtel is -> olyankor biztosan nem maradunk le a gyors váltásokról!"
        # "Kijelzõ frissítése"
        n532 = event-data() -> ()  [unwired: 1 in, 3 out]
        n533 = Get Date/Time In Seconds() -> (seconds since 1Jan1904=→"Digitális Óra":timestamp)
      }
      event "Felhasználó váltás": Value Change {
        n534 = event-data() -> ("NewVal"=w1592:bool)  [unwired: 1 in]
        n535 = case shown="True" w1592 {
          tunnel: w1595 -> [w1596 w1599]
          tunnel: [w1596 w1606] -> w1594
          tunnel: [w1597 w1604] -> w1593
          tunnel: w1591 -> [w1597 w1602]
          frame False {
          }
          frame True {
            n536 = call-poly "Enqueue Message.vi"("error in (no error)"=w1602, "Message Data"="Felhasználó váltás" ("Message"), "Message"="Set Statusbar", "Message Queue"=w1599) -> ("error out"=w1601:errorcluster, "dup Message Queue"=w1598:refnum<queue>)  [unwired: 6 in]
            n537 = call-poly "Enqueue Message.vi"("error in (no error)"=w1601, "Message"="Felhasználó váltás", "Message Queue"=w1598) -> ("error out"=w1604:errorcluster, "dup Message Queue"=w1606:refnum<queue>)  [unwired: 7 in]
          }
        }
      }
      event "Kilépés": Value Change {
        n538 = event-data() -> ("NewVal"=w1608:bool)  [unwired: 1 in]
        n539 = case shown="True" w1608 {
          tunnel: w1611 -> [w1612 w1618]
          tunnel: [w1612 w1617] -> w1610
          tunnel: [w1613 w1615] -> w1609
          tunnel: w1607 -> [w1613 w1614]
          frame False {
          }
          frame True {
            n540 = call-poly "Enqueue Message.vi"("error in (no error)"=w1614, "Message"="Kilépés", "Message Queue"=w1618) -> ("error out"=w1615:errorcluster, "dup Message Queue"=w1617:refnum<queue>)  [unwired: 7 in]
          }
        }
      }
      event "Termék választás": Value Change {
        n541 = event-data() -> ("NewVal"=w1619:bool)  [unwired: 1 in]
        n542 = case shown="True" w1619 {
          tunnel: w1623 -> [w1624 w1626]
          tunnel: [w1624 w1634] -> w1622
          tunnel: [w1625 w1632] -> w1621
          tunnel: w1620 -> [w1625 w1629]
          frame False {
          }
          frame True {
            n543 = call-poly "Enqueue Message.vi"("error in (no error)"=w1629, "Message Data"="Termék választás" ("Message"), "Message"="Set Statusbar", "Message Queue"=w1626) -> ("error out"=w1628:errorcluster, "dup Message Queue"=w1627:refnum<queue>)  [unwired: 6 in]
            n544 = call-poly "Enqueue Message.vi"("error in (no error)"=w1628, "Message"="Termék választás", "Message Queue"=w1627) -> ("error out"=w1632:errorcluster, "dup Message Queue"=w1634:refnum<queue>)  [unwired: 7 in]
          }
        }
      }
      event "Karbantartás": Value Change {
        n545 = event-data() -> ("NewVal"=w1635:bool)  [unwired: 1 in]
        n546 = case shown="True" w1635 {
          tunnel: w1639 -> [w1641 w1646]
          tunnel: [w1641 w1645] -> w1638
          tunnel: [w1640 w1643] -> w1637
          tunnel: w1636 -> [w1640 w1642]
          frame False {
          }
          frame True {
            n547 = call-poly "Enqueue Message.vi"("error in (no error)"=w1642, "Message"="Karbantartás képernyõ", "Message Queue"=w1646) -> ("error out"=w1643:errorcluster, "dup Message Queue"=w1645:refnum<queue>)  [unwired: 7 in]
          }
        }
      }
      event "Stop": Value Change {
        n548 = event-data() -> ()  [unwired: 1 in, 5 out]
        n549 = call-poly "Enqueue Message.vi"("Priority Message? (F)"=TRUE, "error in (no error)"=w1649, "Message"="Initiate Stop", "Message Queue"=w1650) -> ("error out"=w1651:errorcluster, "dup Message Queue"=w1652:refnum<queue>)  [unwired: 6 in]
      }
      event "Mérés start", "Mérés start 2": Value Change {
        n550 = event-data() -> ("NewVal"=w1653:bool)  [unwired: 1 in]
        n551 = case shown="True" w1653 {
          selector: w1653 -> [_ w1660]
          tunnel: w1657 -> [w1658 w1665]
          tunnel: [w1658 w1668] -> w1656
          tunnel: [w1659 w1667] -> w1655
          tunnel: w1654 -> [w1659 w1666]
          frame False {
          }
          frame True {
            w1663 = T23 {"Thread ID"=0, "Thread Flag"=FALSE}  # Thread Flag
            n552 = Bundle By Name(cluster=w1663, "Thread ID"=u16 0, "Thread Flag"=w1660) -> (w1661:T23)
            n553 = call-poly "Enqueue Message.vi"("error in (no error)"=w1666, "Message Data"=w1661, "Message"="Mérés Start", "Message Queue"=w1665) -> ("error out"=w1667:errorcluster, "dup Message Queue"=w1668:refnum<queue>)  [unwired: 6 in]
          }
        }
      }
      event "Mérés következõ": Value Change {
        n554 = event-data() -> ("NewVal"=w1669:bool)  [unwired: 1 in]
        n555 = case shown="True" w1669 {
          selector: w1669 -> [_ w1676]
          tunnel: w1673 -> [w1674 w1682]
          tunnel: [w1674 w1685] -> w1672
          tunnel: [w1675 w1684] -> w1671
          tunnel: w1670 -> [w1675 w1683]
          frame False {
          }
          frame True {
            w1680 = T23 {"Thread ID"=0, "Thread Flag"=FALSE}  # Thread Flag
            n556 = Not(x=w1676) -> (.not. x?=w1677:bool)
            n557 = Bundle By Name(cluster=w1680, "Thread ID"=u16 0, "Thread Flag"=w1677) -> (w1678:T23)
            n558 = call-poly "Enqueue Message.vi"("error in (no error)"=w1683, "Message Data"=w1678, "Message"="Mérés Következõ", "Message Queue"=w1682) -> ("error out"=w1684:errorcluster, "dup Message Queue"=w1685:refnum<queue>)  [unwired: 6 in]
          }
        }
      }
      event "Mérés stop", "Mérés stop 2": Value Change {
        n559 = event-data() -> ("NewVal"=w1686:bool)  [unwired: 1 in]
        n560 = case shown="True" w1686 {
          selector: w1686 -> [_ w1693]
          tunnel: w1690 -> [w1691 w1699]
          tunnel: [w1691 w1702] -> w1689
          tunnel: [w1692 w1701] -> w1688
          tunnel: w1687 -> [w1692 w1700]
          frame False {
          }
          frame True {
            w1697 = T23 {"Thread ID"=0, "Thread Flag"=FALSE}  # Thread Flag
            n561 = Not(x=w1693) -> (.not. x?=w1694:bool)
            n562 = Bundle By Name(cluster=w1697, "Thread ID"=u16 0, "Thread Flag"=w1694) -> (w1695:T23)
            n563 = call-poly "Enqueue Message.vi"("error in (no error)"=w1700, "Message Data"=w1695, "Message"="Mérés Vége", "Message Queue"=w1699) -> ("error out"=w1701:errorcluster, "dup Message Queue"=w1702:refnum<queue>)  [unwired: 6 in]
          }
        }
      }
      event "Végig mér": Value Change {
        w1706 = T23 {"Thread ID"=0, "Thread Flag"=FALSE}  # Thread Flag
        n564 = event-data() -> ("NewVal"=w1704:bool)  [unwired: 1 in]
        n565 = Bundle By Name(cluster=w1706, "Thread ID"=u16 0, "Thread Flag"=w1704) -> (w1703:T23)
        n566 = call-poly "Enqueue Message.vi"("error in (no error)"=w1708, "Message Data"=w1703, "Message"="Végig Mér", "Message Queue"=w1711) -> ("error out"=w1709:errorcluster, "dup Message Queue"=w1710:refnum<queue>)  [unwired: 6 in]
      }
      event "Mérés Folyamatos": Value Change {
        w1715 = T23 {"Thread ID"=0, "Thread Flag"=FALSE}  # Thread Flag
        n567 = event-data() -> ("NewVal"=w1712:bool)  [unwired: 1 in]
        n568 = Bundle By Name(cluster=w1715, "Thread ID"=u16 0, "Thread Flag"=w1712) -> (w1713:T23)
        n569 = call-poly "Enqueue Message.vi"("error in (no error)"=w1717, "Message Data"=w1713, "Message"="Mérés Lépésenként", "Message Queue"=w1720) -> ("error out"=w1718:errorcluster, "dup Message Queue"=w1719:refnum<queue>)  [unwired: 6 in]
      }
      event "Reset_Counters": Value Change {
        n570 = event-data() -> ("NewVal"=w1721:bool)  [unwired: 1 in]
        n571 = case shown="True" w1721 {
          tunnel: w1725 -> [w1727 w1735]
          tunnel: [w1727 w1734] -> w1724
          tunnel: [w1726 w1733] -> w1723
          tunnel: w1722 -> [w1726 w1732]
          frame False {
          }
          frame True {
            w1730 = T24 {"Thread ID"=0, "Callback"="", "Data"=variant, "Error"={"status"=FALSE, "code"=0, "source"=""}}  # Message
            n572 = Bundle By Name(cluster=w1730, "Thread ID"=u16 0) -> (w1728:T24)
            n573 = call-poly "Enqueue Message.vi"("error in (no error)"=w1732, "Message Data"=w1728, "Message"="Reset Result Number Variables", "Message Queue"=w1735) -> ("error out"=w1733:errorcluster, "dup Message Queue"=w1734:refnum<queue>)  [unwired: 6 in]
          }
        }
      }
      event "Reset_Counters 2": Value Change {
        n574 = event-data() -> ("NewVal"=w1736:bool)  [unwired: 1 in]
        n575 = case shown="True" w1736 {
          tunnel: w1740 -> [w1742 w1750]
          tunnel: [w1742 w1749] -> w1739
          tunnel: [w1741 w1748] -> w1738
          tunnel: w1737 -> [w1741 w1747]
          frame False {
          }
          frame True {
            w1745 = T24 {"Thread ID"=0, "Callback"="", "Data"=variant, "Error"={"status"=FALSE, "code"=0, "source"=""}}  # Message
            n576 = Bundle By Name(cluster=w1745, "Thread ID"=u16 1) -> (w1743:T24)
            n577 = call-poly "Enqueue Message.vi"("error in (no error)"=w1747, "Message Data"=w1743, "Message"="Reset Result Number Variables", "Message Queue"=w1750) -> ("error out"=w1748:errorcluster, "dup Message Queue"=w1749:refnum<queue>)  [unwired: 6 in]
          }
        }
      }
      event "Teszt vektor listbox": Value Change {
        n578 = event-data() -> ("NewVal"=w1751:i32)  [unwired: 1 in]
        n579 = local write "Etalon listbox"(w1751) -> ()
      }
      event "Etalon listbox": Value Change {
        n580 = event-data() -> ("NewVal"=w1754:i32)  [unwired: 1 in]
        n581 = local write "Teszt vektor listbox"(w1754) -> ()
      }
      event "Teszt hozzáad", "Teszt hozzáad 2": Value Change {
        n582 = event-data() -> ("NewVal"=w1758:bool)  [unwired: 1 in]
        n583 = case shown="True" w1758 {
          tunnel: w1761 -> [w1762 w1768]
          tunnel: [w1762 w1767] -> w1760
          tunnel: [w1763 w1765] -> w1759
          tunnel: w1757 -> [w1763 w1764]
          frame False {
          }
          frame True {
            n584 = call-poly "Enqueue Message.vi"("error in (no error)"=w1764, "Message"="Teszt hozzáadása", "Message Queue"=w1768) -> ("error out"=w1765:errorcluster, "dup Message Queue"=w1767:refnum<queue>)  [unwired: 7 in]
          }
        }
      }
      event "Teszt beilleszt", "Teszt beilleszt 2": Value Change {
        n585 = event-data() -> ("NewVal"=w1770:bool)  [unwired: 1 in]
        n586 = case shown="True" w1770 {
          tunnel: w1773 -> [w1774 w1780]
          tunnel: [w1774 w1779] -> w1772
          tunnel: [w1775 w1777] -> w1771
          tunnel: w1769 -> [w1775 w1776]
          frame False {
          }
          frame True {
            n587 = call-poly "Enqueue Message.vi"("error in (no error)"=w1776, "Message"="Teszt beillesztése", "Message Queue"=w1780) -> ("error out"=w1777:errorcluster, "dup Message Queue"=w1779:refnum<queue>)  [unwired: 7 in]
          }
        }
      }
      event "Teszt módosít", "Teszt módosít 2": Value Change {
        n588 = event-data() -> ("NewVal"=w1782:bool)  [unwired: 1 in]
        n589 = case shown="True" w1782 {
          tunnel: w1785 -> [w1786 w1792]
          tunnel: [w1786 w1791] -> w1784
          tunnel: [w1787 w1789] -> w1783
          tunnel: w1781 -> [w1787 w1788]
          frame False {
          }
          frame True {
            n590 = call-poly "Enqueue Message.vi"("error in (no error)"=w1788, "Message"="Teszt módosítása", "Message Queue"=w1792) -> ("error out"=w1789:errorcluster, "dup Message Queue"=w1791:refnum<queue>)  [unwired: 7 in]
          }
        }
      }
      event "Teszt töröl", "Teszt töröl 2": Value Change {
        n591 = event-data() -> ("NewVal"=w1794:bool)  [unwired: 1 in]
        n592 = case shown="True" w1794 {
          tunnel: w1797 -> [w1798 w1804]
          tunnel: [w1798 w1803] -> w1796
          tunnel: [w1799 w1801] -> w1795
          tunnel: w1793 -> [w1799 w1800]
          frame False {
          }
          frame True {
            n593 = call-poly "Enqueue Message.vi"("error in (no error)"=w1800, "Message"="Teszt törlése", "Message Queue"=w1804) -> ("error out"=w1801:errorcluster, "dup Message Queue"=w1803:refnum<queue>)  [unwired: 7 in]
          }
        }
      }
      event "Teszt másol", "Teszt másol 2": Value Change {
        n594 = event-data() -> ("NewVal"=w1805:bool)  [unwired: 1 in]
        n595 = case shown="True" w1805 {
          tunnel: w1809 -> [w1811 w1816]
          tunnel: [w1811 w1815] -> w1808
          tunnel: [w1810 w1814] -> w1807
          tunnel: w1806 -> [w1810 w1813]
          frame False {
          }
          frame True {
            n596 = call-poly "Enqueue Message.vi"("error in (no error)"=w1813, "Message"="Teszt másolása", "Message Queue"=w1816) -> ("error out"=w1814:errorcluster, "dup Message Queue"=w1815:refnum<queue>)  [unwired: 7 in]
          }
        }
      }
      event "Teszt szerkeszt", "Teszt szerkeszt 2": Value Change {
        n597 = event-data() -> ("NewVal"=w1817:bool)  [unwired: 1 in]
        n598 = case shown="True" w1817 {
          tunnel: w1821 -> [w1823 w1828]
          tunnel: [w1823 w1827] -> w1820
          tunnel: [w1822 w1826] -> w1819
          tunnel: w1818 -> [w1822 w1825]
          frame False {
          }
          frame True {
            n599 = call-poly "Enqueue Message.vi"("error in (no error)"=w1825, "Message"="Teszt szerkesztése", "Message Queue"=w1828) -> ("error out"=w1826:errorcluster, "dup Message Queue"=w1827:refnum<queue>)  [unwired: 7 in]
          }
        }
      }
      event "Teszt megnyit", "Teszt megnyit 2": Value Change {
        n600 = event-data() -> ("NewVal"=w1830:bool)  [unwired: 1 in]
        n601 = local read "Thread Num"() -> (w1829:enum16{"Mérés", "Gyûrûzés"})
        n602 = case shown="True" w1830 {
          tunnel: w1834 -> [w1835 w1845]
          tunnel: [w1835 w1844] -> w1833
          tunnel: [w1836 w1843] -> w1832
          tunnel: w1831 -> [w1836 w1842]
          tunnel: w1829 -> [_ w1837]
          frame False {
          }
          frame True {
            n603 = Bundle By Name(cluster=T15 {"Thread Num"=enum."Mérés", "Elérési út"=path ""}, "Thread Num"=w1837, "Elérési út"=path "") -> (w1838:T15)
            n604 = call-poly "Enqueue Message.vi"("error in (no error)"=w1842, "Message Data"=w1838, "Message"="Tesztszekvencia megnyitása", "Message Queue"=w1845) -> ("error out"=w1843:errorcluster, "dup Message Queue"=w1844:refnum<queue>)  [unwired: 6 in]
          }
        }
      }
      event "Teszt ment", "Teszt ment 2": Value Change {
        n605 = event-data() -> ("NewVal"=w1846:bool)  [unwired: 1 in]
        n606 = case shown="True" w1846 {
          tunnel: w1850 -> [w1851 w1857]
          tunnel: [w1851 w1856] -> w1849
          tunnel: [w1852 w1855] -> w1848
          tunnel: w1847 -> [w1852 w1854]
          frame False {
          }
          frame True {
            n607 = call-poly "Enqueue Message.vi"("error in (no error)"=w1854, "Message"="Tesztszekvencia mentése", "Message Queue"=w1857) -> ("error out"=w1855:errorcluster, "dup Message Queue"=w1856:refnum<queue>)  [unwired: 7 in]
          }
        }
      }
      event "Teszt eltávolít", "Teszt eltávolít 2": Value Change {
        n608 = event-data() -> ("NewVal"=w1858:bool)  [unwired: 1 in]
        n609 = case shown="True" w1858 {
          tunnel: w1862 -> [w1863 w1869]
          tunnel: [w1863 w1868] -> w1861
          tunnel: [w1864 w1867] -> w1860
          tunnel: w1859 -> [w1864 w1866]
          frame False {
          }
          frame True {
            n610 = call-poly "Enqueue Message.vi"("error in (no error)"=w1866, "Message"="Tesztszekvencia eltávolítása", "Message Queue"=w1869) -> ("error out"=w1867:errorcluster, "dup Message Queue"=w1868:refnum<queue>)  [unwired: 7 in]
          }
        }
      }
      event "Thread 0", "Thread 0_2": Value Change {
        n611 = event-data() -> ("NewVal"=w1870:bool)  [unwired: 1 in]
        n612 = case shown="True" w1870 {
          tunnel: w1874 -> [w1875 w1881]
          tunnel: [w1875 w1880] -> w1873
          tunnel: [w1876 w1879] -> w1872
          tunnel: w1871 -> [w1876 w1878]
          frame False {
          }
          frame True {
            n613 = call-poly "Enqueue Message.vi"("error in (no error)"=w1878, "Message"="Teszt váltás Mérés", "Message Queue"=w1881) -> ("error out"=w1879:errorcluster, "dup Message Queue"=w1880:refnum<queue>)  [unwired: 7 in]
          }
        }
      }
      event "Thread 1", "Thread 1_2": Value Change {
        n614 = event-data() -> ("NewVal"=w1882:bool)  [unwired: 1 in]
        n615 = case shown="True" w1882 {
          tunnel: w1886 -> [w1887 w1892]
          tunnel: [w1887 w1891] -> w1885
          tunnel: [w1888 w1890] -> w1884
          tunnel: w1883 -> [w1888 w1889]
          frame False {
          }
          frame True {
            n616 = disable-structure shown="Disabled" {
              disable-tunnel: w1892 -> [w1897 w1899]
              disable-tunnel: [w1896 w1899] -> w1891
              disable-tunnel: [w1895 w1898] -> w1890
              disable-tunnel: w1889 -> [w1894 w1898]
              frame Disabled {
                n617 = call-poly "Enqueue Message.vi"("error in (no error)"=w1894, "Message"="Teszt váltás Gyûrûzés", "Message Queue"=w1897) -> ("error out"=w1895:errorcluster, "dup Message Queue"=w1896:refnum<queue>)  [unwired: 7 in]
              }
              frame Enabled {
              }
            }
          }
        }
      }
      event "Keyence Open": Value Change {
        n618 = event-data() -> ("NewVal"=w1901:bool)  [unwired: 1 in]
        n619 = call-poly "Enqueue Message.vi"("error in (no error)"=w1902, "Message Data"=w1901, "Message"="KEYENCE Open Connection", "Message Queue"=w1905) -> ("error out"=w1903:errorcluster, "dup Message Queue"=w1904:refnum<queue>)  [unwired: 6 in]
      }
      event "Start marking": Value Change {
        n620 = event-data() -> ("NewVal"=w1906:bool)  [unwired: 1 in]
        n621 = case shown="True" w1906 {
          tunnel: w1910 -> [w1912 w1917]
          tunnel: [w1912 w1916] -> w1909
          tunnel: [w1911 w1915] -> w1908
          tunnel: w1907 -> [w1911 w1914]
          frame False {
          }
          frame True {
            n622 = call-poly "Enqueue Message.vi"("error in (no error)"=w1914, "Message"="KEYENCE Marking", "Message Queue"=w1917) -> ("error out"=w1915:errorcluster, "dup Message Queue"=w1916:refnum<queue>)  [unwired: 7 in]
          }
        }
      }
      event "Program change": Value Change {
        n623 = event-data() -> ("NewVal"=w1918:bool)  [unwired: 1 in, 5 out]
        n624 = case shown="True" w1918 {
          tunnel: w1923 -> [w1925 w1931]
          tunnel: [w1925 w1930] -> w1922
          tunnel: [w1924 w1929] -> w1921
          tunnel: w1920 -> [w1924 w1928]
          tunnel: "Program No" -> [_ w1926]
          frame False {
          }
          frame True {
            n625 = call-poly "Enqueue Message.vi"("error in (no error)"=w1928, "Message Data"=w1926, "Message"="KEYENCE Program Change", "Message Queue"=w1931) -> ("error out"=w1929:errorcluster, "dup Message Queue"=w1930:refnum<queue>)  [unwired: 6 in]
          }
        }
      }
      event "Error clear": Value Change {
        n626 = event-data() -> ("NewVal"=w1932:bool)  [unwired: 1 in]
        n627 = case shown="True" w1932 {
          tunnel: w1936 -> [w1938 w1943]
          tunnel: [w1938 w1942] -> w1935
          tunnel: [w1937 w1941] -> w1934
          tunnel: w1933 -> [w1937 w1940]
          frame False {
          }
          frame True {
            n628 = call-poly "Enqueue Message.vi"("error in (no error)"=w1940, "Message"="KEYENCE Error Clear", "Message Queue"=w1943) -> ("error out"=w1941:errorcluster, "dup Message Queue"=w1942:refnum<queue>)  [unwired: 7 in]
          }
        }
      }
      event "Update Sys Time": Value Change {
        n629 = event-data() -> ("NewVal"=w1944:bool)  [unwired: 1 in]
        n630 = case shown="True" w1944 {
          tunnel: w1948 -> [w1950 w1955]
          tunnel: [w1950 w1954] -> w1947
          tunnel: [w1949 w1953] -> w1946
          tunnel: w1945 -> [w1949 w1952]
          frame False {
          }
          frame True {
            n631 = call-poly "Enqueue Message.vi"("error in (no error)"=w1952, "Message"="KEYENCE Update Sys Time", "Message Queue"=w1955) -> ("error out"=w1953:errorcluster, "dup Message Queue"=w1954:refnum<queue>)  [unwired: 7 in]
          }
        }
      }
      event "Termék ment": Value Change {
        n632 = event-data() -> ("NewVal"=w1956:bool)  [unwired: 1 in]
        n633 = case shown="True" w1956 {
          tunnel: w1960 -> [w1961 w1967]
          tunnel: [w1961 w1966] -> w1959
          tunnel: [w1962 w1964] -> w1958
          tunnel: w1957 -> [w1962 w1963]
          frame False {
          }
          frame True {
            n634 = call-poly "Enqueue Message.vi"("error in (no error)"=w1963, "Message"="Termék mentése", "Message Queue"=w1967) -> ("error out"=w1964:errorcluster, "dup Message Queue"=w1966:refnum<queue>)  [unwired: 7 in]
          }
        }
      }
      event "Keyence Disable": Value Change {
        n635 = event-data() -> ("NewVal"=w1968:bool)  [unwired: 1 in]
        n636 = call-poly "Enqueue Message.vi"("error in (no error)"=w1970, "Message Data"=w1968, "Message"="KEYENCE Laser Disable", "Message Queue"=w1973) -> ("error out"=w1971:errorcluster, "dup Message Queue"=w1972:refnum<queue>)  [unwired: 6 in]
      }
      event "Etalon mérés": Value Change {
        n637 = event-data() -> ("NewVal"=w1974:bool)  [unwired: 1 in]
        n638 = call-poly "Enqueue Message.vi"("error in (no error)"=w1978, "Message Data"=w1974, "Message"="Etalon mérés", "Message Queue"=w1979) -> ("error out"=w1977:errorcluster, "dup Message Queue"=w1976:refnum<queue>)  [unwired: 6 in]
      }
      event "Új felhasználó": Value Change {
        n639 = event-data() -> ("NewVal"=w1981:bool)  [unwired: 1 in]
        n640 = case shown="True" w1981 {
          tunnel: w1984 -> [w1985 w1989]
          tunnel: [w1985 w1995] -> w1983
          tunnel: [w1986 w1993] -> w1982
          tunnel: w1980 -> [w1986 w1990]
          frame False {
          }
          frame True {
            n641 = call-poly "Enqueue Message.vi"("error in (no error)"=w1990, "Message Data"="Új felhasználó" ("Message"), "Message"="Set Statusbar", "Message Queue"=w1989) -> ("error out"=w1991:errorcluster, "dup Message Queue"=w1987:refnum<queue>)  [unwired: 6 in]
            n642 = call-poly "Enqueue Message.vi"("error in (no error)"=w1991, "Message"="Új felhasználó", "Message Queue"=w1987) -> ("error out"=w1993:errorcluster, "dup Message Queue"=w1995:refnum<queue>)  [unwired: 7 in]
          }
        }
      }
      event "Felhasználó törlése": Value Change {
        n643 = event-data() -> ("NewVal"=w1996:bool)  [unwired: 1 in]
        n644 = case shown="True" w1996 {
          tunnel: w2000 -> [w2001 w2004]
          tunnel: [w2001 w2011] -> w1999
          tunnel: [w2002 w2009] -> w1998
          tunnel: w1997 -> [w2002 w2005]
          frame False {
          }
          frame True {
            n645 = call-poly "Enqueue Message.vi"("error in (no error)"=w2005, "Message Data"="Felhasználó törlése" ("Message"), "Message"="Set Statusbar", "Message Queue"=w2004) -> ("error out"=w2006:errorcluster, "dup Message Queue"=w2003:refnum<queue>)  [unwired: 6 in]
            n646 = call-poly "Enqueue Message.vi"("error in (no error)"=w2006, "Message"="Felhasználó törlése", "Message Queue"=w2003) -> ("error out"=w2009:errorcluster, "dup Message Queue"=w2011:refnum<queue>)  [unwired: 7 in]
          }
        }
      }
      event "Felhasználó módosítás": Value Change {
        n647 = event-data() -> ("NewVal"=w2013:bool)  [unwired: 1 in]
        n648 = case shown="True" w2013 {
          tunnel: w2016 -> [w2017 w2020]
          tunnel: [w2017 w2027] -> w2015
          tunnel: [w2018 w2025] -> w2014
          tunnel: w2012 -> [w2018 w2021]
          frame False {
          }
          frame True {
            n649 = call-poly "Enqueue Message.vi"("error in (no error)"=w2021, "Message Data"="Felhasználó módosítása" ("Message"), "Message"="Set Statusbar", "Message Queue"=w2020) -> ("error out"=w2022:errorcluster, "dup Message Queue"=w2019:refnum<queue>)  [unwired: 6 in]
            n650 = call-poly "Enqueue Message.vi"("error in (no error)"=w2022, "Message"="Felhasználó módosítása", "Message Queue"=w2019) -> ("error out"=w2025:errorcluster, "dup Message Queue"=w2027:refnum<queue>)  [unwired: 7 in]
          }
        }
      }
      event "Felhasználók mentés": Value Change {
        n651 = event-data() -> ("NewVal"=w2029:bool)  [unwired: 1 in]
        n652 = case shown="True" w2029 {
          tunnel: w2032 -> [w2033 w2036]
          tunnel: [w2033 w2043] -> w2031
          tunnel: [w2034 w2041] -> w2030
          tunnel: w2028 -> [w2034 w2037]
          frame False {
          }
          frame True {
            n653 = call-poly "Enqueue Message.vi"("error in (no error)"=w2037, "Message Data"="Mentés" ("Message"), "Message"="Set Statusbar", "Message Queue"=w2036) -> ("error out"=w2038:errorcluster, "dup Message Queue"=w2035:refnum<queue>)  [unwired: 6 in]
            n654 = call-poly "Enqueue Message.vi"("error in (no error)"=w2038, "Message"="Felhasználó mentés", "Message Queue"=w2035) -> ("error out"=w2041:errorcluster, "dup Message Queue"=w2043:refnum<queue>)  [unwired: 7 in]
          }
        }
      }
      event Panel Close? {
        n655 = event-data() -> ()  [unwired: 1 in, 1 out]
        n656 = call-poly "Enqueue Message.vi"("Priority Message? (F)"=TRUE, "Message"="Confirm Quit", "Message Queue"=w2048) -> ("error out"=w2047:errorcluster, "dup Message Queue"=w2046:refnum<queue>)  [unwired: 7 in]
        n657 = event-data("Discard?"=TRUE) -> ()  [unwired: 1 in, 1 out]
      }
      event Application Instance Close {
        # "#CodeRecommended - When a project closes, all VIs within that project are aborted and leave memory. However, any code placed in this event frame is guaranteed to run to completion, so add any cleanup code that absolutely must happen here."
        n658 = event-data() -> ()  [unwired: 1 in, 1 out]
      }
      event User Event {
        n659 = event-data() -> ()  [unwired: 1 in, 4 out]
        n660 = flat-sequence {
          tunnel: w2052 -> [w2055]
          tunnel: [w2055] -> w2051
          frame #0 {
          }
        }
      }
      event "Tab Control": Value Change {
        n661 = event-data() -> ("CtlRef"=w2069:refnum<vi>, "NewVal"=w2061:T1, "OldVal"=w2067:T1)  [unwired: 1 in, 1 out]
        n662 = property class="TabCtl (strict)"(reference=w2069, error in=w2063) -> (error out=w2058:errorcluster, "Pages"=w2068:refnum<vi>[])  [unwired: 1 out]
        n663 = Index Array(array=w2068, index #1=w2061, index #2=w2067) -> (element #1=w2062:refnum<vi>, element #2=w2072:refnum<vi>)
        n664 = call-poly "Enqueue Message.vi"("error in (no error)"=w2058, "Message"="Update Controls", "Message Queue"=w2060) -> ("error out"=w2057:errorcluster, "dup Message Queue"=w2059:refnum<queue>)  [unwired: 7 in]
        n665 = property class="Page"(reference=w2062, error in=w2057, "FG Color"=u32 13816530) -> (error out=w2065:errorcluster)  [unwired: 1 out]
        n666 = property class="Page"(reference=w2072, error in=w2057, "FG Color"=u32 11842740) -> (error out=w2066:errorcluster)  [unwired: 1 out]
        n667 = Merge Errors(w2065, w2066) -> (w2064:errorcluster)
      }
      event Value Change {
        n668 = event-data() -> ()  [unwired: 1 in, 6 out]
        n669 = call-poly "Enqueue Message.vi"("error in (no error)"=w2076, "Message Data"="Digital Out", "Message"="OUTPUT PortWrite", "Message Queue"=w2078) -> ("error out"=w2075:errorcluster, "dup Message Queue"=w2077:refnum<queue>)  [unwired: 6 in]
      }
      event Value Change {
        n670 = event-data() -> ()  [unwired: 1 in, 6 out]
        n671 = Unbundle By Name("NI Analog Output") -> ("NI-6221.UCTRL"=w2081:dbl)
        n672 = Bundle(cluster=cluster{i32, "UCtrl":dbl} {0, "UCtrl"=0.0}, Enum_AO."UCTRL" ("Enum"), "UCtrl"=w2081) -> (w2079:cluster{i32, "UCtrl":dbl})
        n673 = call-poly "Enqueue Message.vi"("error in (no error)"=w2086, "Message Data"=w2079, "Message"="OUTPUT Analog Write", "Message Queue"=w2088) -> ("error out"=w2085:errorcluster, "dup Message Queue"=w2087:refnum<queue>)  [unwired: 6 in]
      }
      event "Setup UCTRL NTC": Value Change {
        n674 = event-data() -> ("NewVal"=w2093:bool)  [unwired: 1 in, 5 out]
        n675 = case shown="True" w2093 {
          tunnel: w2094 -> [_ w2114]
          tunnel: w2092 -> [w2096 w2105]
          tunnel: [w2096 w2104] -> w2091
          tunnel: w2090 -> [w2095 w2103]
          tunnel: [w2095 w2100] -> w2089
          frame False {
          }
          frame True {
            w2111 = T27 {"Dummy"=FALSE, "R Res"=0.0, "NTC Res"=0.0, "Insulation Res"=0.0, "Temperature"=0.0, "NTC Exp Res"=0.0, "NTC Calc Temp"=0.0, "Delta U Puffer"=refnum, "I Adj Parameters"={"Vr NTC"=0.0, "Vr R"=0.0, "Vr dU"=0.0, "I Adj step"=0, "Output"=0.0, "Adj Failed"=FALSE}, "UCTRL Cluster"={"UCTRL NTC"=0.0, "UCTRL R"=0.0, "UCTRL dU"=0.0}}  # Data Processor Data Cluster
            n676 = Unbundle By Name(w2114) -> ("Data Processor data"=w2113:refnum<queue>)
            n677 = call "Preview Message.vi"("error in (no error)"=w2103, "Message Queue"=w2113) -> ("error out"=w2102:errorcluster, "Message Data"=w2112:variant)  [unwired: 5 in, 3 out]
            n678 = Variant To Data(error in=w2102, type=w2111, Variant=w2112) -> (data=w2110:T27, error out=w2101:errorcluster)
            n679 = Unbundle By Name(w2110) -> ("UCTRL Cluster.UCTRL NTC"=w2097:dbl)
            n680 = local read "NI Analog Output"() -> (w2099:T7)
            n681 = Bundle(cluster=cluster{i32, "UCtrl":dbl} {0, "UCtrl"=0.0}, Enum_AO."UCTRL" ("Enum"), "UCtrl"=w2097) -> (w2109:cluster{i32, "UCtrl":dbl})
            n682 = Bundle By Name(cluster=w2099, "NI-6221.UCTRL"=w2097) -> (w2098:T7)
            n683 = local write "NI Analog Output"(w2098) -> ()
            n684 = call-poly "Enqueue Message.vi"("error in (no error)"=w2101, "Message Data"=w2109, "Message"="OUTPUT Analog Write", "Message Queue"=w2105) -> ("error out"=w2100:errorcluster, "dup Message Queue"=w2104:refnum<queue>)  [unwired: 6 in]
          }
        }
      }
      event "Setup UCTRL R": Value Change {
        n685 = event-data() -> ("NewVal"=w2119:bool)  [unwired: 1 in, 5 out]
        n686 = case shown="True" w2119 {
          tunnel: w2120 -> [_ w2140]
          tunnel: w2118 -> [w2122 w2131]
          tunnel: [w2122 w2130] -> w2117
          tunnel: w2116 -> [w2121 w2129]
          tunnel: [w2121 w2126] -> w2115
          frame False {
          }
          frame True {
            w2137 = T27 {"Dummy"=FALSE, "R Res"=0.0, "NTC Res"=0.0, "Insulation Res"=0.0, "Temperature"=0.0, "NTC Exp Res"=0.0, "NTC Calc Temp"=0.0, "Delta U Puffer"=refnum, "I Adj Parameters"={"Vr NTC"=0.0, "Vr R"=0.0, "Vr dU"=0.0, "I Adj step"=0, "Output"=0.0, "Adj Failed"=FALSE}, "UCTRL Cluster"={"UCTRL NTC"=0.0, "UCTRL R"=0.0, "UCTRL dU"=0.0}}  # Data Processor Data Cluster
            n687 = Unbundle By Name(w2140) -> ("Data Processor data"=w2139:refnum<queue>)
            n688 = call "Preview Message.vi"("error in (no error)"=w2129, "Message Queue"=w2139) -> ("error out"=w2128:errorcluster, "Message Data"=w2138:variant)  [unwired: 5 in, 3 out]
            n689 = Variant To Data(error in=w2128, type=w2137, Variant=w2138) -> (data=w2136:T27, error out=w2127:errorcluster)
            n690 = Unbundle By Name(w2136) -> ("UCTRL Cluster.UCTRL R"=w2123:dbl)
            n691 = local read "NI Analog Output"() -> (w2125:T7)
            n692 = Bundle(cluster=cluster{i32, "UCtrl":dbl} {0, "UCtrl"=0.0}, Enum_AO."UCTRL" ("Enum"), "UCtrl"=w2123) -> (w2135:cluster{i32, "UCtrl":dbl})
            n693 = Bundle By Name(cluster=w2125, "NI-6221.UCTRL"=w2123) -> (w2124:T7)
            n694 = local write "NI Analog Output"(w2124) -> ()
            n695 = call-poly "Enqueue Message.vi"("error in (no error)"=w2127, "Message Data"=w2135, "Message"="OUTPUT Analog Write", "Message Queue"=w2131) -> ("error out"=w2126:errorcluster, "dup Message Queue"=w2130:refnum<queue>)  [unwired: 6 in]
          }
        }
      }
      event "Tab control debug": Value Change {
        n696 = event-data() -> ("CtlRef"=w2157:refnum<vi>, "NewVal"=w2142:enum32{"Digital IO", "Analog IO", "Laser"}, "OldVal"=w2154:enum32{"Digital IO", "Analog IO", "Laser"})  [unwired: 1 in, 1 out]
        n697 = property class="TabCtl (strict)"(reference=w2157, error in=w2156) -> (error out=w2144:errorcluster, "Pages"=w2153:refnum<vi>[])  [unwired: 1 out]
        n698 = Index Array(array=w2153, index #1=w2142, index #2=w2154) -> (element #1=w2152:refnum<vi>, element #2=w2151:refnum<vi>)
        n699 = call-poly "Enqueue Message.vi"("error in (no error)"=w2144, "Message"="Update Controls", "Message Queue"=w2146) -> ("error out"=w2143:errorcluster, "dup Message Queue"=w2145:refnum<queue>)  [unwired: 7 in]
        n700 = property class="Page"(reference=w2152, error in=w2143, "FG Color"=u32 13816530) -> (error out=w2147:errorcluster)  [unwired: 1 out]
        n701 = property class="Page"(reference=w2151, error in=w2143, "FG Color"=u32 11842740) -> (error out=w2148:errorcluster)  [unwired: 1 out]
        n702 = Merge Errors(w2147, w2148) -> (w2155:errorcluster)
      }
    }
    n703 = call "Error Handler - Event Handling Loop.vi"("error in (no error)"=w1584, "Message Queue"=w1582) -> ("dup error in"=w1581:errorcluster)  [unwired: 8 in, 1 out]
  }
  n704 = call "Keyence handler.vi"("error in (no error)"=w3, "Message Queues out"=w1) -> ("error out"=w14:errorcluster)  [unwired: 8 in, 1 out]
  n705 = call "NI Digital.vi"("error in (no error)"=w3, "Message Queues"=w1) -> ("error out"=w43:errorcluster)  [unwired: 8 in, 1 out]
  n706 = call "NI Analog.vi"("error in (no error)"=w3, "Message Queues"=w1) -> ("error out"=w4:errorcluster)  [unwired: 8 in, 1 out]
  n707 = call "Timer mérés.vi"("error in (no error)"=w3, "Message Queues in"=w1) -> ("error out"=w29:errorcluster)  [unwired: 8 in, 1 out]
  n708 = call "Timer laser.vi"("error in (no error)"=w3, "Message Queues in"=w1) -> ("error out"=w22:errorcluster)  [unwired: 8 in, 1 out]
  n709 = call <vilib>:"Clear Errors.vi"("error in (no error)"=w22) -> ("error out"=w25:errorcluster)  [unwired: 5 in, 1 out]
  n710 = call <vilib>:"Clear Errors.vi"("error in (no error)"=w11) -> ("error out"=w8:errorcluster)  [unwired: 5 in, 1 out]
  n711 = call <vilib>:"Clear Errors.vi"("error in (no error)"=w21) -> ("error out"=w18:errorcluster)  [unwired: 5 in, 1 out]
  n712 = call <vilib>:"Clear Errors.vi"("error in (no error)"=w29) -> ("error out"=w26:errorcluster)  [unwired: 5 in, 1 out]
  n713 = call <vilib>:"Clear Errors.vi"("error in (no error)"=w36) -> ("error out"=w35:errorcluster)  [unwired: 5 in, 1 out]
  n714 = call <vilib>:"Clear Errors.vi"("error in (no error)"=w49) -> ("error out"=w48:errorcluster)  [unwired: 5 in, 1 out]
  n715 = call <vilib>:"Clear Errors.vi"("error in (no error)"=w14) -> ("error out"=w17:errorcluster)  [unwired: 5 in, 1 out]
  n716 = call <vilib>:"Clear Errors.vi"("error in (no error)"=w32) -> ("error out"=w31:errorcluster)  [unwired: 5 in, 1 out]
  n717 = call <vilib>:"Clear Errors.vi"("error in (no error)"=w46) -> ("error out"=w45:errorcluster)  [unwired: 5 in, 1 out]
  n718 = call <vilib>:"Clear Errors.vi"("error in (no error)"=w43) -> ("error out"=w41:errorcluster)  [unwired: 5 in, 1 out]
  n719 = call <vilib>:"Clear Errors.vi"("error in (no error)"=w4) -> ("error out"=w6:errorcluster)  [unwired: 5 in, 1 out]
  n720 = Unbundle By Name(w1) -> ("UI"=w2:refnum<queue>)
  n721 = call-poly "Enqueue Message.vi"("Priority Message? (F)"=TRUE, "error in (no error)"=w25, "Message"="Timer laser Stopped", "Message Queue"=w2) -> ()  [unwired: 6 in, 2 out]
  n722 = call-poly "Enqueue Message.vi"("Priority Message? (F)"=TRUE, "error in (no error)"=w35, "Message"="DAQ Stopped", "Message Queue"=w2) -> ()  [unwired: 6 in, 2 out]
  n723 = call-poly "Enqueue Message.vi"("Priority Message? (F)"=TRUE, "error in (no error)"=w26, "Message"="Timer mérés Stopped", "Message Queue"=w2) -> ()  [unwired: 6 in, 2 out]
  n724 = call-poly "Enqueue Message.vi"("Priority Message? (F)"=TRUE, "error in (no error)"=w41, "Message"="NI Digital Stopped", "Message Queue"=w2) -> ()  [unwired: 6 in, 2 out]
  n725 = call-poly "Enqueue Message.vi"("Priority Message? (F)"=TRUE, "error in (no error)"=w6, "Message"="NI Analog Stopped", "Message Queue"=w2) -> ()  [unwired: 6 in, 2 out]
  n726 = call-poly "Enqueue Message.vi"("Priority Message? (F)"=TRUE, "error in (no error)"=w48, "Message"="Engine Stopped", "Message Queue"=w2) -> ()  [unwired: 6 in, 2 out]
  n727 = call-poly "Enqueue Message.vi"("Priority Message? (F)"=TRUE, "error in (no error)"=w31, "Message"="Data Processor Stopped", "Message Queue"=w2) -> ()  [unwired: 6 in, 2 out]
  n728 = call-poly "Enqueue Message.vi"("Priority Message? (F)"=TRUE, "error in (no error)"=w45, "Message"="Timers Stopped", "Message Queue"=w2) -> ()  [unwired: 6 in, 2 out]
  n729 = call-poly "Enqueue Message.vi"("Priority Message? (F)"=TRUE, "error in (no error)"=w8, "Message"="Ring Stopped", "Message Queue"=w2) -> ()  [unwired: 6 in, 2 out]
  n730 = call-poly "Enqueue Message.vi"("Priority Message? (F)"=TRUE, "error in (no error)"=w18, "Message"="Laser Stopped", "Message Queue"=w2) -> ()  [unwired: 6 in, 2 out]
  n731 = call-poly "Enqueue Message.vi"("Priority Message? (F)"=TRUE, "error in (no error)"=w17, "Message"="Keyence Stopped", "Message Queue"=w2) -> ()  [unwired: 6 in, 2 out]
  n732 = Unregister For Events(event registration refnum=w53, error in=w52) -> (error out=w54:errorcluster)
  n733 = Merge Errors(w54, w57) -> (w55:errorcluster)
  n734 = call "Destroy User Event - Stop.vi"("error in (no error)"=w55, "User Event - Stop"=w13) -> ("error out"=w44:errorcluster)  [unwired: 9 in]
  n735 = disable-structure shown="Enabled" {
    disable-tunnel: w44 -> [w2158 _]
    frame Disabled {
      n736 = flat-sequence {
        tunnel: w2158 -> [_]
        frame #0 {
          n737 = property on="Tab Control" class="TabCtl (strict)"() -> ("Pages"=w2162:refnum<vi>[])  [unwired: 2 in, 2 out]
          n738 = for {
            tunnel: w2162 -> [w2166] mode=indexing
            tunnel: [w2163] -> w2161 mode=indexing
            n739 = property class="Page"(reference=w2166) -> ("Page Enabled State"=w2165:T31)  [unwired: 1 in, 2 out]
            n740 = Equal?(x=w2165, y=T31."Page Enabled") -> (x = y?=w2163:bool)
          }
          n741 = And Array Elements(Boolean array=w2161) -> (logical AND=w2160:bool)
          n742 = Not(x=w2160) -> (.not. x?=w2159:bool)
          n743 = Quit LabVIEW(quit? (T)=w2159) -> ()
        }
      }
    }
    frame Enabled {
    }
  }
